vi "myRIO_BRig_RT_v0,41.vi"() -> ()   [LabVIEW 2014]
uses:
  myRIO_BRig_RT__Case_Exp_stateList.ctl
  myRIO_BRig_RT__Case_NonExp_stateList.ctl
  <vilib>/Platform/TimedLoop/XDataNode/timing_clust.ctl
  <vilib>/Platform/TimedLoop/XDataNode/nitl_modes.ctl
  <vilib>/Platform/TimedLoop/XDataNode/wakeup.ctl
  <vilib>/WebDAVClient/Advanced/SessionHandle.ctl
  <vilib>/myRIO/Common/Instrument Driver Framework/myRIO v1.0/UART/vis/myRIO v1.0 Close UART.vi
  <vilib>/FPGAPlugInAG/myRIO-1900/niLvFpga_Open_myRIO-1900.vi
  <vilib>/rvi/interface/common/dynamic/niFpgaDynamicAddResources.vi
  <vilib>/Utility/error.llb/Error Cluster From Error Code.vi
  <vilib>/rvi/errors/niLvFpgaAdjustHostInterfaceError.vi
  <vilib>/FPGAPlugInAG/Dynamic/niLvFpga_Close_Dynamic.vi
  <vilib>/myRIO/Common/Instrument Driver Framework/Utilities/vis/FPGA Ref Manager.vi
  <vilib>/myRIO/Common/Instrument Driver Framework/myRIO v1.0/myRIO v1.0 Reset FPGA.vi
  <vilib>/myRIO/Common/Instrument Driver Framework/myRIO v1.0/IRQ/vis/myRIO v1.0 IRQ Info FGV.vi
  <vilib>/myRIO/Common/Instrument Driver Framework/myRIO v1.0/IRQ/vis/myRIO v1.0 Timer IRQ Info FGV.vi
  <vilib>/myRIO/Common/Instrument Driver Framework/myRIO v1.0/IRQ/vis/myRIO v1.0 ISR Agent.vi
  <vilib>/rvi/interface/nirviOpenFPGA/nirviOpenFPGA.xnode
  myRIO_BRig_FPGA_v3,2__PortC__build.lvbitx
  myRIO_BRig_FPGA_v3,2__PortC.vi
  <vilib>/rvi/interface/nirviReadWriteControl/nirviReadWriteControl.xnode
  <vilib>/Platform/TimedLoop/XDataNode/XDataNode.xnode
  <vilib>/rvi/interface/nirviCloseFPGA/nirviCloseFPGA.xnode
  <vilib>/Platform/TimedLoop/XDataNode/XDNodeRunTimeDep.lvlib
  <vilib>/rvi/interface/Simulation/niFpgaSimulationCallBeginRW.vi
  <vilib>/myRIO/Instrument Drivers/Utilities/Utilities.lvlib
  <vilib>/WebDAVClient/NI_WebDAV.lvlib
  NiFpgaLv.dll
panel:
  in  "AO0":i16 min=-2047 max=2047 step=1
  in  "laser_Nvalley":u32
  in  "laser_Npeak":u32
  in  "LC_Cue1_All_Count":u16
  in  "LC_Cue1_First_Count":u16
  in  "LC_Cue1_All_delayOpt":bool
  in  "LC_ENL1_All_delayOpt":bool
  in  "LC_ENL1_All_Count":u16
  in  "LC_ENL1_First_Count":u16
  in  "LC_Cue1_First_delayOpt":bool
  in  "LC_ENL1_First_delayOpt":bool
  in  "Tcycle_Cue_max":u16=1000 caption="Max [ms]" min=5 max=5000 step=5
  in  "Tcycle_Cue_min":u16=1000 caption="Min [ms]" min=5 max=5000 step=5
  in  "SendData":bool
  out "cSpout":enum16{"Left", "Right"}(ring) caption="Left or Right Spout"
  out "A4":u32 caption="LickCounter_Right"
  out "A2":u32 caption="LickCounter_Left"
  in  "tDelay_laser_wro":u32
  in  "tCycle_laser_wro":u32=1000
  in  "tDelay_laser_rew":u32
  in  "laserResponse_wrong_LED":bool
  out "error_initTrial":errorcluster
  out "error_Selection_pre":errorcluster
  out "error_Selection":errorcluster
  in  "tCycle_laser_rew":u32=1000
  out "SelectWrong":bool
  out "SelectReward":bool
  in  "Left(F)_or_Right(T)":bool
  in  "ignoreWrong":bool
  in  "SelectionState":bool
  in  "laserResponse_wrong":bool
  in  "laserResponse_reward":bool
  in  "laserResponse_reward_LED":bool
  out "nRewards_Right":u16 caption="# Rewards Total (Right)"
  out "nRewards_Left":u16 caption="# Rewards Total (Left)"
  out "nRewards_cur":u16 caption="# Rewards in Current Block"
  out "TpB_target":u16 caption="Target Trials Per Block"
  out "cState_NonExp":T1 caption="NonExperimental State"
  out "iBlock":u16 caption="Current Block"
  out "cState":T2 caption="Experimental State"
  out "iTrial":u16 caption="Current Trial"
  in  "warmupType":bool
  in  "TestConnection":bool
  in  "warmup":bool caption="WarmUp"
  in  "Host Filename Prefix":string="Exp1_TM2"
  out "Connected To Host?":bool
  in  "Host Password":string="sabalab"
  in  "Host UserName":string="Test2"
  in  "sp_RightSpout":u16(slide)=2 max=2 step=1 scale=0.0..2.0
  in  "sp_LeftSpout":u16(slide)=2 max=2 step=1 scale=0.0..2.0
  in  "BUR_max":u16 caption="Count Reward Structure  (0 = off)"
  in  "LC_Wrong_Probability":u16
  in  "LC_Wrong_Trial":u16(slide) max=2 step=1 scale=0.0..2.0
  in  "LC_Wrong_Block":u16(slide) max=2 step=1 scale=0.0..2.0
  in  "LC_Wrong_OnOff":bool
  in  "LC_Reward_Probability":u16
  in  "LC_Reward_Trial":u16(slide) max=2 step=1 scale=0.0..2.0
  in  "LC_Reward_Block":u16(slide) max=2 step=1 scale=0.0..2.0
  in  "LC_Reward_OnOff":bool
  in  "LC_Cue1_All_Probability":u16
  in  "LC_Cue1_All_Block":u16(slide) max=2 step=1 scale=0.0..2.0
  in  "LC_Cue1_All_OnOff":bool
  in  "LC_Cue1_First_Probability":u16
  in  "LC_Cue1_First_Block":u16(slide) max=2 step=1 scale=0.0..2.0
  in  "LC_Cue1_First_OnOff":bool
  in  "LC_ENL1_All_Probability":u16 max=100 step=1
  in  "LC_ENL1_All_Block":u16(slide) max=2 step=1 scale=0.0..2.0
  in  "LC_ENL1_All_OnOff":bool
  in  "LC_ENL1_First_Probability":u16 max=100 step=1
  in  "LC_ENL1_First_Block":u16(slide) max=2 step=1 scale=0.0..2.0
  in  "A6":bool caption="Activate Recording?\n(Select Prior to\nStarting Experiment)"
  in  "Tcycle_Timeout":u16=1000 caption="Timeout Time [ms]" min=10 max=10000 step=1
  in  "Tcycle_Wrong":u16=1000 caption="Wrong Time [ms]" min=10 max=10000 step=1
  in  "Tcycle_Selection":u16=1000 caption="Answer Time [ms]" min=1 max=10000 step=1
  in  "Tcycle_RewardPost":u16=1000 caption="Consumption Time [ms]" min=250 max=10000 step=250
  in  "Tcycle_Reward_L":u16=500 caption="Reward Time [ms]" min=1 max=1000 step=1
  in  "Tcycle_Reward_R":u16=500 caption="Reward Time [ms]" min=1 max=1000 step=1
  in  "TpB_Max_R":u16=4 caption="Max TrialsPerBlock" min=1 max=12 step=1
  in  "TpB_Min_R":u16=4 caption="Min TrialsPerBlock" min=1 max=12 step=1
  in  "TpB_Max_L":u16=4 caption="Max TrialsPerBlock" min=1 max=12 step=1
  in  "TpB_Min_L":u16=4 caption="Min TrialsPerBlock" min=1 max=12 step=1
  in  "BUR_min":u16 caption="Count Reward Structure  (0 = off)"
  in  "TrialUntilReward":bool caption="Ignore Wrong \nSelection"
  in  "CueCycles":u16=1 caption="Cue Structure" min=1 max=1 step=1
  in  "MTrig_Laser_Tcycle":u16=10 caption="Time [ms]"
  in  "MTrig_Laser_trig":bool
  in  "MTrig_Audio_trig__R":bool caption="Trigger Audio"
  in  "MTrig_Audio_trig__L":bool caption="Trigger Audio"
  in  "RewCalib_Trig_R":bool caption="Calibrate_R"
  in  "RewCalib_Trig_L":bool caption="Calibrate_L"
  in  "MTrig_Solenoid_Tcycle__R":u16=300 caption="Time [ms]"
  in  "MTrig_Solenoid_Tcycle__L":u16=300 caption="Time [ms]"
  in  "MTrig_Solenoid_trig__R":bool caption="Solenoid"
  in  "MTrig_Solenoid_trig__L":bool caption="Solenoid"
  in  "STOP_abort":bool caption="Stop LabView\n(Stops myRio and FPGA)"
  in  "STOP_endBlock":bool caption="Stop Experiment\n@ End of Block"
  in  "STOP_endTrial":bool caption="Stop Experiment\n@ End of Trial"
  in  "START":bool caption="Start Experiment"
  in  "Tcycle_CuePenalty":u16=1000 caption="Penalty [ms]" min=1 max=10000 step=1
  in  "Audio_Amp__R":u16=100 caption="Amp"
  in  "Audio_Freq__R":u16=5 caption="Freq [kHz]" max=14 step=1
  in  "Audio_Amp__L":u16=100 caption="Amp"
  in  "Audio_Freq__L":u16=5 caption="Freq [kHz]" max=14 step=1
  in  "LC_Wrong_Tdelay":u16
  in  "LC_Cue1_All_Tdelay":u16
  in  "LC_ENL1_All_Tdelay":u16
  in  "LC_Reward_Tdelay":u16
  in  "LC_Cue1_First_Tdelay":u16
  in  "LC_ENL1_First_Tdelay":u16
  in  "LC_ENL1_First_OnOff":bool
  in  "Tcycle_ENLPenalty":u16=100 caption="Penalty [ms]" min=10 max=100 step=10
  in  "Tcycle_ENL_max":u16=1000 caption="Max [ms]" min=250 max=10000 step=250
  in  "Tcycle_ENL_min":u16=1000 caption="Min [ms]" min=250 max=10000 step=250
  # "Manual Control"
  # "Task Structure"
  # "Task Timing"
  # "Laser Control    [10ms pulse]\n\n                                                    On/Off      Block        Probability [%]   Delay [ms]                              Count"
  # "Manual Solenoid Trigger\nLeft              Right"
  # "Master Structure"
  # "Enforced NonLick"
  # "Enforced NonLick 1"
  # "from end"
  # "Time = Cue Min"
  # "Min\n \n  \nMax"
  # "First Trial"
  # "from start"
  # "(1) = Switching\n(2) = Two Choice"
  # "from end"
  # "All Trials"
  # "Cue"
  # "from start"
  # "Cue 1"
  # "from end"
  # "from start"
  # "Cue then reward"
  # "Min"
  # "Max"
  # "from end"
  # "Cue with reward"
  # "Trial Per Block Structure\n       Left                    Right"
  # "from start"
  # "Spout Selection Control"
  # "Manual Speaker Trigger\nLeft              Right"
  # "Selection Reward"
  # "Answer Time\n         [ms]\n\n  \nWrong Choice Penalty\n         [ms]\n \n \nChoice Timeout Penalty\n         [ms]"
  # "Selection Wrong"
  # "Cue Control"
  # "Left              Right"
  # "State"
  # "Manual Laser Trigger"
  # "Freq [kHz]\n \n \nAmp\n \n\n \n\nSpeaker\nSetting"
  # "Reward Control\n                 Left              Right"
  # "Min = 1\nMax = 32k"
  # "Reward Time\n         [ms]"
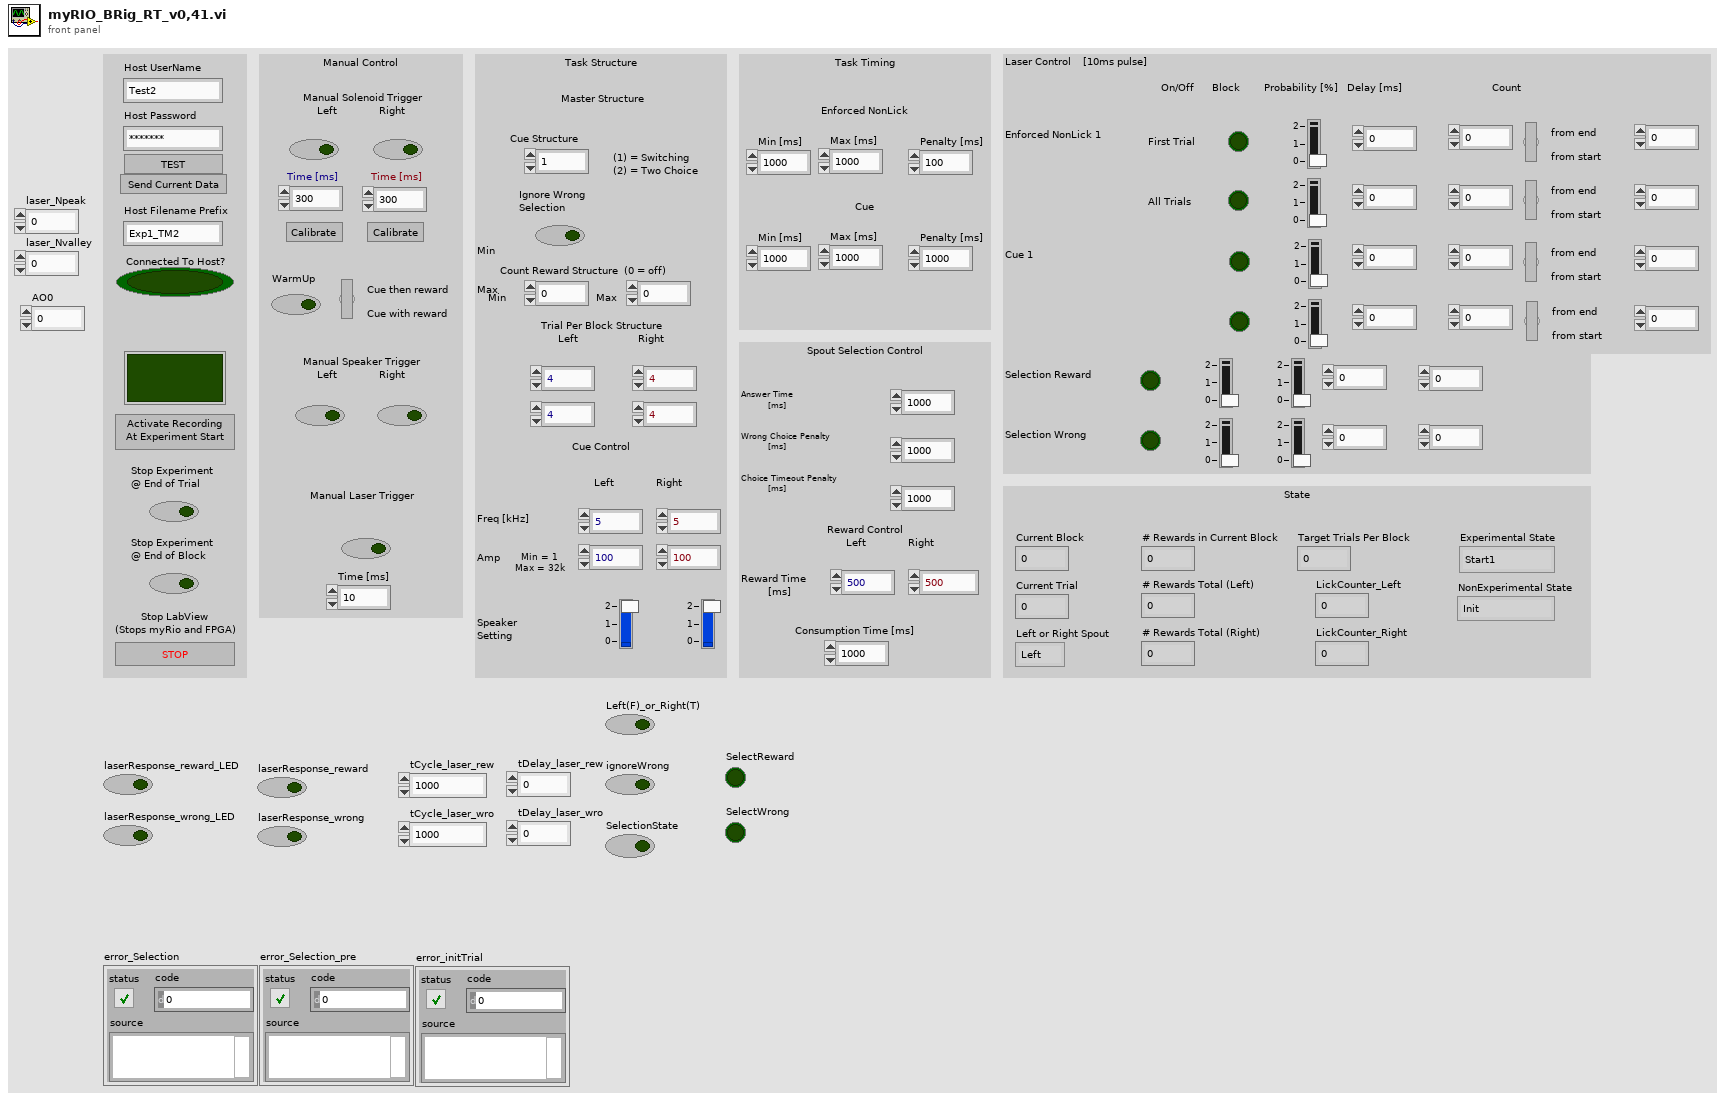
[diagram p1: front panel]
types:
  T1 = typedef "myRIO_BRig_RT__Case_NonExp_stateList.ctl" = enum16{"Init", "UploadSettings_pre", "UploadSettings_Read_dataExp", "UploadSettings_dataExp_1", "UploadSettings_Read_dataLC", "UploadSettings_dataLC_1", "UploadSettings_dataLC_2", "UploadSettings_Read_dataMTrig", "UploadSettings_dataMTrig_1", "UploadSettings_post", "Idle_pre", "IdleEmpty", "IdleEmpty2", "IdleEmpty3", "IdleEmpty4", "Idle", "Idle_2", "Idle_3", "Idle_4", "Idle_post", "Cue_pre__pre", "Cue_pre", "Cue", "Cue_post", "RewardCalibration_pre", "DispenseWater_pre__pre", "DispenseWater_pre", "DispenseWater", "DispenseWater_post", "TestConnection", "SendData", "End"}
  T2 = typedef "myRIO_BRig_RT__Case_Exp_stateList.ctl" = enum16{"Start1", "Start2", "Start3", "saveSettings1", "saveSettings2", "saveSettings3", "saveSettings4_LC_ENL", "saveSettings5_LC_Cue", "saveSettings6_LC_Other", "setSettings_Audio", "setSettings_Laser", "initBlock_pre", "initBlock", "initBlock2", "initBlock_post", "initTrial_pre", "initTrial", "initTrial2", "initTrial3", "initTrial4", "initTrial_LC_ENL1", "initTrial_LC_Cue1", "initTrial_post", "ENL1_pre", "ENL1", "ENL1_post", "ENL1Penalty_pre", "ENL1Penalty", "ENL2_pre", "ENL2", "ENL2Penalty_pre", "ENL2Penalty", "Cue1_pre", "Cue1", "Cue1_post", "Cue1Penalty_pre", "Cue1Penalty", "Cue2_pre", "Cue2", "Cue2Penalty_pre", "Cue2Penalty", "Selection_pre", "Selection", "Select_post", "SelectReward_pre", "SelectReward", "SelectRewardPost_pre", "SelectRewardPost", "SelectWrong_pre", "SelectWrong", "SelectWrong_post", "SelectTimeout_pre", "SelectTimeout", "SelectTimeout_post", "endTrial_pre", "endTrial1", "endTrial2", "endTrial3", "endTrial_post", "endBlock_pre", "endBlock", "endBlock_post", "endExp", "commConnect", "commUpload_pre", "commUpload_dataBlock", "commUpload_dataCurrent", "commUpload_dataExp", "commUpload_dataLC", "commUpload_dataTrial", "commUpload_post", "saveData_pre", "saveData_dataBlock", "saveData_dataCurrent", "saveData_dataExp", "saveData_dataLC", "saveData_dataTrial", "saveData_post"}
  T3 = typedef "XDNodeRunTimeDep.lvlib/timing_clust.ctl" = cluster{"Expected End [f-1]":u64, "Actual End [f-1]":u64, "Finished Late? [f-1]":bool, "Expected End [i-1]":u64, "Actual End [i-1]":u64, "Finished Late? [i-1]":bool, "Expected Start [i]":u64, "Actual Start [i]":u64, "Expected Start [f]":u64, "Actual Start [f]":u64, "Source Name":string, "Structure Name":string, "Period":i64, "Deadline":i64, "Offset":i64, "Start":i64, "Priority":i32, "Timeout":i32, "Mode":T4, "Wakeup Reason":T5, "Error":errorcluster, "Source Type":string, "Secondary Source Type":string, "Global End Time":u64, "Global Start Time":u64, "Frame Duration":u64, "Iteration Duration":u64, "Assigned CPU":i32, "I/O Scan Engine Mode":u32}
  T4 = typedef "XDNodeRunTimeDep.lvlib/nitl_modes.ctl" = enum32{"No Change", "Process missed periods, maintain original phase", "Discard missed periods, maintain original phase", "Process missed periods, ignore original phase", "Discard missed periods, ignore original phase"}
  T5 = typedef "XDNodeRunTimeDep.lvlib/wakeup.ctl" = enum32{"Normal", "Aborted", "Asynchronous wakeup", "Timing source error", "Timed loop error", "Timeout"}
  T6 = typedef "NI_WebDAV.lvlib/SessionHandle.ctl" = refnum<k1>
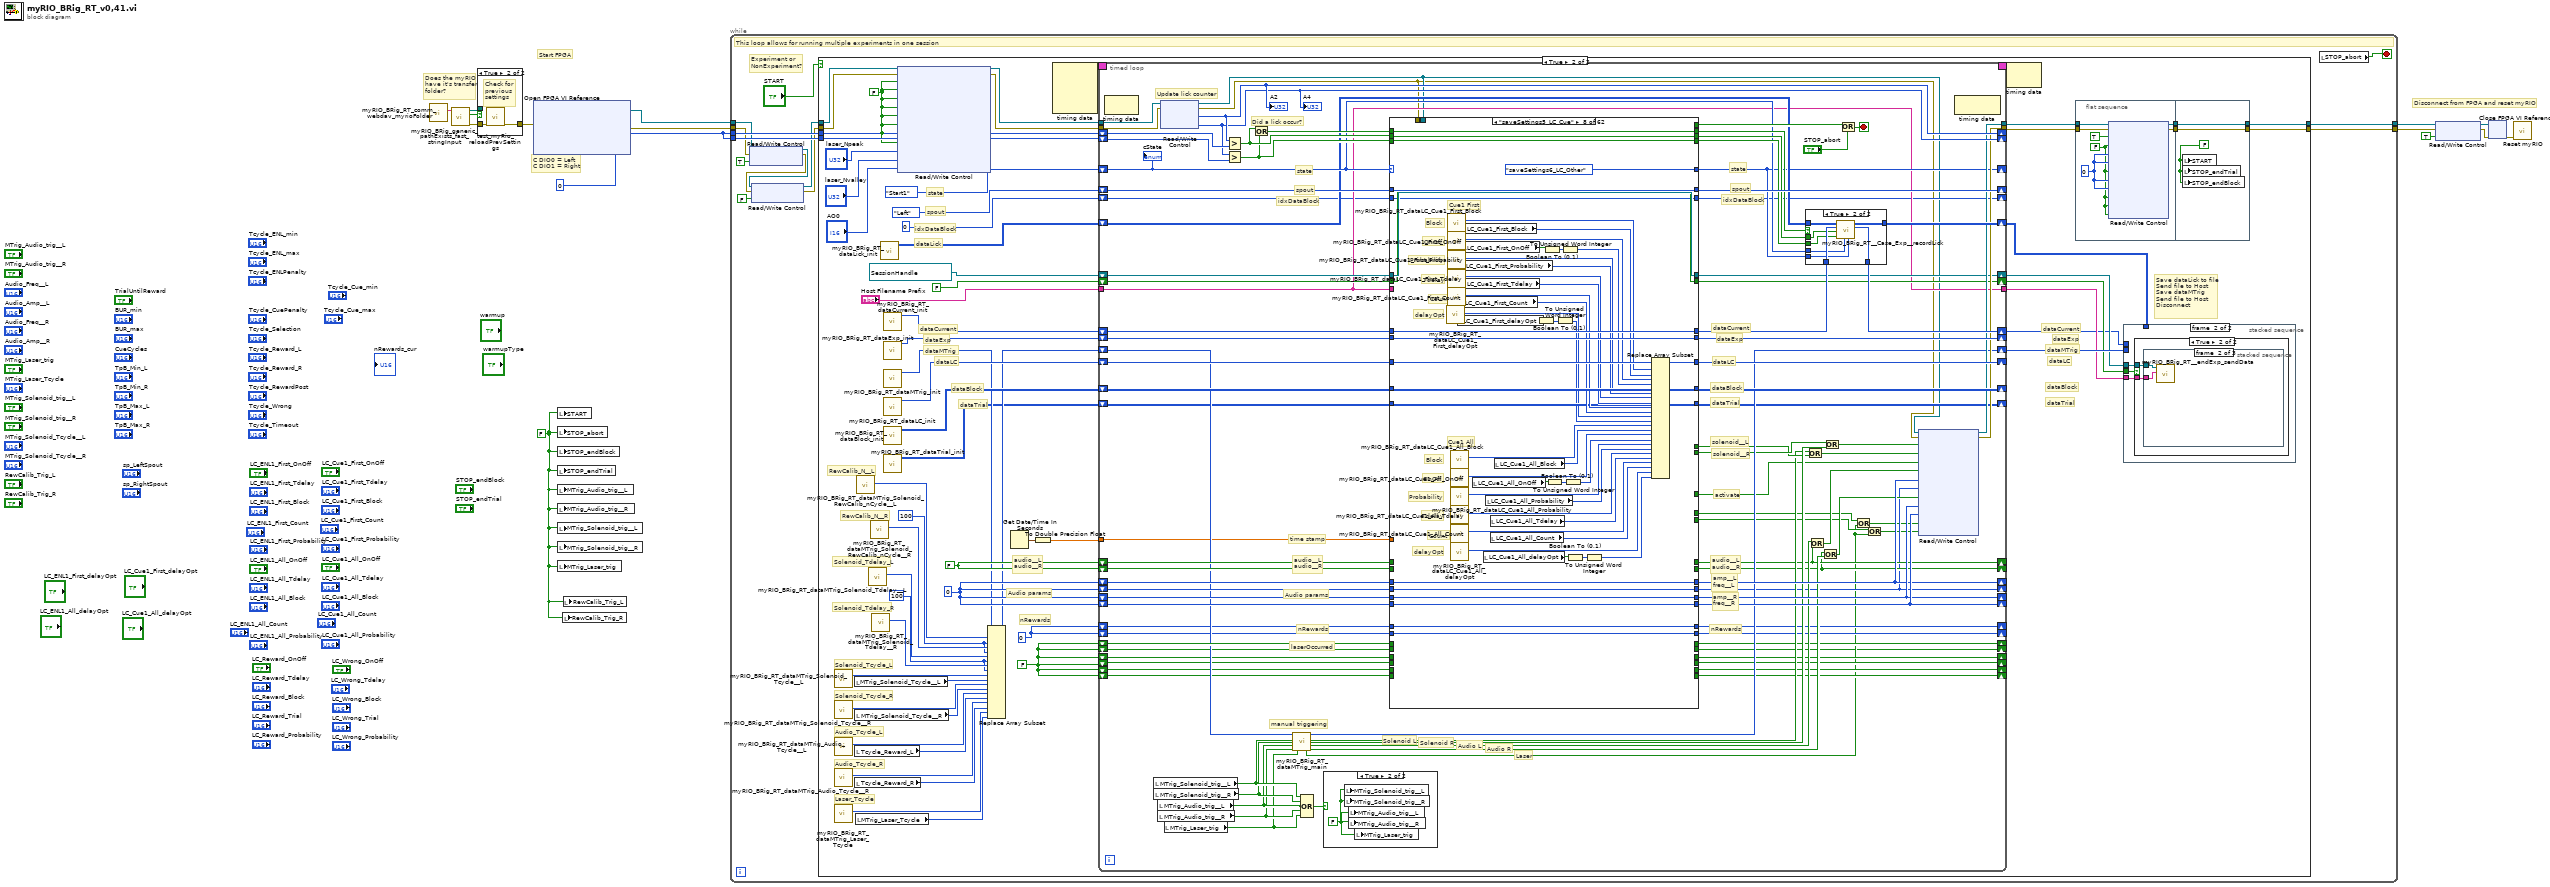
[diagram p0: block diagram]
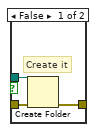
[diagram p2: hidden frame]
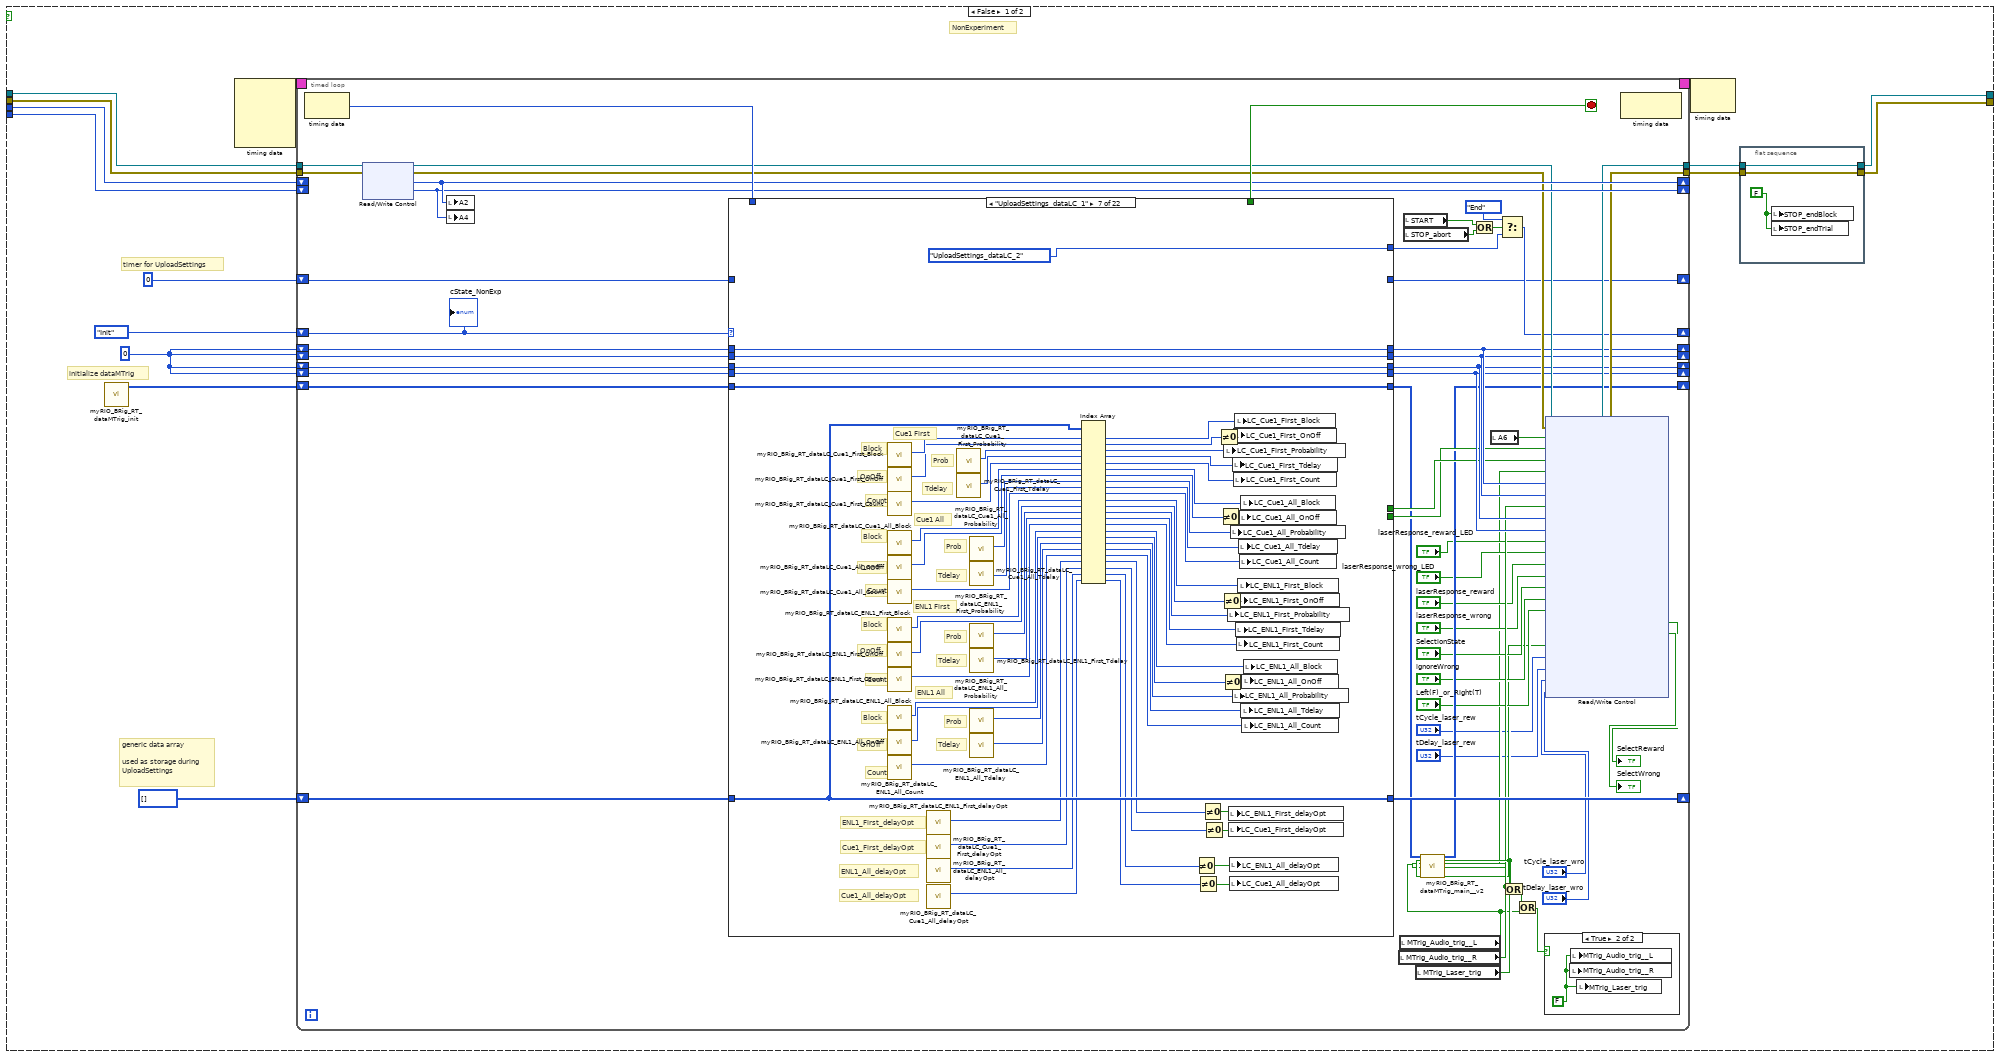
[diagram p3: hidden frame]
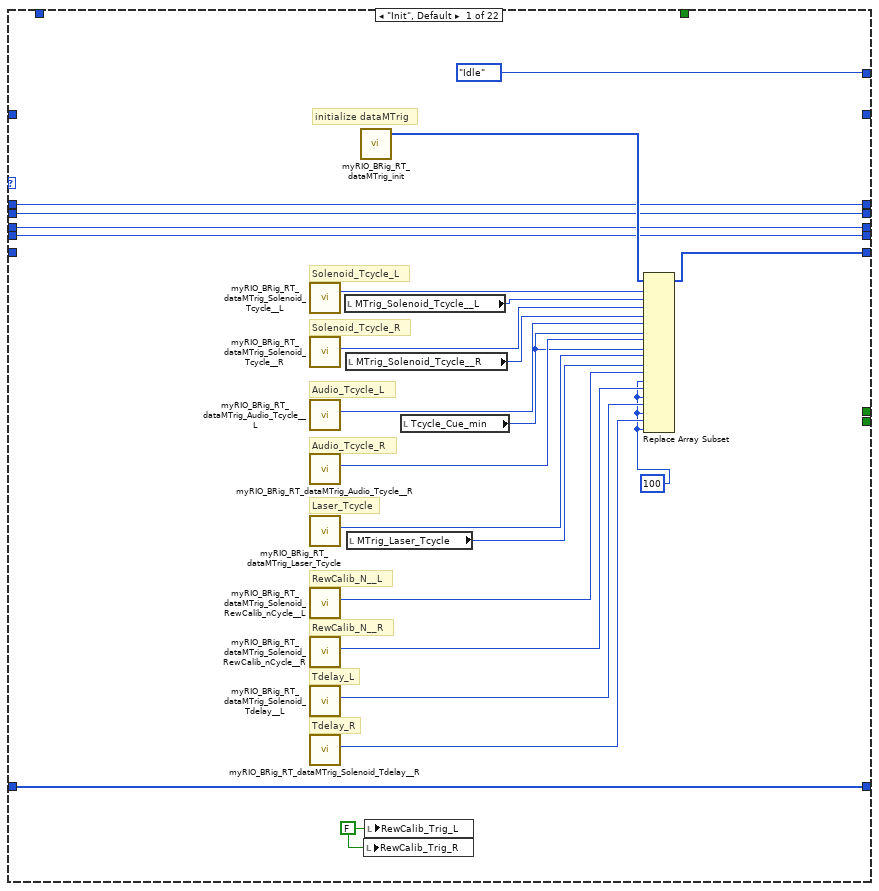
[diagram p5: hidden frame]
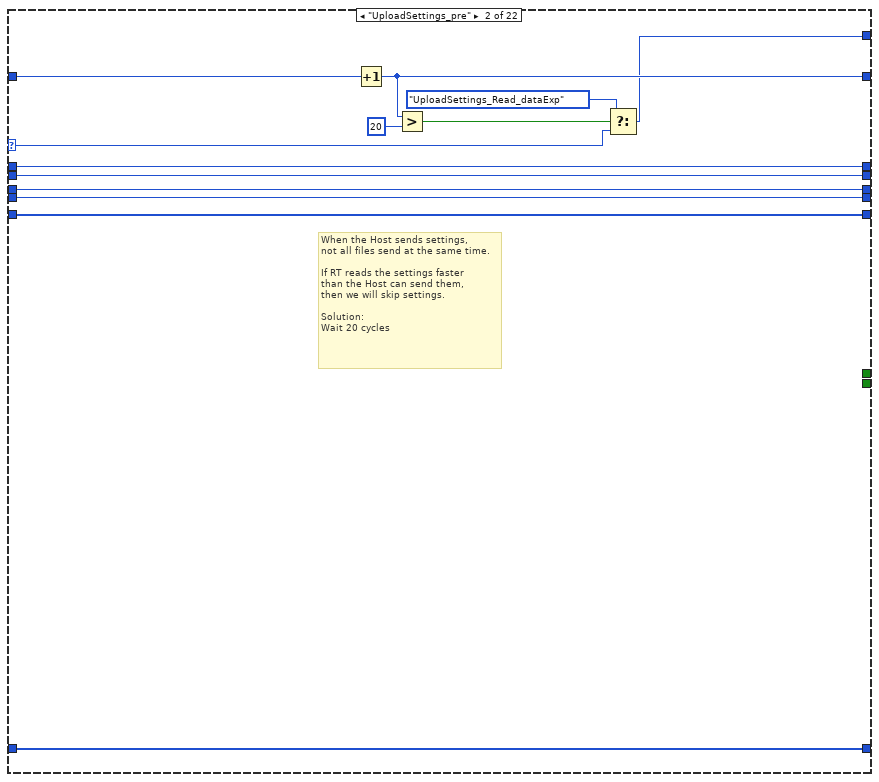
[diagram p6: hidden frame]
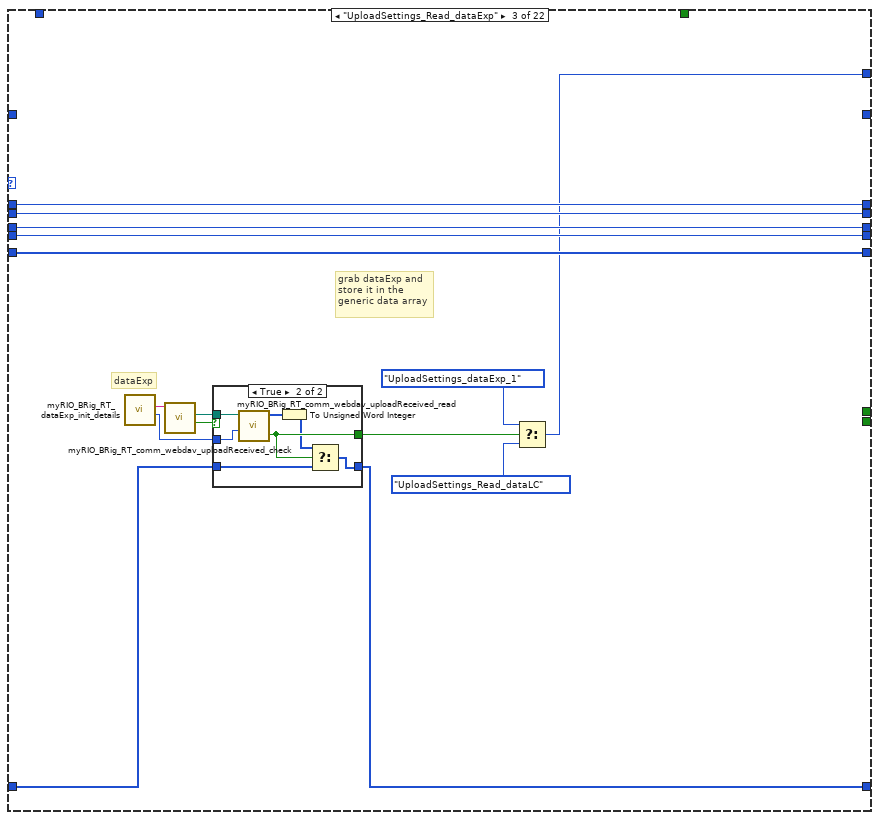
[diagram p7: hidden frame]
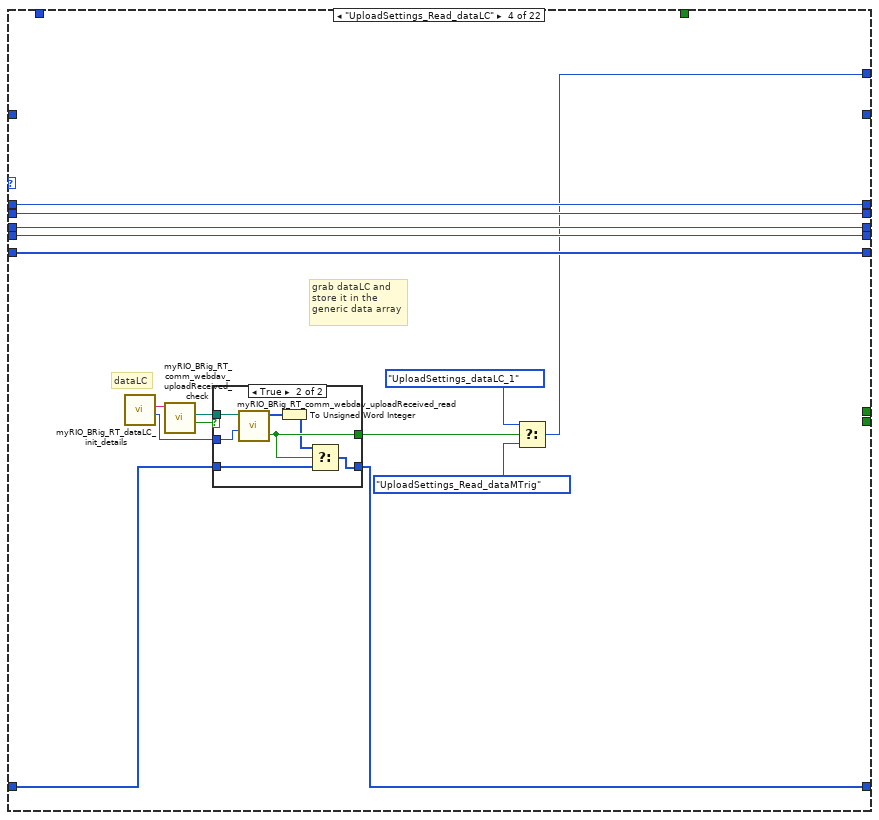
[diagram p9: hidden frame]
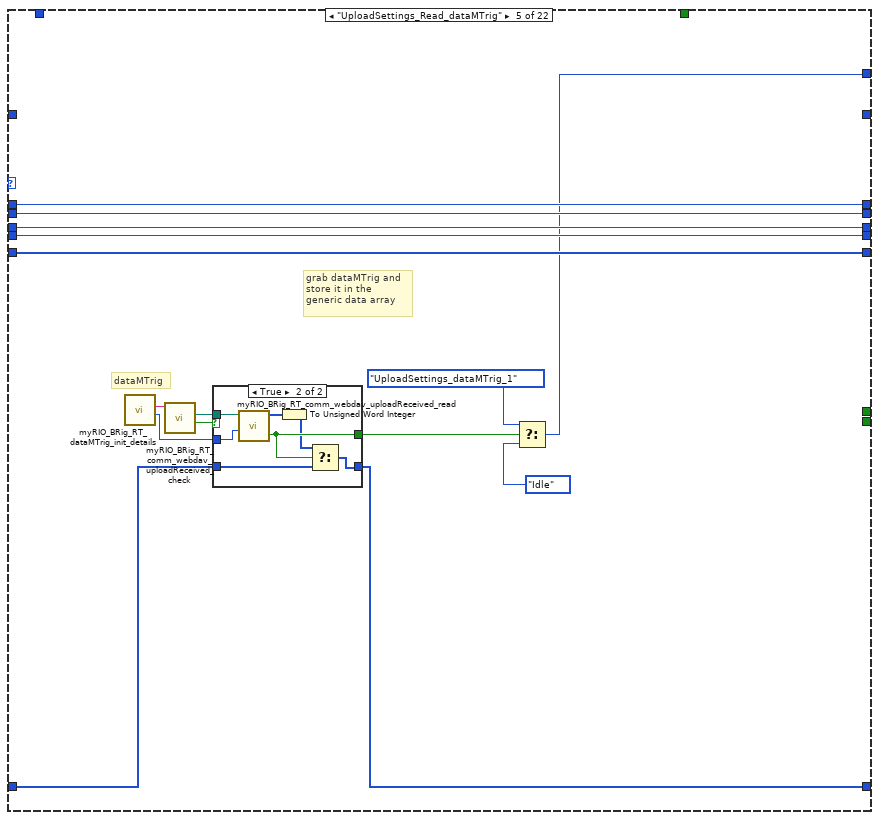
[diagram p11: hidden frame]
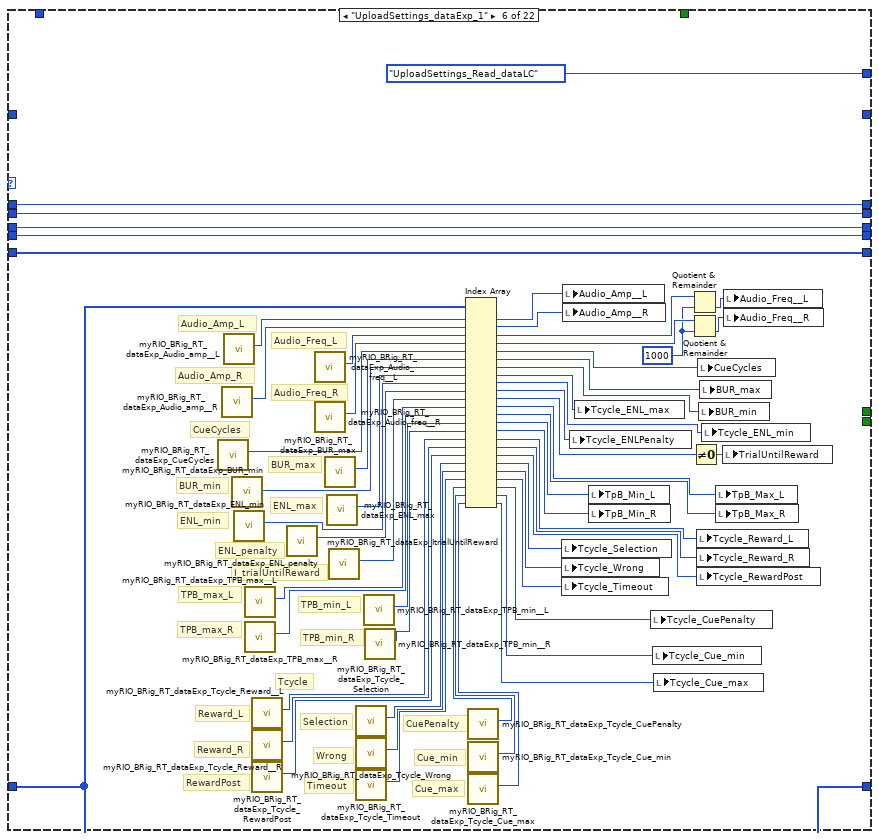
[diagram p13: hidden frame]
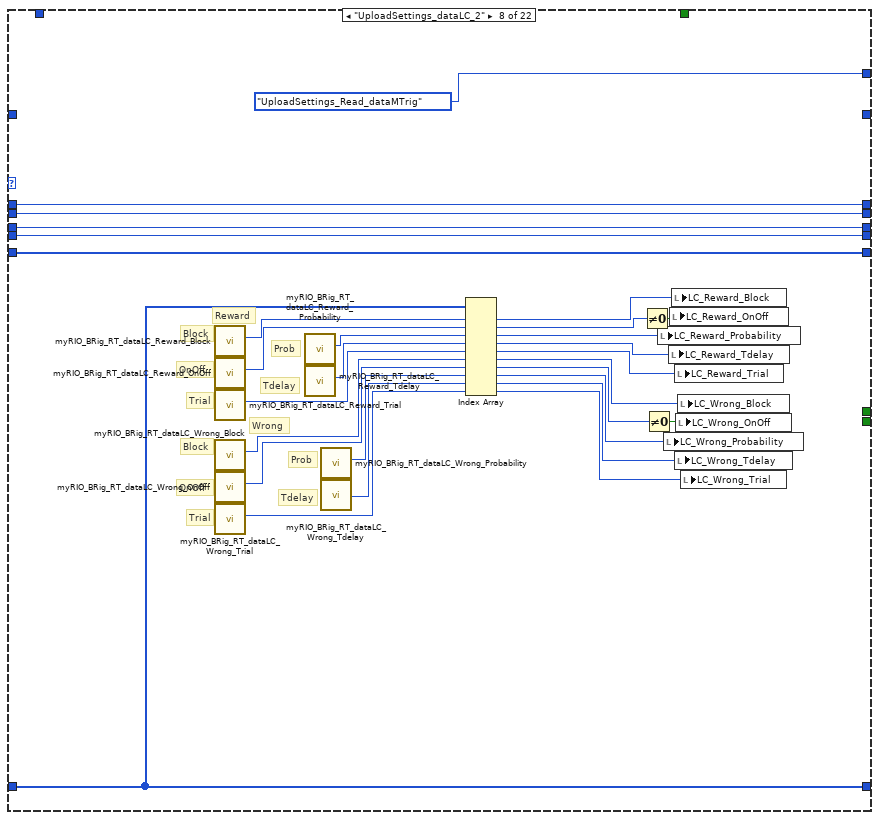
[diagram p14: hidden frame]
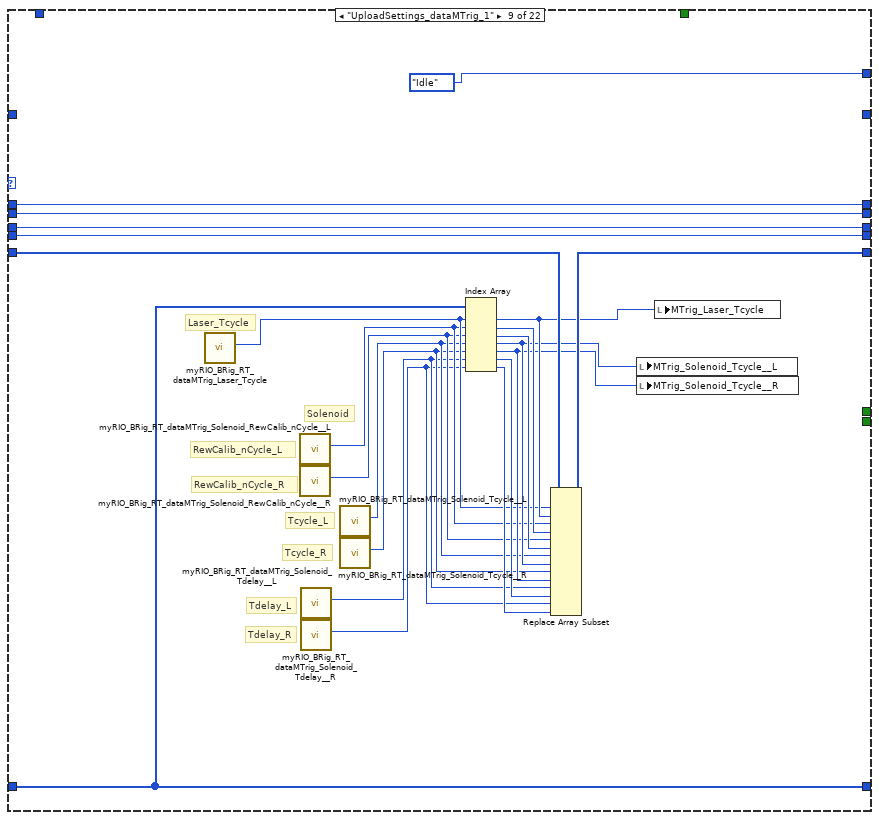
[diagram p15: hidden frame]
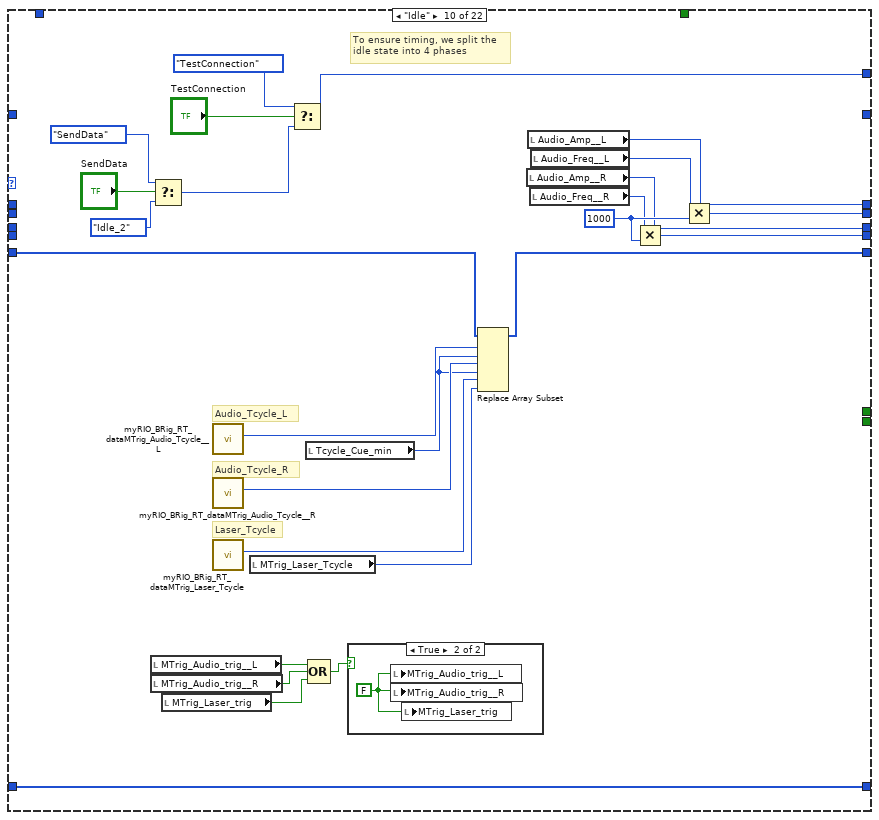
[diagram p16: hidden frame]
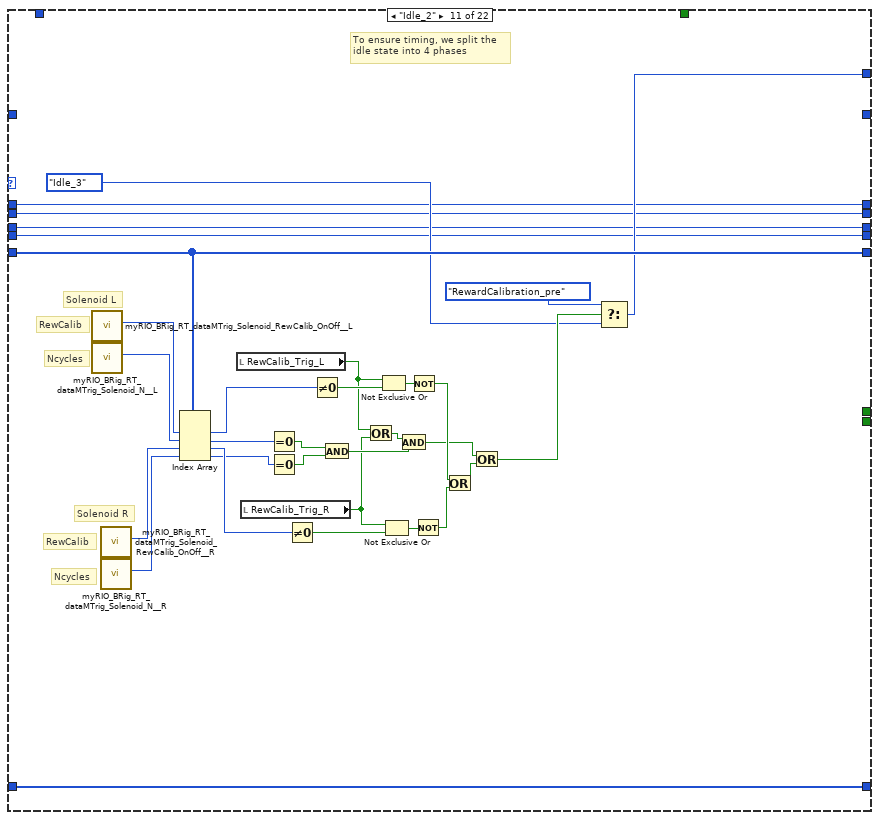
[diagram p18: hidden frame]
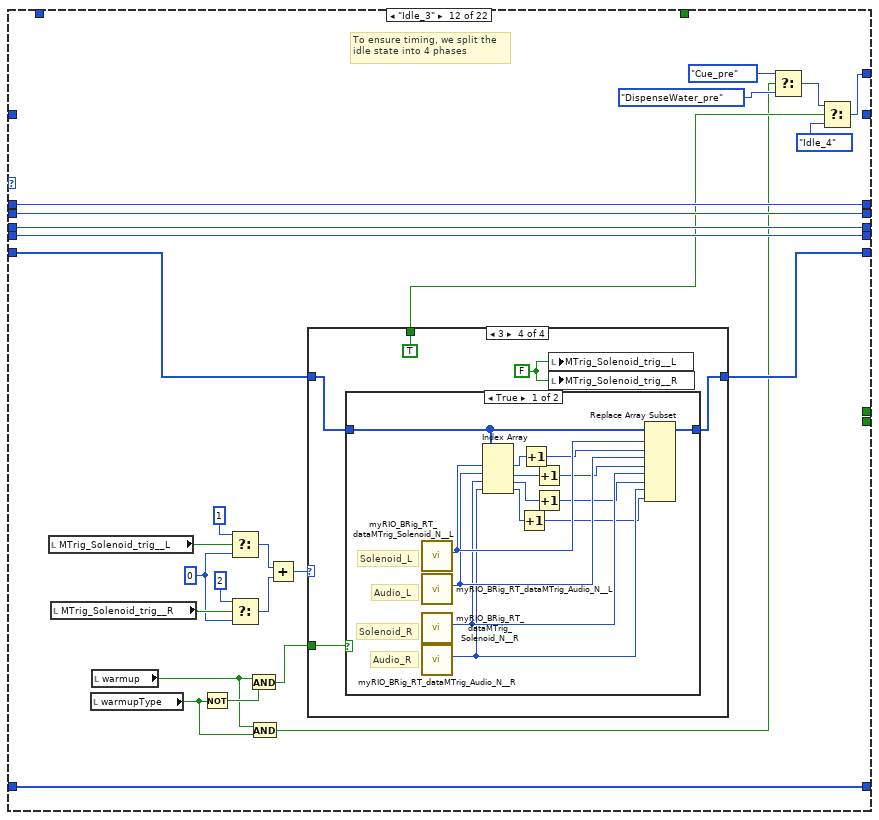
[diagram p19: hidden frame]
diagram:
  w9 = u32 0
  w6 = FALSE
  # "Does the myRIO\nhave it's transfer\nfolder?"
  # "C DIO0 = Left\nC DIO1 = Right"
  # "Start FPGA"
  # "Disconnect from FPGA and reset myRIO"
  n1 = call "myRIO_BRig_RT_comm_webdav_myrioFolder.vi"() -> ("output_myrioFolder"=w4:string)  [unwired: 11 in]
  n2 = call "myRIO_BRig_generic_pathExists_fast_stringInput.vi"("input_filePath"=w4) -> ("output_error"=w3:errorcluster, "output_Iexist"=w2:bool, "output_filePath"=w1:path)  [unwired: 8 in]
  n3 = case shown="True" w2 {
    tunnel: w1 -> [w18 _]
    tunnel: w3 -> [w17 w20]
    tunnel: [w16 w19] -> w5
    frame False {
      # "Create it"
      n4 = Create Folder(path (use dialog)=w18, error in=w17) -> (error out=w16:errorcluster)  [unwired: 1 in, 2 out]
    }
    frame True {
      # "Check for\nprevious\nsettings"
      n5 = call "test_myRio_reloadPrevSettings.vi"("input_error"=w20) -> ("output_error"=w19:errorcluster)  [unwired: 10 in]
    }
  }
  n6 = xnode "Open FPGA VI Reference"("error in"=w5) -> ("FPGA VI Reference Out"=w11:refnum<k20>, "error out"=w10:errorcluster)  [unwired: 1 in]
  n7 = local write "START"(w6) -> ()
  n8 = local write "STOP_abort"(w6) -> ()
  n9 = local write "STOP_endBlock"(w6) -> ()
  n10 = local write "STOP_endTrial"(w6) -> ()
  n11 = local write "MTrig_Audio_trig__L"(w6) -> ()
  n12 = local write "MTrig_Audio_trig__R"(w6) -> ()
  n13 = local write "MTrig_Solenoid_trig__L"(w6) -> ()
  n14 = local write "MTrig_Solenoid_trig__R"(w6) -> ()
  n15 = local write "MTrig_Laser_trig"(w6) -> ()
  n16 = local write "RewCalib_Trig_R"(w6) -> ()
  n17 = local write "RewCalib_Trig_L"(w6) -> ()
  n18 = while {
    tunnel: w11 -> [w24]
    tunnel: w10 -> [w29]
    tunnel: w9 -> [w32]
    tunnel: w9 -> [w31]
    tunnel: [w22] -> w8
    tunnel: [w21] -> w7
    stop <- w30 stop-if-true
    # "Experiment or\nNonExperiment?"
    # "This loop allows for running multiple experiments in one session"
    n19 = xnode "Read/Write Control"("FPGA VI Reference In"=w24, "error in"=w29, "Counts_Reset"=TRUE) -> ("FPGA VI Reference Out"=w26:refnum<k20>, "error out"=w27:errorcluster)
    n20 = xnode "Read/Write Control"("FPGA VI Reference In"=w26, "error in"=w27, "Counts_Reset"=FALSE) -> ("FPGA VI Reference Out"=w23:refnum<k20>, "error out"=w25:errorcluster)
    n21 = case shown="True" "START" {
      tunnel: w32 -> [w45 w917]
      tunnel: w31 -> [w44 w916]
      tunnel: w25 -> [w42 w867]
      tunnel: w23 -> [w43 w866]
      tunnel: [w40 w913] -> w22
      tunnel: [w38 w908] -> w21
      frame False {
        w37 = u16 0 ("Audio_Amp__L")
        # "generic data array\n\nused as storage during\nUploadSettings"
        # "timer for UploadSettings"
        # "initialize dataMTrig"
        # "NonExperiment"
        n22 = call "myRIO_BRig_RT_dataMTrig_init.vi"() -> ("output_dataMTrig"=w46:u16[])  [unwired: 5 in]
        n23 = node-c288() -> (w49:T3)  [unwired: 4 in]
        n24 = timed-loop {
          timing: w49 -> [_]
          timing-out: [_] -> w48
          shift-right: [w83] -> _
          shift-left: w46 -> [w107]
          shift-right: [w72] -> _
          shift-left: myRIO_BRig_RT__Case_NonExp_stateList."Init" ("Enum") -> [w97]
          shift-right: [w105] -> _
          shift-left: w45 -> [_]
          shift-right: [w104] -> _
          shift-left: w44 -> [_]
          tunnel: [w100] -> w41
          tunnel: [w98] -> w39
          tunnel: w42 -> [w103]
          tunnel: w43 -> [w102]
          shift-right: [w96] -> _
          shift-left: u16[] [] ("output_data") -> [w95]
          shift-right: [w90] -> _
          shift-left: w37 -> [w94]
          shift-right: [w89] -> _
          shift-left: w37 -> [w93]
          shift-right: [w88] -> _
          shift-left: w37 -> [w92]
          shift-right: [w87] -> _
          shift-left: w37 -> [w91]
          shift-right: [w54] -> _
          shift-left: u16 0 ("Audio_Amp__L") -> [w55]
          stop <- w108 stop-if-true
          n25 = node-c288() -> (w106:i64)  [unwired: 1 in]
          n26 = xnode "Read/Write Control"("FPGA VI Reference In"=w102, "error in"=w103) -> ("FPGA VI Reference Out"=w101:refnum<k20>, "error out"=w99:errorcluster, "A2_LickL"=w105:u32, "A4_LickR"=w104:u32)
          n27 = local write "A2"(w105) -> ()
          n28 = local write "A4"(w104) -> ()
          n29 = case shown="\"UploadSettings_dataLC_1\"" w97 {
            selector: w97 -> [_ w141 _ _ _ _ _ _ _ _ _ _ _ _ w573 _ _ w758 _ _ _ w855]
            tunnel: [myRIO_BRig_RT__Case_NonExp_stateList."Idle" ("Enum") w139 w146 w169 w192 myRIO_BRig_RT__Case_NonExp_stateList."UploadSettings_Read_dataLC" ("Enum") myRIO_BRig_RT__Case_NonExp_stateList."UploadSettings_dataLC_2" ("Enum") myRIO_BRig_RT__Case_NonExp_stateList."UploadSettings_Read_dataMTrig" ("f") myRIO_BRig_RT__Case_NonExp_stateList."Idle" ("Enum") w399 w420 w453 w544 myRIO_BRig_RT__Case_NonExp_stateList."Cue" ("t") w572 myRIO_BRig_RT__Case_NonExp_stateList."DispenseWater_pre" ("Enum") w700 w756 w783 myRIO_BRig_RT__Case_NonExp_stateList."Idle" ("Enum") myRIO_BRig_RT__Case_NonExp_stateList."Idle" ("Enum") w855] -> w73
            tunnel: [w124 w134 w156 w179 w202 w273 w336 w365 w385 w410 w435 w464 w542 w560 w586 w610 w737 w763 w794 w837 w847 w853] -> w84
            tunnel: [_ _ _ _ _ _ _ _ _ _ _ _ _ _ _ _ _ _ _ _ _ TRUE] -> w108
            tunnel: w107 -> [_ w134 w156 w179 w202 w273 w336 w365 w386 w409 w435 w465 w542 w561 w586 w596 w733 w764 w795 w837 w847 w853]
            tunnel: w106 -> [_ _ _ _ _ _ _ _ _ _ _ _ _ _ _ _ _ w768 _ _ _ _]
            tunnel: [w113 w133 w147 w170 w193 w217 w288 w337 w366 w394 w415 w447 w537 w548 w571 w587 w685 w741 w776 w825 w841 w848] -> w96
            tunnel: w95 -> [w113 w133 w148 w171 w194 w217 w288 w337 w366 w394 w415 w447 w537 w548 w571 w587 w685 w741 w776 w825 w841 w848]
            tunnel: [w117 w137 w159 w182 w205 w270 w334 w340 w383 w405 w418 w457 w539 w568 w583 w590 w739 w774 w801 w828 w844 w851] -> w89
            tunnel: [w115 w135 w157 w180 w203 w268 w332 w338 w381 w404 w416 w459 w541 w566 w585 w588 w738 w772 w799 w826 w842 w849] -> w87
            tunnel: [w118 w138 w160 w183 w206 w271 w335 w341 w384 w403 w419 w456 w538 w570 w582 w591 w740 w775 w802 w829 w845 w852] -> w90
            tunnel: [w116 w136 w158 w181 w204 w269 w333 w339 w382 w402 w417 w458 w540 w567 w584 w589 w738 w773 w800 w827 w843 w850] -> w88
            tunnel: w94 -> [w118 w138 w160 w183 w206 w271 w335 w341 w384 _ w419 w456 w538 w570 w582 w591 w740 w775 w802 w829 w845 w852]
            tunnel: w93 -> [w117 w137 w159 w182 w205 w270 w334 w340 w383 _ w418 w457 w539 w568 w583 w590 w739 w774 w801 w828 w844 w851]
            tunnel: w92 -> [w116 w136 w158 w181 w204 w269 w333 w339 w382 _ w417 w458 w540 w567 w584 w589 w738 w773 w800 w827 w843 w850]
            tunnel: w91 -> [w115 w135 w157 w180 w203 w268 w332 w338 w381 _ w416 w459 w541 w566 w585 w588 _ w772 w799 w826 w842 w849]
            tunnel: [_ _ _ _ _ _ _ _ _ _ _ _ _ _ _ _ _ w765 _ _ _ _] -> w86
            tunnel: [_ _ _ _ _ _ _ _ _ _ _ _ _ _ _ _ _ w747 _ _ _ _] -> w85
            tunnel: w55 -> [_ w145 _ _ _ _ _ _ _ _ _ _ _ _ _ _ _ _ _ _ _ _]
            tunnel: [_ w144 _ _ _ _ _ _ _ _ _ _ _ _ _ _ _ _ _ _ _ _] -> w54
            frame "Init", Default {
              w114 = FALSE ("RewCalib_Trig_L")
              w110 = u16 100 ("new element/subarray")
              # "Tdelay_R"
              # "Tdelay_L"
              # "RewCalib_N__R"
              # "RewCalib_N__L"
              # "Solenoid_Tcycle_R"
              # "Solenoid_Tcycle_L"
              # "Laser_Tcycle"
              # "Audio_Tcycle_R"
              # "Audio_Tcycle_L"
              # "initialize dataMTrig"
              n30 = call "myRIO_BRig_RT_dataMTrig_Solenoid_Tcycle__L.vi"() -> ("output_Solenoid_Tcycle__L"=w126:i32)  [unwired: 11 in]
              n31 = call "myRIO_BRig_RT_dataMTrig_Solenoid_Tcycle__R.vi"() -> ("output_Solenoid_Tcycle__R"=w127:i32)  [unwired: 11 in]
              n32 = call "myRIO_BRig_RT_dataMTrig_Audio_Tcycle__L.vi"() -> ("output_Audio_Tcycle__L"=w128:i32)  [unwired: 11 in]
              n33 = call "myRIO_BRig_RT_dataMTrig_Audio_Tcycle__R.vi"() -> ("output_Audio_Tcycle__R"=w129:i32)  [unwired: 11 in]
              n34 = call "myRIO_BRig_RT_dataMTrig_Laser_Tcycle.vi"() -> ("output_Laser_Tcycle"=w130:i32)  [unwired: 11 in]
              n35 = call "myRIO_BRig_RT_dataMTrig_Solenoid_RewCalib_nCycle__L.vi"() -> ("output_Solenoid_RewCalib_nCycle__L"=w122:i32)  [unwired: 11 in]
              n36 = call "myRIO_BRig_RT_dataMTrig_Solenoid_RewCalib_nCycle__R.vi"() -> ("output_Solenoid_RewCalib_nCycle__R"=w121:i32)  [unwired: 11 in]
              n37 = call "myRIO_BRig_RT_dataMTrig_Solenoid_Tdelay__L.vi"() -> ("output_Solenoid_Tdelay__L"=w120:i32)  [unwired: 11 in]
              n38 = call "myRIO_BRig_RT_dataMTrig_Solenoid_Tdelay__R.vi"() -> ("output_Solenoid_Tdelay__R"=w119:i32)  [unwired: 11 in]
              n39 = local read "MTrig_Solenoid_Tcycle__L"() -> (w131:u16)
              n40 = local read "MTrig_Solenoid_Tcycle__R"() -> (w132:u16)
              n41 = local read "MTrig_Laser_Tcycle"() -> (w111:u16)
              n42 = call "myRIO_BRig_RT_dataMTrig_init.vi"() -> ("output_dataMTrig"=w125:u16[])  [unwired: 5 in]
              n43 = local write "RewCalib_Trig_R"(w114) -> ()
              n44 = local write "RewCalib_Trig_L"(w114) -> ()
              n45 = local read "Tcycle_Cue_min"() -> (w112:u16)
              n46 = Replace Array Subset(array=w125, new element #1=w131, index #1=w126, new element #2=w132, index #2=w127, new element #3=w112, index #3=w128, new element #4=w112, index #4=w129, new element #5=w111, index #5=w130, new element #6=w110, index #6=w122, new element #7=w110, index #7=w121, new element #8=w110, index #8=w120, new element #9=w110, index #9=w119) -> (w124:u16[])
            }
            frame "UploadSettings_pre" {
              # "When the Host sends settings,\nnot all files send at the same time.\n\nIf RT reads the settings faster\nthan the Host can send them,\nthen we will skip settings.\n\nSolution:\nWait 20 cycles"
              n47 = Increment(x=w145) -> (x+1=w144:u16)
              n48 = Greater?(x=w144, y=u16 20) -> (0:w142:bool)
              n49 = Select(t=myRIO_BRig_RT__Case_NonExp_stateList."UploadSettings_Read_dataExp", s=w142, f=w141) -> (s? t:f=w139:T1)
            }
            frame "UploadSettings_Read_dataExp" {
              # "grab dataExp and\nstore it in the\ngeneric data array"
              # "dataExp"
              n50 = call "myRIO_BRig_RT_dataExp_init_details.vi"() -> ("output_dataSize"=w152:i32, "output_dataName"=w155:string)  [unwired: 10 in]
              n51 = call "myRIO_BRig_RT_comm_webdav_uploadReceived_check.vi"("input_dataName"=w155) -> ("output_Iexist"=w154:bool, "output_dataPath"=w153:path)  [unwired: 9 in]
              n52 = case shown="True" w154 {
                tunnel: w153 -> [_ w168]
                tunnel: w152 -> [_ w167]
                tunnel: [_ w166] -> w151
                tunnel: w148 -> [w161 w165]
                tunnel: [w161 w162] -> w147
                frame False {
                }
                frame True {
                  n53 = call "myRIO_BRig_RT_comm_webdav_uploadReceived_read.vi"("input_dataSize"=w167, "input_filePath"=w168) -> ("output_Ivalid"=w166:bool, "output_data"=w164:i64[])  [unwired: 8 in]
                  n54 = To Unsigned Word Integer(number=w164) -> (unsigned 16bit integer=w163:u16[])
                  n55 = Select(t=w163, s=w166, f=w165) -> (s? t:f=w162:u16[])
                }
              }
              n56 = Select(t=myRIO_BRig_RT__Case_NonExp_stateList."UploadSettings_dataExp_1", s=w151, f=myRIO_BRig_RT__Case_NonExp_stateList."UploadSettings_Read_dataLC" ("t")) -> (s? t:f=w146:T1)
            }
            frame "UploadSettings_Read_dataLC" {
              # "grab dataLC and\nstore it in the\ngeneric data array"
              # "dataLC"
              n57 = call "myRIO_BRig_RT_dataLC_init_details.vi"() -> ("output_dataSize"=w175:i32, "output_dataName"=w178:string)  [unwired: 10 in]
              n58 = call "myRIO_BRig_RT_comm_webdav_uploadReceived_check.vi"("input_dataName"=w178) -> ("output_Iexist"=w177:bool, "output_dataPath"=w176:path)  [unwired: 9 in]
              n59 = case shown="True" w177 {
                tunnel: w176 -> [_ w191]
                tunnel: w175 -> [_ w190]
                tunnel: [_ w189] -> w174
                tunnel: w171 -> [w184 w188]
                tunnel: [w184 w185] -> w170
                frame False {
                }
                frame True {
                  n60 = call "myRIO_BRig_RT_comm_webdav_uploadReceived_read.vi"("input_dataSize"=w190, "input_filePath"=w191) -> ("output_Ivalid"=w189:bool, "output_data"=w187:i64[])  [unwired: 8 in]
                  n61 = To Unsigned Word Integer(number=w187) -> (unsigned 16bit integer=w186:u16[])
                  n62 = Select(t=w186, s=w189, f=w188) -> (s? t:f=w185:u16[])
                }
              }
              n63 = Select(t=myRIO_BRig_RT__Case_NonExp_stateList."UploadSettings_dataLC_1", s=w174, f=myRIO_BRig_RT__Case_NonExp_stateList."UploadSettings_Read_dataMTrig" ("t")) -> (s? t:f=w169:T1)
            }
            frame "UploadSettings_Read_dataMTrig" {
              # "grab dataMTrig and\nstore it in the\ngeneric data array"
              # "dataMTrig"
              n64 = call "myRIO_BRig_RT_dataMTrig_init_details.vi"() -> ("output_dataSize"=w198:i32, "output_dataName"=w201:string)  [unwired: 10 in]
              n65 = call "myRIO_BRig_RT_comm_webdav_uploadReceived_check.vi"("input_dataName"=w201) -> ("output_Iexist"=w200:bool, "output_dataPath"=w199:path)  [unwired: 9 in]
              n66 = case shown="True" w200 {
                tunnel: w199 -> [_ w214]
                tunnel: w198 -> [_ w213]
                tunnel: [_ w212] -> w197
                tunnel: w194 -> [w207 w211]
                tunnel: [w207 w208] -> w193
                frame False {
                }
                frame True {
                  n67 = call "myRIO_BRig_RT_comm_webdav_uploadReceived_read.vi"("input_dataSize"=w213, "input_filePath"=w214) -> ("output_Ivalid"=w212:bool, "output_data"=w210:i64[])  [unwired: 8 in]
                  n68 = To Unsigned Word Integer(number=w210) -> (unsigned 16bit integer=w209:u16[])
                  n69 = Select(t=w209, s=w212, f=w211) -> (s? t:f=w208:u16[])
                }
              }
              n70 = Select(t=myRIO_BRig_RT__Case_NonExp_stateList."UploadSettings_dataMTrig_1", s=w197, f=myRIO_BRig_RT__Case_NonExp_stateList."Idle" ("t")) -> (s? t:f=w192:T1)
            }
            frame "UploadSettings_dataExp_1" {
              w218 = u16 1000 ("y")
              # "Cue_max"
              # "Cue_min"
              # "CuePenalty"
              # "Timeout"
              # "Wrong"
              # "Selection"
              # "RewardPost"
              # "Reward_R"
              # "Reward_L"
              # "Tcycle"
              # "TPB_min_R"
              # "TPB_min_L"
              # "TPB_max_R"
              # "TPB_max_L"
              # "I_trialUntilReward"
              # "ENL_penalty"
              # "ENL_min"
              # "ENL_max"
              # "BUR_max"
              # "BUR_min"
              # "CueCycles"
              # "Audio_Freq_R"
              # "Audio_Freq_L"
              # "Audio_Amp_R"
              # "Audio_Amp_L"
              n71 = call "myRIO_BRig_RT_dataExp_CueCycles.vi"() -> ("output_CueCycles"=w261:i32)  [unwired: 11 in]
              n72 = call "myRIO_BRig_RT_dataExp_Audio_amp__R.vi"() -> ("output_Audio_amp__R"=w265:i32)  [unwired: 11 in]
              n73 = call "myRIO_BRig_RT_dataExp_Audio_amp__L.vi"() -> ("output_Audio_amp__L"=w267:i32)  [unwired: 11 in]
              n74 = call "myRIO_BRig_RT_dataExp_BUR_min.vi"() -> ("output_BUR_min"=w258:i32)  [unwired: 11 in]
              n75 = call "myRIO_BRig_RT_dataExp_ENL_min.vi"() -> ("output_ENL_min"=w254:i32)  [unwired: 11 in]
              n76 = call "myRIO_BRig_RT_dataExp_TPB_max__L.vi"() -> ("output_TPB_max__L"=w246:i32)  [unwired: 11 in]
              n77 = call "myRIO_BRig_RT_dataExp_TPB_max__R.vi"() -> ("output_TPB_max__R"=w245:i32)  [unwired: 11 in]
              n78 = call "myRIO_BRig_RT_dataExp_Tcycle_Reward__L.vi"() -> ("output_Tcycle_Reward__L"=w238:i32)  [unwired: 11 in]
              n79 = call "myRIO_BRig_RT_dataExp_Tcycle_Reward__R.vi"() -> ("output_Tcycle_Reward__R"=w237:i32)  [unwired: 11 in]
              n80 = call "myRIO_BRig_RT_dataExp_Tcycle_RewardPost.vi"() -> ("output_Tcycle_RewardPost"=w236:i32)  [unwired: 11 in]
              n81 = call "myRIO_BRig_RT_dataExp_ENL_penalty.vi"() -> ("output_ENL_penalty"=w253:i32)  [unwired: 11 in]
              n82 = call "myRIO_BRig_RT_dataExp_Audio_freq__L.vi"() -> ("output_Audio_freq__L"=w263:i32)  [unwired: 11 in]
              n83 = call "myRIO_BRig_RT_dataExp_Audio_freq__R.vi"() -> ("output_Audio_freq__R"=w262:i32)  [unwired: 11 in]
              n84 = call "myRIO_BRig_RT_dataExp_BUR_max.vi"() -> ("output_BUR_max"=w259:i32)  [unwired: 11 in]
              n85 = call "myRIO_BRig_RT_dataExp_ENL_max.vi"() -> ("output_ENL_max"=w255:i32)  [unwired: 11 in]
              n86 = call "myRIO_BRig_RT_dataExp_ItrialUntilReward.vi"() -> ("output_I_trialUntilReward"=w249:i32)  [unwired: 11 in]
              n87 = call "myRIO_BRig_RT_dataExp_Tcycle_Selection.vi"() -> ("output_Tcycle_Selection"=w235:i32)  [unwired: 11 in]
              n88 = call "myRIO_BRig_RT_dataExp_Tcycle_Wrong.vi"() -> ("output_Tcycle_Wrong"=w234:i32)  [unwired: 11 in]
              n89 = call "myRIO_BRig_RT_dataExp_Tcycle_Timeout.vi"() -> ("output_Tcycle_Timeout"=w233:i32)  [unwired: 11 in]
              n90 = call "myRIO_BRig_RT_dataExp_TPB_min__L.vi"() -> ("output_TPB_min__L"=w244:i32)  [unwired: 11 in]
              n91 = call "myRIO_BRig_RT_dataExp_TPB_min__R.vi"() -> ("output_TPB_min__R"=w243:i32)  [unwired: 11 in]
              n92 = call "myRIO_BRig_RT_dataExp_Tcycle_CuePenalty.vi"() -> ("output_Tcycle_CuePenalty"=w226:i32)  [unwired: 11 in]
              n93 = call "myRIO_BRig_RT_dataExp_Tcycle_Cue_min.vi"() -> ("output_Tcycle_Cue_min"=w225:i32)  [unwired: 11 in]
              n94 = call "myRIO_BRig_RT_dataExp_Tcycle_Cue_max.vi"() -> ("output_Tcycle_Cue_max"=w224:i32)  [unwired: 11 in]
              n95 = Index Array(array=w217, index #1=w267, index #2=w265, index #3=w263, index #4=w262, index #5=w261, index #6=w259, index #7=w258, index #8=w255, index #9=w254, index #10=w253, index #11=w249, index #12=w246, index #13=w245, index #14=w244, index #15=w243, index #16=w238, index #17=w237, index #18=w236, index #19=w235, index #20=w234, index #21=w233, index #22=w226, index #23=w225, index #24=w224) -> (element #1=w266:u16, element #2=w264:u16, element #3=w221:u16, element #4=w220:u16, element #5=w260:u16, element #6=w257:u16, element #7=w256:u16, element #8=w252:u16, element #9=w251:u16, element #10=w250:u16, element #11=w247:u16, element #12=w242:u16, element #13=w241:u16, element #14=w240:u16, element #15=w239:u16, element #16=w232:u16, element #17=w231:u16, element #18=w230:u16, element #19=w229:u16, element #20=w228:u16, element #21=w227:u16, element #22=w223:u16, element #23=w216:u16, element #24=w215:u16)
              n96 = local write "Tcycle_Selection"(w229) -> ()
              n97 = local write "Tcycle_Wrong"(w228) -> ()
              n98 = local write "Tcycle_Timeout"(w227) -> ()
              n99 = local write "Audio_Amp__L"(w266) -> ()
              n100 = local write "Audio_Amp__R"(w264) -> ()
              n101 = local write "Tcycle_ENLPenalty"(w250) -> ()
              n102 = local write "Tcycle_ENL_max"(w252) -> ()
              n103 = local write "TpB_Min_L"(w240) -> ()
              n104 = local write "TpB_Min_R"(w239) -> ()
              n105 = local write "Tcycle_CuePenalty"(w223) -> ()
              n106 = local write "Tcycle_Cue_min"(w216) -> ()
              n107 = local write "Tcycle_Cue_max"(w215) -> ()
              n108 = Quotient & Remainder(x=w221, y=w218) -> (floor(x/y)=w222:u16)  [unwired: 1 out]
              n109 = Quotient & Remainder(x=w220, y=w218) -> (floor(x/y)=w219:u16)  [unwired: 1 out]
              n110 = Not Equal To 0?(x=w247) -> (x != 0?=w248:bool)
              n111 = local write "Tcycle_Reward_L"(w232) -> ()
              n112 = local write "Tcycle_Reward_R"(w231) -> ()
              n113 = local write "Tcycle_RewardPost"(w230) -> ()
              n114 = local write "CueCycles"(w260) -> ()
              n115 = local write "BUR_min"(w256) -> ()
              n116 = local write "BUR_max"(w257) -> ()
              n117 = local write "Tcycle_ENL_min"(w251) -> ()
              n118 = local write "TpB_Max_L"(w242) -> ()
              n119 = local write "TpB_Max_R"(w241) -> ()
              n120 = local write "TrialUntilReward"(w248) -> ()
              n121 = local write "Audio_Freq__L"(w222) -> ()
              n122 = local write "Audio_Freq__R"(w219) -> ()
            }
            frame "UploadSettings_dataLC_1" {
              # "Cue1_All_delayOpt"
              # "ENL1_All_delayOpt"
              # "Cue1_First_delayOpt"
              # "ENL1_First_delayOpt"
              # "ENL1 First"
              # "Cue1 All"
              # "Cue1 First"
              # "Count"
              # "Tdelay"
              # "Prob"
              # "OnOff"
              # "Block"
              # "ENL1 All"
              # "Count"
              # "Tdelay"
              # "Prob"
              # "OnOff"
              # "Block"
              # "Count"
              # "Tdelay"
              # "Prob"
              # "Block"
              # "OnOff"
              # "Count"
              # "Tdelay"
              # "Prob"
              # "OnOff"
              # "Block"
              n123 = call "myRIO_BRig_RT_dataLC_Cue1_First_Block.vi"() -> ("output_Cue1_First_Block"=w330:i32)  [unwired: 11 in]
              n124 = call "myRIO_BRig_RT_dataLC_Cue1_First_OnOff.vi"() -> ("output_Cue1_First_OnOff"=w328:i32)  [unwired: 11 in]
              n125 = call "myRIO_BRig_RT_dataLC_Cue1_First_Count.vi"() -> ("output_Cue1_First_Count"=w325:i32)  [unwired: 11 in]
              n126 = call "myRIO_BRig_RT_dataLC_Cue1_All_Block.vi"() -> ("output_Cue1_All_Block"=w312:i32)  [unwired: 11 in]
              n127 = call "myRIO_BRig_RT_dataLC_Cue1_All_OnOff.vi"() -> ("output_Cue1_All_OnOff"=w311:i32)  [unwired: 11 in]
              n128 = call "myRIO_BRig_RT_dataLC_Cue1_All_Count.vi"() -> ("output_Cue1_All_Count"=w322:i32)  [unwired: 11 in]
              n129 = call "myRIO_BRig_RT_dataLC_ENL1_First_Block.vi"() -> ("output_ENL1_First_Block"=w310:i32)  [unwired: 11 in]
              n130 = call "myRIO_BRig_RT_dataLC_ENL1_First_OnOff.vi"() -> ("output_ENL1_First_OnOff"=w321:i32)  [unwired: 11 in]
              n131 = call "myRIO_BRig_RT_dataLC_ENL1_First_Count.vi"() -> ("output_ENL1_First_Count"=w318:i32)  [unwired: 11 in]
              n132 = call "myRIO_BRig_RT_dataLC_ENL1_All_Block.vi"() -> ("output_ENL1_All_Block"=w317:i32)  [unwired: 11 in]
              n133 = call "myRIO_BRig_RT_dataLC_ENL1_All_OnOff.vi"() -> ("output_ENL1_All_OnOff"=w316:i32)  [unwired: 11 in]
              n134 = call "myRIO_BRig_RT_dataLC_ENL1_All_Count.vi"() -> ("output_ENL1_All_Count"=w313:i32)  [unwired: 11 in]
              n135 = call "myRIO_BRig_RT_dataLC_ENL1_First_delayOpt.vi"() -> ("output_ENL1_First_delayOpt"=w287:i32)  [unwired: 11 in]
              n136 = call "myRIO_BRig_RT_dataLC_Cue1_First_delayOpt.vi"() -> ("output_Cue1_First_delayOpt"=w286:i32)  [unwired: 11 in]
              n137 = call "myRIO_BRig_RT_dataLC_ENL1_All_delayOpt.vi"() -> ("output_ENL1_All_delayOpt"=w279:i32)  [unwired: 11 in]
              n138 = call "myRIO_BRig_RT_dataLC_Cue1_All_delayOpt.vi"() -> ("output_Cue1_All_delayOpt"=w278:i32)  [unwired: 11 in]
              n139 = call "myRIO_BRig_RT_dataLC_Cue1_First_Probability.vi"() -> ("output_Cue1_First_Probability"=w327:i32)  [unwired: 11 in]
              n140 = call "myRIO_BRig_RT_dataLC_Cue1_First_Tdelay.vi"() -> ("output_Cue1_First_Tdelay"=w326:i32)  [unwired: 11 in]
              n141 = call "myRIO_BRig_RT_dataLC_Cue1_All_Probability.vi"() -> ("output_Cue1_All_Probability"=w324:i32)  [unwired: 11 in]
              n142 = call "myRIO_BRig_RT_dataLC_Cue1_All_Tdelay.vi"() -> ("output_Cue1_All_Tdelay"=w323:i32)  [unwired: 11 in]
              n143 = call "myRIO_BRig_RT_dataLC_ENL1_First_Probability.vi"() -> ("output_ENL1_First_Probability"=w320:i32)  [unwired: 11 in]
              n144 = call "myRIO_BRig_RT_dataLC_ENL1_First_Tdelay.vi"() -> ("output_ENL1_First_Tdelay"=w319:i32)  [unwired: 11 in]
              n145 = call "myRIO_BRig_RT_dataLC_ENL1_All_Probability.vi"() -> ("output_ENL1_All_Probability"=w315:i32)  [unwired: 11 in]
              n146 = call "myRIO_BRig_RT_dataLC_ENL1_All_Tdelay.vi"() -> ("output_ENL1_All_Tdelay"=w314:i32)  [unwired: 11 in]
              n147 = Index Array(array=w288, index #1=w330, index #2=w328, index #3=w327, index #4=w326, index #5=w325, index #6=w312, index #7=w311, index #8=w324, index #9=w323, index #10=w322, index #11=w310, index #12=w321, index #13=w320, index #14=w319, index #15=w318, index #16=w317, index #17=w316, index #18=w315, index #19=w314, index #20=w313, index #21=w287, index #22=w286, index #23=w279, index #24=w278) -> (element #1=w329:u16, element #2=w308:u16, element #3=w307:u16, element #4=w306:u16, element #5=w305:u16, element #6=w301:u16, element #7=w300:u16, element #8=w299:u16, element #9=w298:u16, element #10=w297:u16, element #11=w296:u16, element #12=w295:u16, element #13=w294:u16, element #14=w293:u16, element #15=w280:u16, element #16=w292:u16, element #17=w291:u16, element #18=w290:u16, element #19=w289:u16, element #20=w281:u16, element #21=w284:u16, element #22=w282:u16, element #23=w275:u16, element #24=w274:u16)
              n148 = Not Equal To 0?(x=w275) -> (x != 0?=w277:bool)
              n149 = Not Equal To 0?(x=w274) -> (x != 0?=w276:bool)
              n150 = Not Equal To 0?(x=w284) -> (x != 0?=w285:bool)
              n151 = Not Equal To 0?(x=w282) -> (x != 0?=w283:bool)
              n152 = Not Equal To 0?(x=w308) -> (x != 0?=w309:bool)
              n153 = Not Equal To 0?(x=w300) -> (x != 0?=w304:bool)
              n154 = Not Equal To 0?(x=w295) -> (x != 0?=w303:bool)
              n155 = Not Equal To 0?(x=w291) -> (x != 0?=w302:bool)
              n156 = local write "LC_Cue1_First_Probability"(w307) -> ()
              n157 = local write "LC_ENL1_First_Probability"(w294) -> ()
              n158 = local write "LC_ENL1_First_delayOpt"(w285) -> ()
              n159 = local write "LC_Cue1_First_delayOpt"(w283) -> ()
              n160 = local write "LC_ENL1_All_delayOpt"(w277) -> ()
              n161 = local write "LC_Cue1_All_delayOpt"(w276) -> ()
              n162 = local write "LC_Cue1_All_Probability"(w299) -> ()
              n163 = local write "LC_Cue1_First_Tdelay"(w306) -> ()
              n164 = local write "LC_ENL1_All_Probability"(w290) -> ()
              n165 = local write "LC_Cue1_First_OnOff"(w309) -> ()
              n166 = local write "LC_Cue1_First_Count"(w305) -> ()
              n167 = local write "LC_Cue1_First_Block"(w329) -> ()
              n168 = local write "LC_ENL1_First_Tdelay"(w293) -> ()
              n169 = local write "LC_ENL1_First_OnOff"(w303) -> ()
              n170 = local write "LC_ENL1_First_Count"(w280) -> ()
              n171 = local write "LC_ENL1_First_Block"(w296) -> ()
              n172 = local write "LC_Cue1_All_Tdelay"(w298) -> ()
              n173 = local write "LC_Cue1_All_OnOff"(w304) -> ()
              n174 = local write "LC_Cue1_All_Count"(w297) -> ()
              n175 = local write "LC_Cue1_All_Block"(w301) -> ()
              n176 = local write "LC_ENL1_All_Tdelay"(w289) -> ()
              n177 = local write "LC_ENL1_All_OnOff"(w302) -> ()
              n178 = local write "LC_ENL1_All_Count"(w281) -> ()
              n179 = local write "LC_ENL1_All_Block"(w292) -> ()
            }
            frame "UploadSettings_dataLC_2" {
              # "Wrong"
              # "Reward"
              # "Trial"
              # "Tdelay"
              # "Prob"
              # "Block"
              # "OnOff"
              # "Trial"
              # "Tdelay"
              # "Prob"
              # "OnOff"
              # "Block"
              n180 = call "myRIO_BRig_RT_dataLC_Reward_Block.vi"() -> ("output_Reward_Block"=w363:i32)  [unwired: 11 in]
              n181 = call "myRIO_BRig_RT_dataLC_Reward_OnOff.vi"() -> ("output_Reward_OnOff"=w361:i32)  [unwired: 11 in]
              n182 = call "myRIO_BRig_RT_dataLC_Reward_Trial.vi"() -> ("output_Reward_Trial"=w358:i32)  [unwired: 11 in]
              n183 = call "myRIO_BRig_RT_dataLC_Wrong_Block.vi"() -> ("output_Wrong_Block"=w354:i32)  [unwired: 11 in]
              n184 = call "myRIO_BRig_RT_dataLC_Wrong_OnOff.vi"() -> ("output_Wrong_OnOff"=w353:i32)  [unwired: 11 in]
              n185 = call "myRIO_BRig_RT_dataLC_Wrong_Trial.vi"() -> ("output_Wrong_Trial"=w355:i32)  [unwired: 11 in]
              n186 = call "myRIO_BRig_RT_dataLC_Reward_Probability.vi"() -> ("output_Reward_Probability"=w360:i32)  [unwired: 11 in]
              n187 = call "myRIO_BRig_RT_dataLC_Reward_Tdelay.vi"() -> ("output_Reward_Tdelay"=w359:i32)  [unwired: 11 in]
              n188 = call "myRIO_BRig_RT_dataLC_Wrong_Probability.vi"() -> ("output_Wrong_Probability"=w357:i32)  [unwired: 11 in]
              n189 = call "myRIO_BRig_RT_dataLC_Wrong_Tdelay.vi"() -> ("output_Wrong_Tdelay"=w356:i32)  [unwired: 11 in]
              n190 = Index Array(array=w337, index #1=w363, index #2=w361, index #3=w360, index #4=w359, index #5=w358, index #6=w354, index #7=w353, index #8=w357, index #9=w356, index #10=w355) -> (element #1=w362:u16, element #2=w351:u16, element #3=w350:u16, element #4=w349:u16, element #5=w348:u16, element #6=w346:u16, element #7=w345:u16, element #8=w344:u16, element #9=w343:u16, element #10=w342:u16)
              n191 = Not Equal To 0?(x=w351) -> (x != 0?=w352:bool)
              n192 = Not Equal To 0?(x=w345) -> (x != 0?=w347:bool)
              n193 = local write "LC_Reward_Probability"(w350) -> ()
              n194 = local write "LC_Wrong_Probability"(w344) -> ()
              n195 = local write "LC_Reward_Tdelay"(w349) -> ()
              n196 = local write "LC_Reward_OnOff"(w352) -> ()
              n197 = local write "LC_Reward_Block"(w362) -> ()
              n198 = local write "LC_Reward_Trial"(w348) -> ()
              n199 = local write "LC_Wrong_Tdelay"(w343) -> ()
              n200 = local write "LC_Wrong_OnOff"(w347) -> ()
              n201 = local write "LC_Wrong_Block"(w346) -> ()
              n202 = local write "LC_Wrong_Trial"(w342) -> ()
            }
            frame "UploadSettings_dataMTrig_1" {
              # "Tdelay_R"
              # "Tdelay_L"
              # "Tcycle_R"
              # "Tcycle_L"
              # "RewCalib_nCycle_R"
              # "RewCalib_nCycle_L"
              # "Solenoid"
              # "Laser_Tcycle"
              n203 = call "myRIO_BRig_RT_dataMTrig_Laser_Tcycle.vi"() -> ("output_Laser_Tcycle"=w373:i32)  [unwired: 11 in]
              n204 = call "myRIO_BRig_RT_dataMTrig_Solenoid_RewCalib_nCycle__L.vi"() -> ("output_Solenoid_RewCalib_nCycle__L"=w372:i32)  [unwired: 11 in]
              n205 = call "myRIO_BRig_RT_dataMTrig_Solenoid_RewCalib_nCycle__R.vi"() -> ("output_Solenoid_RewCalib_nCycle__R"=w371:i32)  [unwired: 11 in]
              n206 = call "myRIO_BRig_RT_dataMTrig_Solenoid_Tdelay__L.vi"() -> ("output_Solenoid_Tdelay__L"=w368:i32)  [unwired: 11 in]
              n207 = call "myRIO_BRig_RT_dataMTrig_Solenoid_Tdelay__R.vi"() -> ("output_Solenoid_Tdelay__R"=w367:i32)  [unwired: 11 in]
              n208 = call "myRIO_BRig_RT_dataMTrig_Solenoid_Tcycle__L.vi"() -> ("output_Solenoid_Tcycle__L"=w370:i32)  [unwired: 11 in]
              n209 = call "myRIO_BRig_RT_dataMTrig_Solenoid_Tcycle__R.vi"() -> ("output_Solenoid_Tcycle__R"=w369:i32)  [unwired: 11 in]
              n210 = Index Array(array=w366, index #1=w373, index #2=w372, index #3=w371, index #4=w370, index #5=w369, index #6=w368, index #7=w367) -> (element #1=w380:u16, element #2=w379:u16, element #3=w378:u16, element #4=w377:u16, element #5=w376:u16, element #6=w375:u16, element #7=w374:u16)
              n211 = Replace Array Subset(array=w386, new element #1=w380, index #1=w373, new element #2=w379, index #2=w372, new element #3=w378, index #3=w371, new element #4=w377, index #4=w370, new element #5=w376, index #5=w369, new element #6=w375, index #6=w368, new element #7=w374, index #7=w367) -> (w385:u16[])
              n212 = local write "MTrig_Solenoid_Tcycle__L"(w377) -> ()
              n213 = local write "MTrig_Solenoid_Tcycle__R"(w376) -> ()
              n214 = local write "MTrig_Laser_Tcycle"(w380) -> ()
            }
            frame "Idle" {
              w406 = u16 1000 ("y")
              # "To ensure timing, we split the\nidle state into 4 phases"
              # "Laser_Tcycle"
              # "Audio_Tcycle_R"
              # "Audio_Tcycle_L"
              n215 = local read "MTrig_Audio_trig__L"() -> (w395:bool)
              n216 = local read "MTrig_Audio_trig__R"() -> (w397:bool)
              n217 = Select(t=myRIO_BRig_RT__Case_NonExp_stateList."SendData" ("Enum"), s="SendData", f=myRIO_BRig_RT__Case_NonExp_stateList."Idle_2" ("Enum")) -> (s? t:f=w390:T1)
              n218 = local read "MTrig_Laser_trig"() -> (w396:bool)
              n219 = call "myRIO_BRig_RT_dataMTrig_Audio_Tcycle__L.vi"() -> ("output_Audio_Tcycle__L"=w413:i32)  [unwired: 11 in]
              n220 = call "myRIO_BRig_RT_dataMTrig_Audio_Tcycle__R.vi"() -> ("output_Audio_Tcycle__R"=w412:i32)  [unwired: 11 in]
              n221 = call "myRIO_BRig_RT_dataMTrig_Laser_Tcycle.vi"() -> ("output_Laser_Tcycle"=w411:i32)  [unwired: 11 in]
              n222 = local read "MTrig_Laser_Tcycle"() -> (w388:u16)
              n223 = Select(t=myRIO_BRig_RT__Case_NonExp_stateList."TestConnection" ("Enum"), s="TestConnection", f=w390) -> (s? t:f=w399:T1)
              n224 = local read "Tcycle_Cue_min"() -> (w389:u16)
              n225 = Compound Arithmetic op=OR(w395, w397, w396) -> (w398:bool)
              n226 = case shown="True" w398 {
                frame False {
                }
                frame True {
                  w414 = FALSE
                  n227 = local write "MTrig_Audio_trig__L"(w414) -> ()
                  n228 = local write "MTrig_Audio_trig__R"(w414) -> ()
                  n229 = local write "MTrig_Laser_trig"(w414) -> ()
                }
              }
              n230 = Replace Array Subset(array=w409, new element #1=w389, index #1=w413, new element #2=w389, index #2=w412, new element #3=w388, index #3=w411) -> (w410:u16[])
              n231 = local read "Audio_Amp__R"() -> (w402:u16)
              n232 = local read "Audio_Amp__L"() -> (w403:u16)
              n233 = local read "Audio_Freq__R"() -> (w400:u16)
              n234 = local read "Audio_Freq__L"() -> (w401:u16)
              n235 = Multiply(x=w400, y=w406) -> (x*y=w404:u16)
              n236 = Multiply(x=w401, y=w406) -> (x*y=w405:u16)
            }
            frame "Idle_2" {
              # "To ensure timing, we split the\nidle state into 4 phases"
              # "Ncycles"
              # "Ncycles"
              # "RewCalib"
              # "RewCalib"
              # "Solenoid R"
              # "Solenoid L"
              n237 = call "myRIO_BRig_RT_dataMTrig_Solenoid_RewCalib_OnOff__L.vi"() -> ("output_Solenoid_RewCalib_OnOff__L"=w444:i32)  [unwired: 11 in]
              n238 = call "myRIO_BRig_RT_dataMTrig_Solenoid_N__L.vi"() -> ("output_Solenoid_N__L"=w432:i32)  [unwired: 11 in]
              n239 = call "myRIO_BRig_RT_dataMTrig_Solenoid_RewCalib_OnOff__R.vi"() -> ("output_Solenoid_RewCalib_OnOff__R"=w429:i32)  [unwired: 11 in]
              n240 = call "myRIO_BRig_RT_dataMTrig_Solenoid_N__R.vi"() -> ("output_Solenoid_N__R"=w428:i32)  [unwired: 11 in]
              n241 = Index Array(array=w435, index #1=w444, index #2=w432, index #3=w429, index #4=w428) -> (element #1=w431:u16, element #2=w426:u16, element #3=w427:u16, element #4=w425:u16)
              n242 = local read "RewCalib_Trig_L"() -> (w424:bool)
              n243 = local read "RewCalib_Trig_R"() -> (w423:bool)
              n244 = Equal To 0?(x=w426) -> (x = 0?=w434:bool)
              n245 = Equal To 0?(x=w425) -> (x = 0?=w433:bool)
              n246 = Not Equal To 0?(x=w427) -> (x != 0?=w445:bool)
              n247 = Not Equal To 0?(x=w431) -> (x != 0?=w446:bool)
              n248 = And(x=w434, y=w433) -> (x .and. y?=w438:bool)
              n249 = Or(x=w424, y=w423) -> (x .or. y?=w439:bool)
              n250 = Not Exclusive Or(1:w446, 2:w424) -> (0:w441:bool)
              n251 = Not Exclusive Or(1:w445, 2:w423) -> (0:w443:bool)
              n252 = And(x=w439, y=w438) -> (x .and. y?=w421:bool)
              n253 = Not(x=w441) -> (.not. x?=w440:bool)
              n254 = Not(x=w443) -> (.not. x?=w442:bool)
              n255 = Or(x=w440, y=w442) -> (x .or. y?=w422:bool)
              n256 = Or(x=w421, y=w422) -> (x .or. y?=w437:bool)
              n257 = Select(t=myRIO_BRig_RT__Case_NonExp_stateList."RewardCalibration_pre" ("Enum"), s=w437, f=myRIO_BRig_RT__Case_NonExp_stateList."Idle_3" ("Enum")) -> (s? t:f=w420:T1)
            }
            frame "Idle_3" {
              w469 = u8 0 ("f")
              # "To ensure timing, we split the\nidle state into 4 phases"
              n258 = local read "MTrig_Solenoid_trig__L"() -> (w455:bool)
              n259 = local read "MTrig_Solenoid_trig__R"() -> (w470:bool)
              n260 = local read "warmupType"() -> (w461:bool)
              n261 = local read "warmup"() -> (w462:bool)
              n262 = Not(x=w461) -> (.not. x?=w463:bool)
              n263 = Select(t=u8 1, s=w455, f=w469) -> (s? t:f=w468:u8)
              n264 = Select(t=u8 2, s=w470, f=w469) -> (s? t:f=w467:u8)
              n265 = And(x=w462, y=w463) -> (x .and. y?=w460:bool)
              n266 = And(x=w462, y=w461) -> (x .and. y?=w450:bool)
              n267 = Add(x=w468, y=w467) -> (x+y=w466:u8)
              n268 = case shown="3" w466 {
                tunnel: w465 -> [w473 w477 w495 w513]
                tunnel: [w473 w476 w494 w512] -> w464
                tunnel: w460 -> [_ w475 w493 w511]
                tunnel: [_ TRUE TRUE TRUE] -> w452
                frame 0, Default {
                }
                frame 1 {
                  n269 = case shown="True" w475 {
                    tunnel: w477 -> [w486 w491]
                    tunnel: [w485 w490] -> w476
                    frame True {
                      # "Audio_L"
                      # "Solenoid_L"
                      n270 = call "myRIO_BRig_RT_dataMTrig_Solenoid_N__L.vi"() -> ("output_Solenoid_N__L"=w482:i32)  [unwired: 11 in]
                      n271 = call "myRIO_BRig_RT_dataMTrig_Audio_N__L.vi"() -> ("output_Audio_N__L"=w480:i32)  [unwired: 11 in]
                      n272 = Index Array(array=w486, index #1=w482, index #2=w480) -> (element #1=w484:u16, element #2=w483:u16)
                      n273 = Increment(x=w484) -> (x+1=w481:u16)
                      n274 = Increment(x=w483) -> (x+1=w479:u16)
                      n275 = Replace Array Subset(array=w486, new element #1=w481, index #1=w482, new element #2=w479, index #2=w480) -> (w485:u16[])
                    }
                    frame False {
                      # "Solenoid_L"
                      n276 = call "myRIO_BRig_RT_dataMTrig_Solenoid_N__L.vi"() -> ("output_Solenoid_N__L"=w488:i32)  [unwired: 11 in]
                      n277 = Index Array(array=w491, index=w488) -> (element=w489:u16)
                      n278 = Increment(x=w489) -> (x+1=w487:u16)
                      n279 = Replace Array Subset(array=w491, new element=w487, index=w488) -> (w490:u16[])
                    }
                  }
                  n280 = local write "MTrig_Solenoid_trig__L"(FALSE) -> ()
                }
                frame 2 {
                  n281 = case shown="True" w493 {
                    tunnel: w495 -> [w504 w509]
                    tunnel: [w503 w508] -> w494
                    frame True {
                      # "Audio_R"
                      # "Solenoid_R"
                      n282 = call "myRIO_BRig_RT_dataMTrig_Solenoid_N__R.vi"() -> ("output_Solenoid_N__R"=w500:i32)  [unwired: 11 in]
                      n283 = call "myRIO_BRig_RT_dataMTrig_Audio_N__R.vi"() -> ("output_Audio_N__R"=w499:i32)  [unwired: 11 in]
                      n284 = Index Array(array=w504, index #1=w500, index #2=w499) -> (element #1=w502:u16, element #2=w501:u16)
                      n285 = Increment(x=w501) -> (x+1=w497:u16)
                      n286 = Increment(x=w502) -> (x+1=w498:u16)
                      n287 = Replace Array Subset(array=w504, new element #1=w498, index #1=w500, new element #2=w497, index #2=w499) -> (w503:u16[])
                    }
                    frame False {
                      # "Solenoid_R"
                      n288 = call "myRIO_BRig_RT_dataMTrig_Solenoid_N__R.vi"() -> ("output_Solenoid_N__R"=w505:i32)  [unwired: 11 in]
                      n289 = Index Array(array=w509, index=w505) -> (element=w507:u16)
                      n290 = Increment(x=w507) -> (x+1=w506:u16)
                      n291 = Replace Array Subset(array=w509, new element=w506, index=w505) -> (w508:u16[])
                    }
                  }
                  n292 = local write "MTrig_Solenoid_trig__R"(FALSE) -> ()
                }
                frame 3 {
                  w514 = FALSE
                  n293 = case shown="True" w511 {
                    tunnel: w513 -> [w528 w536]
                    tunnel: [w527 w535] -> w512
                    frame True {
                      # "Audio_R"
                      # "Solenoid_R"
                      # "Audio_L"
                      # "Solenoid_L"
                      n294 = call "myRIO_BRig_RT_dataMTrig_Solenoid_N__L.vi"() -> ("output_Solenoid_N__L"=w522:i32)  [unwired: 11 in]
                      n295 = call "myRIO_BRig_RT_dataMTrig_Audio_N__L.vi"() -> ("output_Audio_N__L"=w520:i32)  [unwired: 11 in]
                      n296 = call "myRIO_BRig_RT_dataMTrig_Solenoid_N__R.vi"() -> ("output_Solenoid_N__R"=w518:i32)  [unwired: 11 in]
                      n297 = call "myRIO_BRig_RT_dataMTrig_Audio_N__R.vi"() -> ("output_Audio_N__R"=w517:i32)  [unwired: 11 in]
                      n298 = Index Array(array=w528, index #1=w522, index #2=w520, index #3=w518, index #4=w517) -> (element #1=w526:u16, element #2=w525:u16, element #3=w524:u16, element #4=w523:u16)
                      n299 = Increment(x=w523) -> (x+1=w515:u16)
                      n300 = Increment(x=w526) -> (x+1=w521:u16)
                      n301 = Increment(x=w525) -> (x+1=w519:u16)
                      n302 = Increment(x=w524) -> (x+1=w516:u16)
                      n303 = Replace Array Subset(array=w528, new element #1=w521, index #1=w522, new element #2=w519, index #2=w520, new element #3=w516, index #3=w518, new element #4=w515, index #4=w517) -> (w527:u16[])
                    }
                    frame False {
                      # "Solenoid_R"
                      # "Solenoid_L"
                      n304 = call "myRIO_BRig_RT_dataMTrig_Solenoid_N__L.vi"() -> ("output_Solenoid_N__L"=w532:i32)  [unwired: 11 in]
                      n305 = call "myRIO_BRig_RT_dataMTrig_Solenoid_N__R.vi"() -> ("output_Solenoid_N__R"=w529:i32)  [unwired: 11 in]
                      n306 = Index Array(array=w536, index #1=w532, index #2=w529) -> (element #1=w534:u16, element #2=w533:u16)
                      n307 = Increment(x=w534) -> (x+1=w531:u16)
                      n308 = Increment(x=w533) -> (x+1=w530:u16)
                      n309 = Replace Array Subset(array=w536, new element #1=w531, index #1=w532, new element #2=w530, index #2=w529) -> (w535:u16[])
                    }
                  }
                  n310 = local write "MTrig_Solenoid_trig__L"(w514) -> ()
                  n311 = local write "MTrig_Solenoid_trig__R"(w514) -> ()
                }
              }
              n312 = Select(t=myRIO_BRig_RT__Case_NonExp_stateList."Cue_pre", s=w450, f=myRIO_BRig_RT__Case_NonExp_stateList."DispenseWater_pre" ("Enum")) -> (s? t:f=w448:T1)
              n313 = Select(t=w448, s=w452, f=myRIO_BRig_RT__Case_NonExp_stateList."Idle_4" ("Enum")) -> (s? t:f=w453:T1)
            }
            frame "Idle_4" {
              # "use dataMTrig as it is one of the last to transfer"
              # "To ensure timing, we split the\nidle state into 4 phases"
              n314 = call "myRIO_BRig_RT_comm_webdav_uploadReceived_check_v2,0.vi"("input_dataName"="dataMTrig") -> ("output_Iexist"=w546:bool)  [unwired: 9 in, 1 out]
              n315 = Select(t=myRIO_BRig_RT__Case_NonExp_stateList."UploadSettings_pre" ("Enum"), s=w546, f=myRIO_BRig_RT__Case_NonExp_stateList."Idle") -> (s? t:f=w544:T1)
            }
            frame "Cue_pre" {
              w554 = u16 1 ("t")
              w553 = u16 0 ("new element/subarray")
              w550 = u16 0 ("new element/subarray")
              # "Ncycle"
              # "count"
              # "Audio_R"
              # "Solenoid_R"
              # "Solenoid_L"
              # "Ncycle"
              # "count"
              # "Audio_L"
              n316 = call "myRIO_BRig_RT_dataMTrig_Solenoid_N__L.vi"() -> ("output_Solenoid_N__L"=w565:i32)  [unwired: 11 in]
              n317 = call "myRIO_BRig_RT_dataMTrig_Solenoid_N__R.vi"() -> ("output_Solenoid_N__R"=w564:i32)  [unwired: 11 in]
              n318 = Index Array(array=w561, index #1=w565, index #2=w564) -> (element #1=w563:u16, element #2=w562:u16)
              n319 = Not Equal To 0?(x=w562) -> (x != 0?=w555:bool)
              n320 = Not Equal To 0?(x=w563) -> (x != 0?=w557:bool)
              n321 = Select(t=w554, s=w557, f=w553) -> (s? t:f=w556:u16)
              n322 = Select(t=w554, s=w555, f=w553) -> (s? t:f=w549:u16)
              n323 = call "myRIO_BRig_RT_dataMTrig_Audio_c__L.vi"() -> ("output_Audio_c__L"=w559:i32)  [unwired: 11 in]
              n324 = call "myRIO_BRig_RT_dataMTrig_Audio_N__L.vi"() -> ("output_Audio_N__L"=w558:i32)  [unwired: 11 in]
              n325 = call "myRIO_BRig_RT_dataMTrig_Audio_c__R.vi"() -> ("output_Audio_c__R"=w552:i32)  [unwired: 11 in]
              n326 = call "myRIO_BRig_RT_dataMTrig_Audio_N__R.vi"() -> ("output_Audio_N__R"=w551:i32)  [unwired: 11 in]
              n327 = Replace Array Subset(array=w561, new element #1=w550, index #1=w559, new element #2=w556, index #2=w558, new element #3=w550, index #3=w552, new element #4=w549, index #4=w551) -> (w560:u16[])
            }
            frame "Cue" {
              # "Ncycle"
              # "Audio_R"
              # "Ncycle"
              # "Audio_L"
              n328 = call "myRIO_BRig_RT_dataMTrig_Audio_N__L.vi"() -> ("output_Audio_N__L"=w581:i32)  [unwired: 11 in]
              n329 = call "myRIO_BRig_RT_dataMTrig_Audio_N__R.vi"() -> ("output_Audio_N__R"=w580:i32)  [unwired: 11 in]
              n330 = Index Array(array=w586, index #1=w581, index #2=w580) -> (element #1=w579:u16, element #2=w578:u16)
              n331 = Equal To 0?(x=w579) -> (x = 0?=w577:bool)
              n332 = Equal To 0?(x=w578) -> (x = 0?=w576:bool)
              n333 = And(x=w577, y=w576) -> (x .and. y?=w575:bool)
              n334 = Select(t=myRIO_BRig_RT__Case_NonExp_stateList."DispenseWater_pre", s=w575, f=w573) -> (s? t:f=w572:T1)
            }
            frame "RewardCalibration_pre" {
              (unwired) FALSE
              w592 = FALSE
              w603 = u8 0
              w619 = u8 0
              # "Are we starting a RewardCalibration?\nOr are we stopping a RewardCalibration?\nOr is a RewardCalibration over?"
              # "RewCalib\nOnOff"
              # "N"
              # "Solenoid R"
              # "RewCalib\nOnOff"
              # "N"
              # "Solenoid L"
              n335 = local read "RewCalib_Trig_L"() -> (w626:bool)
              n336 = local read "RewCalib_Trig_R"() -> (w595:bool)
              n337 = call "myRIO_BRig_RT_dataMTrig_Solenoid_N__R.vi"() -> ("output_Solenoid_N__R"=w597:i32)  [unwired: 11 in]
              n338 = call "myRIO_BRig_RT_dataMTrig_Solenoid_RewCalib_OnOff__R.vi"() -> ("output_Solenoid_RewCalib_OnOff__R"=w594:i32)  [unwired: 11 in]
              n339 = call "myRIO_BRig_RT_dataMTrig_Solenoid_N__L.vi"() -> ("output_Solenoid_N__L"=w612:i32)  [unwired: 11 in]
              n340 = call "myRIO_BRig_RT_dataMTrig_Solenoid_RewCalib_OnOff__L.vi"() -> ("output_Solenoid_RewCalib_OnOff__L"=w613:i32)  [unwired: 11 in]
              n341 = Index Array(array=w596, index #1=w597, index #2=w594) -> (element #1=w607:u16, element #2=w602:u16)
              n342 = Index Array(array=w596, index #1=w612, index #2=w613) -> (element #1=w623:u16, element #2=w618:u16)
              n343 = Equal To 0?(x=w607) -> (x = 0?=w608:bool)
              n344 = Not Equal To 0?(x=w602) -> (x != 0?=w605:bool)
              n345 = Equal To 0?(x=w623) -> (x = 0?=w624:bool)
              n346 = Not Equal To 0?(x=w618) -> (x != 0?=w621:bool)
              n347 = local write "MTrig_Solenoid_trig__L"(w592) -> ()
              n348 = local write "MTrig_Solenoid_trig__R"(w592) -> ()
              n349 = Select(t=u8 1, s=w595, f=w603) -> (s? t:f=w599:u8)
              n350 = Select(t=u8 1, s=w626, f=w619) -> (s? t:f=w615:u8)
              n351 = Select(t=u8 2, s=w608, f=w603) -> (s? t:f=w600:u8)
              n352 = Select(t=u8 4, s=w605, f=w603) -> (s? t:f=w601:u8)
              n353 = Select(t=u8 2, s=w624, f=w619) -> (s? t:f=w616:u8)
              n354 = Select(t=u8 4, s=w621, f=w619) -> (s? t:f=w617:u8)
              n355 = Compound Arithmetic op=ADD(w599, w600, w601) -> (w598:u8)
              n356 = Compound Arithmetic op=ADD(w615, w616, w617) -> (w614:u8)
              n357 = case shown="7" w614 {
                tunnel: w596 -> [w656 w661 w663 w668 w673 w675 w678 w683]
                tunnel: [w656 w662 w663 w669 w674 w675 w679 w684] -> w611
                tunnel: w613 -> [_ w659 _ w666 w671 _ w677 w682]
                tunnel: w612 -> [_ w660 _ w667 w672 _ _ _]
                frame 0, Default {
                }
                frame 1 {
                  n358 = Replace Array Subset(array=w661, new element #1=u16 100 ("new element/subarray"), index #1=w660, new element #2=u16 1 ("new element/subarray"), index #2=w659) -> (w662:u16[])
                }
                frame 2 {
                }
                frame 3 {
                  n359 = Replace Array Subset(array=w668, new element #1=u16 100 ("new element/subarray"), index #1=w667, new element #2=u16 1 ("new element/subarray"), index #2=w666) -> (w669:u16[])
                }
                frame 4 {
                  w670 = u16 0 ("new element/subarray")
                  n360 = Replace Array Subset(array=w673, new element #1=w670, index #1=w672, new element #2=w670, index #2=w671) -> (w674:u16[])
                }
                frame 5 {
                }
                frame 6 {
                  n361 = Replace Array Subset(array=w678, new element=u16 0 ("new element/subarray"), index=w677) -> (w679:u16[])
                }
                frame 7 {
                  n362 = local write "RewCalib_Trig_L"(FALSE ("RewCalib_Trig_L")) -> ()
                  n363 = Replace Array Subset(array=w683, new element=u16 0 ("new element/subarray"), index=w682) -> (w684:u16[])
                }
              }
              n364 = case shown="7" w598 {
                tunnel: w611 -> [w627 w632 w634 w639 w644 w646 w649 w654]
                tunnel: [w627 w633 w634 w640 w645 w646 w650 w655] -> w610
                tunnel: w594 -> [_ w630 _ w637 w642 _ w648 w653]
                tunnel: w597 -> [_ w631 _ w638 w643 _ _ _]
                frame 0, Default {
                }
                frame 1 {
                  n365 = Replace Array Subset(array=w632, new element #1=u16 100 ("new element/subarray"), index #1=w631, new element #2=u16 1 ("new element/subarray"), index #2=w630) -> (w633:u16[])
                }
                frame 2 {
                }
                frame 3 {
                  n366 = Replace Array Subset(array=w639, new element #1=u16 100 ("new element/subarray"), index #1=w638, new element #2=u16 1 ("new element/subarray"), index #2=w637) -> (w640:u16[])
                }
                frame 4 {
                  w641 = u16 0 ("new element/subarray")
                  n367 = Replace Array Subset(array=w644, new element #1=w641, index #1=w643, new element #2=w641, index #2=w642) -> (w645:u16[])
                }
                frame 5 {
                }
                frame 6 {
                  n368 = Replace Array Subset(array=w649, new element=u16 0 ("new element/subarray"), index=w648) -> (w650:u16[])
                }
                frame 7 {
                  n369 = local write "RewCalib_Trig_R"(FALSE ("RewCalib_Trig_L")) -> ()
                  n370 = Replace Array Subset(array=w654, new element=u16 0 ("new element/subarray"), index=w653) -> (w655:u16[])
                }
              }
            }
            frame "DispenseWater_pre" {
              w691 = u16 0 ("t")
              w734 = u16 0 ("new element/subarray")
              # "just trust me on this one"
              # "RewCalib\nOnOff"
              # "RewCalib\nOnOff"
              # "nCycle"
              # "Solenoid__R"
              # "Tdelay"
              # "delay"
              # "nCycle"
              # "Solenoid__L"
              # "Tdelay"
              # "delay"
              # "Solenoid__R"
              # "count"
              # "Solenoid_Tcycle_R"
              # "Solenoid_Tcycle_L"
              # "Solenoid__L"
              # "count"
              n371 = call "myRIO_BRig_RT_dataMTrig_Solenoid_RewCalib_OnOff__L.vi"() -> ("output_Solenoid_RewCalib_OnOff__L"=w698:i32)  [unwired: 11 in]
              n372 = call "myRIO_BRig_RT_dataMTrig_Solenoid_N__L.vi"() -> ("output_Solenoid_N__L"=w689:i32)  [unwired: 11 in]
              n373 = call "myRIO_BRig_RT_dataMTrig_Solenoid_delay__L.vi"() -> ("output_Solenoid_delay__L"=w732:i32)  [unwired: 11 in]
              n374 = call "myRIO_BRig_RT_dataMTrig_Solenoid_Tdelay__L.vi"() -> ("output_Solenoid_Tdelay__L"=w731:i32)  [unwired: 11 in]
              n375 = call "myRIO_BRig_RT_dataMTrig_Solenoid_N__R.vi"() -> ("output_Solenoid_N__R"=w687:i32)  [unwired: 11 in]
              n376 = call "myRIO_BRig_RT_dataMTrig_Solenoid_delay__R.vi"() -> ("output_Solenoid_delay__R"=w721:i32)  [unwired: 11 in]
              n377 = call "myRIO_BRig_RT_dataMTrig_Solenoid_Tdelay__R.vi"() -> ("output_Solenoid_Tdelay__R"=w720:i32)  [unwired: 11 in]
              n378 = call "myRIO_BRig_RT_dataMTrig_Solenoid_RewCalib_OnOff__R.vi"() -> ("output_Solenoid_RewCalib_OnOff__R"=w694:i32)  [unwired: 11 in]
              n379 = Index Array(array=w733, index #1=w689, index #2=w732, index #3=w731, index #4=w687, index #5=w721, index #6=w720, index #7=w698, index #8=w694) -> (element #1=w690:u16, element #2=w730:u16, element #3=w725:u16, element #4=w693:u16, element #5=w715:u16, element #6=w714:u16, element #7=w699:u16, element #8=w696:u16)
              n380 = Equal To 0?(x=w730) -> (x = 0?=w729:bool)
              n381 = Equal To 0?(x=w715) -> (x = 0?=w719:bool)
              n382 = local read "RewCalib_Trig_L"() -> (w710:bool)
              n383 = local read "RewCalib_Trig_R"() -> (w705:bool)
              n384 = Not Equal To 0?(x=w690) -> (x != 0?=w728:bool)
              n385 = Not Equal To 0?(x=w693) -> (x != 0?=w718:bool)
              n386 = local read "MTrig_Solenoid_Tcycle__L"() -> (w727:u16)
              n387 = local read "MTrig_Solenoid_Tcycle__R"() -> (w713:u16)
              n388 = Not Equal To 0?(x=w699) -> (x != 0?=w709:bool)
              n389 = Not Equal To 0?(x=w696) -> (x != 0?=w707:bool)
              n390 = Not(x=w710) -> (.not. x?=w708:bool)
              n391 = Not(x=w705) -> (.not. x?=w706:bool)
              n392 = And(x=w709, y=w708) -> (x .and. y?=w704:bool)
              n393 = And(x=w707, y=w706) -> (x .and. y?=w703:bool)
              n394 = call "myRIO_BRig_RT_dataMTrig_Solenoid_c__L.vi"() -> ("output_Solenoid_c__L"=w736:i32)  [unwired: 11 in]
              n395 = call "myRIO_BRig_RT_dataMTrig_Solenoid_c__R.vi"() -> ("output_Solenoid_c__R"=w735:i32)  [unwired: 11 in]
              n396 = Select(t=w727, s=w728, f=u16 0) -> (s? t:f=w724:u16)
              n397 = Or(x=w704, y=w703) -> (x .or. y?=w692:bool)
              n398 = Select(t=w713, s=w718, f=u16 0) -> (s? t:f=w716:u16)
              n399 = Select(t=w724, s=w729, f=w725) -> (s? t:f=w722:u16)
              n400 = Select(t=w716, s=w719, f=w714) -> (s? t:f=w711:u16)
              n401 = call "myRIO_BRig_RT_dataMTrig_Solenoid_Tcycle__L.vi"() -> ("output_Solenoid_Tcycle__L"=w723:i32)  [unwired: 11 in]
              n402 = call "myRIO_BRig_RT_dataMTrig_Solenoid_Tcycle__R.vi"() -> ("output_Solenoid_Tcycle__R"=w712:i32)  [unwired: 11 in]
              n403 = Select(t=w691, s=w692, f=w690) -> (s? t:f=w688:u16)
              n404 = Select(t=w691, s=w692, f=w693) -> (s? t:f=w686:u16)
              n405 = Select(t=myRIO_BRig_RT__Case_NonExp_stateList."Idle" ("Enum"), s=w692, f=myRIO_BRig_RT__Case_NonExp_stateList."DispenseWater" ("Enum")) -> (s? t:f=w700:T1)
              n406 = Select(t=w691, s=w692, f=w699) -> (s? t:f=w697:u16)
              n407 = Select(t=w691, s=w692, f=w696) -> (s? t:f=w695:u16)
              n408 = Replace Array Subset(array=w733, new element #1=w734, index #1=w736, new element #2=w734, index #2=w735, new element #3=w722, index #3=w723, new element #4=w711, index #4=w712, new element #5=w697, index #5=w698, new element #6=w695, index #6=w694, new element #7=w688, index #7=w689, new element #8=w686, index #8=w687) -> (w737:u16[])
            }
            frame "DispenseWater" {
              # "D"
              # "C"
              # "B"
              # "A"
              # "(A) Add COUNT and INCREMENT\n(B) Is (A) smaller than Tcycle?\n(C) Are we dispensing water or in the delay phase?\n(D) If (A) is smaller than Tcycle   AND   if we are dispensing water\n      then send TRUE to solenoid"
              # "delay"
              # "Tcycle"
              # "Solenoid__R"
              # "count"
              # "delay"
              # "Tcycle"
              # "Solenoid__L"
              # "count"
              n409 = To Unsigned Word Integer(number=w768) -> (unsigned 16bit integer=w750:u16)
              n410 = call "myRIO_BRig_RT_dataMTrig_Solenoid_delay__R.vi"() -> ("output_Solenoid_delay__R"=w754:i32)  [unwired: 11 in]
              n411 = call "myRIO_BRig_RT_dataMTrig_Solenoid_c__R.vi"() -> ("output_Solenoid_c__R"=w753:i32)  [unwired: 11 in]
              n412 = call "myRIO_BRig_RT_dataMTrig_Solenoid_Tcycle__R.vi"() -> ("output_Solenoid_Tcycle__R"=w755:i32)  [unwired: 11 in]
              n413 = call "myRIO_BRig_RT_dataMTrig_Solenoid_delay__L.vi"() -> ("output_Solenoid_delay__L"=w770:i32)  [unwired: 11 in]
              n414 = call "myRIO_BRig_RT_dataMTrig_Solenoid_c__L.vi"() -> ("output_Solenoid_c__L"=w762:i32)  [unwired: 11 in]
              n415 = call "myRIO_BRig_RT_dataMTrig_Solenoid_Tcycle__L.vi"() -> ("output_Solenoid_Tcycle__L"=w771:i32)  [unwired: 11 in]
              n416 = Index Array(array=w764, index #1=w762, index #2=w771, index #3=w770, index #4=w753, index #5=w755, index #6=w754) -> (element #1=w769:u16, element #2=w759:u16, element #3=w767:u16, element #4=w749:u16, element #5=w746:u16, element #6=w745:u16)
              n417 = Add(x=w769, y=w750) -> (x+y=w760:u16)
              n418 = Add(x=w749, y=w750) -> (x+y=w751:u16)
              n419 = Less?(x=w760, y=w759) -> (x < y?=w743:bool)
              n420 = Equal To 0?(x=w767) -> (x = 0?=w766:bool)
              n421 = Less?(x=w751, y=w746) -> (x < y?=w744:bool)
              n422 = Equal To 0?(x=w745) -> (x = 0?=w752:bool)
              n423 = And(x=w743, y=w766) -> (x .and. y?=w765:bool)
              n424 = Or(x=w743, y=w744) -> (x .or. y?=w742:bool)
              n425 = And(x=w744, y=w752) -> (x .and. y?=w747:bool)
              n426 = Select(t=w760, s=w743, f=w759) -> (s? t:f=w761:u16)
              n427 = Select(t=w751, s=w744, f=w746) -> (s? t:f=w748:u16)
              n428 = Replace Array Subset(array=w764, new element #1=w761, index #1=w762, new element #2=w748, index #2=w753) -> (w763:u16[])
              n429 = Select(t=w758, s=w742, f=myRIO_BRig_RT__Case_NonExp_stateList."DispenseWater_post" ("Enum")) -> (s? t:f=w756:T1)
            }
            frame "DispenseWater_post" {
              # "nCycle"
              # "delay"
              # "Solenoid__R"
              # "nCycle"
              # "delay"
              # "Solenoid__L"
              n430 = call "myRIO_BRig_RT_dataMTrig_Solenoid_N__L.vi"() -> ("output_Solenoid_N__L"=w793:i32)  [unwired: 11 in]
              n431 = call "myRIO_BRig_RT_dataMTrig_Solenoid_delay__L.vi"() -> ("output_Solenoid_delay__L"=w792:i32)  [unwired: 11 in]
              n432 = call "myRIO_BRig_RT_dataMTrig_Solenoid_N__R.vi"() -> ("output_Solenoid_N__R"=w789:i32)  [unwired: 11 in]
              n433 = call "myRIO_BRig_RT_dataMTrig_Solenoid_delay__R.vi"() -> ("output_Solenoid_delay__R"=w788:i32)  [unwired: 11 in]
              n434 = Index Array(array=w795, index #1=w793, index #2=w792, index #3=w789, index #4=w788) -> (element #1=w797:u16, element #2=w796:u16, element #3=w780:u16, element #4=w782:u16)
              n435 = Not Equal To 0?(x=w797) -> (x != 0?=w798:bool)
              n436 = Not Equal To 0?(x=w780) -> (x != 0?=w781:bool)
              n437 = case shown="True" w781 {
                selector: w781 -> [_ w806]
                tunnel: w780 -> [w804 w812]
                tunnel: w782 -> [_ w813]
                tunnel: [w804 w810] -> w779
                tunnel: [u16 0 w809] -> w778
                tunnel: [_ w806] -> w777
                frame False {
                }
                frame True {
                  n438 = Equal To 0?(x=w813) -> (x = 0?=w805:bool)
                  n439 = Decrement(x=w812) -> (x-1=w811:u16)
                  n440 = Select(t=w811, s=w805, f=w812) -> (s? t:f=w810:u16)
                  n441 = Select(t=u16 1, s=w805, f=u16 0) -> (s? t:f=w809:u16)
                }
              }
              n442 = case shown="True" w798 {
                selector: w798 -> [_ w817]
                tunnel: w797 -> [w815 w823]
                tunnel: w796 -> [_ w824]
                tunnel: [w815 w821] -> w791
                tunnel: [u16 0 w820] -> w790
                tunnel: [_ w817] -> w787
                frame False {
                }
                frame True {
                  n443 = Equal To 0?(x=w824) -> (x = 0?=w816:bool)
                  n444 = Decrement(x=w823) -> (x-1=w822:u16)
                  n445 = Select(t=w822, s=w816, f=w823) -> (s? t:f=w821:u16)
                  n446 = Select(t=u16 1, s=w816, f=u16 0) -> (s? t:f=w820:u16)
                }
              }
              n447 = Or(x=w787, y=w777) -> (x .or. y?=w786:bool)
              n448 = Replace Array Subset(array=w795, new element #1=w791, index #1=w793, new element #2=w790, index #2=w792, new element #3=w779, index #3=w789, new element #4=w778, index #4=w788) -> (w794:u16[])
              n449 = Select(t=myRIO_BRig_RT__Case_NonExp_stateList."DispenseWater_pre" ("Enum"), s=w786, f=myRIO_BRig_RT__Case_NonExp_stateList."Idle" ("Enum")) -> (s? t:f=w783:T1)
            }
            frame "TestConnection" {
              n450 = local read "Host Password"() -> (w835:string)
              n451 = local read "Host UserName"() -> (w836:string)
              n452 = call "myRIO_BRig_RT_comm_webdav_testConnect.vi"("input_password"=w835, "input_username"=w836) -> ("output_Iconnected"=w833:bool)  [unwired: 9 in]
              n453 = Select(t="Connection accepted!" ("message"), s=w833, f="Error!") -> (s? t:f=w831:string)
              n454 = One Button Dialog(message=w831) -> ()  [unwired: 1 in, 1 out]
            }
            frame "SendData" {
              n455 = local read "Host Filename Prefix"() -> (w838:string)
              n456 = local read "Host Password"() -> (w839:string)
              n457 = local read "Host UserName"() -> (w840:string)
              n458 = call "myRIO_BRig_RT_comm_webdav_sendData_all.vi"("Host Filename Prefix"=w838, "Host Password"=w839, "Host UserName"=w840) -> ()  [unwired: 9 in]
            }
            frame "End" {
            }
          }
          n459 = local read "MTrig_Audio_trig__R"() -> (w81:bool)
          n460 = local read "MTrig_Audio_trig__L"() -> (w80:bool)
          n461 = local read "START"() -> (w76:bool)
          n462 = local read "STOP_abort"() -> (w75:bool)
          n463 = local read "MTrig_Laser_trig"() -> (w82:bool)
          n464 = call "myRIO_BRig_RT_dataMTrig_main__v2.vi"("input_dataMTrig"=w84, "input_Audio_trig_L"=w80, "input_Audio_trig_R"=w81, "input_Laser_trig"=w82) -> ("output_dataMTrig"=w83:u16[], "output_Audio_L"=w60:bool, "output_Audio_R"=w71:bool, "output_Laser"=w63:bool)  [unwired: 12 in]
          n465 = Or(x=w76, y=w75) -> (x .or. y?=w74:bool)
          n466 = local read "A6"() -> (w53:bool)
          n467 = Select(t=myRIO_BRig_RT__Case_NonExp_stateList."End" ("Enum"), s=w74, f=w73) -> (s? t:f=w72:T1)
          n468 = Or(x=w81, y=w82) -> (x .or. y?=w79:bool)
          n469 = Or(x=w79, y=w80) -> (x .or. y?=w78:bool)
          n470 = case shown="True" w78 {
            frame False {
            }
            frame True {
              w109 = FALSE
              n471 = local write "MTrig_Audio_trig__R"(w109) -> ()
              n472 = local write "MTrig_Audio_trig__L"(w109) -> ()
              n473 = local write "MTrig_Laser_trig"(w109) -> ()
            }
          }
          n474 = xnode "Read/Write Control"("FPGA VI Reference In"=w101, "error in"=w99, "A6_Act"=w53, "A1_SR"=w85, "A3_SL"=w86, "audioTrigger_L"=w60, "audioAmp_L"=w90, "audioFreq_L_Hz"=w89, "audioTrigger_R"=w71, "audioAmp_R"=w88, "audioFreq_R_Hz"=w87, "laserResponse_reward_LED"="laserResponse_reward_LED", "laserResponse_wrong_LED"="laserResponse_wrong_LED", "laserResponse_reward"="laserResponse_reward", "laserResponse_wrong"="laserResponse_wrong", "SelectionState"="SelectionState", "ignoreWrong"="ignoreWrong", "Left(F)_or_Right(T)"="Left(F)_or_Right(T)", "laserMTrig"=w63, "tCycle_laser_rew"="tCycle_laser_rew", "tDelay_laser_rew"="tDelay_laser_rew", "tCycle_laser_wro"="tCycle_laser_wro", "tDelay_laser_wro"="tDelay_laser_wro") -> ("FPGA VI Reference Out"=w100:refnum<k20>, "error out"=w98:errorcluster, "SelectReward"=→"SelectReward":bool, "SelectWrong"=→"SelectWrong":bool)
          n475 = node-c288() -> ()  [unwired: 1 in, 1 out]
          "cState_NonExp" <- w97
        }
        n476 = node-c288(w48) -> ()  [unwired: 1 out]
        n477 = flat-sequence {
          tunnel: w41 -> [w52]
          tunnel: [w52] -> w40
          tunnel: w39 -> [w51]
          tunnel: [w51] -> w38
          frame #0 {
            w50 = FALSE
            n478 = local write "STOP_endBlock"(w50) -> ()
            n479 = local write "STOP_endTrial"(w50) -> ()
          }
        }
      }
      frame True {
        w865 = FALSE ("SelectionState")
        w870 = u16 0 ("idxDataBlock")
        w872 = u16 100 ("new element/subarray")
        w873 = u16 100 ("new element/subarray")
        w893 = T6 refnum items=["Session NI_WebDAV"] ("output_hSession")
        w902 = FALSE
        w903 = u16 0
        w864 = FALSE
        # "audio__L\naudio__R"
        # "Audio params"
        # "nRewards"
        # "idxDataBlock"
        # "Solenoid_Tdelay_R"
        # "Solenoid_Tdelay_L"
        # "RewCalib_N__R"
        # "RewCalib_N__L"
        # "Save dataLick to file\nSend file to Host\nSave dataMTrig\nSend file to Host\nDisconnect"
        # "dataTrial"
        # "dataTrial"
        # "Solenoid_Tcycle_R"
        # "Solenoid_Tcycle_L"
        # "Laser_Tcycle"
        # "Audio_Tcycle_R"
        # "Audio_Tcycle_L"
        # "dataLick"
        # "dataLC"
        # "dataLC"
        # "dataBlock"
        # "dataBlock"
        # "dataMTrig"
        # "dataMTrig"
        # "dataExp"
        # "dataCurrent"
        # "dataExp"
        # "dataCurrent"
        # "spout"
        # "state"
        n480 = call "myRIO_BRig_RT_dataMTrig_Solenoid_Tcycle__L.vi"() -> ("output_Solenoid_Tcycle__L"=w899:i32)  [unwired: 11 in]
        n481 = call "myRIO_BRig_RT_dataMTrig_Solenoid_Tcycle__R.vi"() -> ("output_Solenoid_Tcycle__R"=w898:i32)  [unwired: 11 in]
        n482 = call "myRIO_BRig_RT_dataMTrig_Audio_Tcycle__L.vi"() -> ("output_Audio_Tcycle__L"=w897:i32)  [unwired: 11 in]
        n483 = call "myRIO_BRig_RT_dataMTrig_Audio_Tcycle__R.vi"() -> ("output_Audio_Tcycle__R"=w896:i32)  [unwired: 11 in]
        n484 = call "myRIO_BRig_RT_dataMTrig_Laser_Tcycle.vi"() -> ("output_Laser_Tcycle"=w895:i32)  [unwired: 11 in]
        n485 = local read "MTrig_Solenoid_Tcycle__L"() -> (w878:u16)
        n486 = local read "MTrig_Solenoid_Tcycle__R"() -> (w877:u16)
        n487 = local read "Tcycle_Reward_L"() -> (w874:u16)
        n488 = local read "Tcycle_Reward_R"() -> (w875:u16)
        n489 = local read "MTrig_Laser_Tcycle"() -> (w876:u16)
        n490 = call "myRIO_BRig_RT_dataMTrig_Solenoid_RewCalib_nCycle__L.vi"() -> ("output_Solenoid_RewCalib_nCycle__L"=w881:i32)  [unwired: 11 in]
        n491 = call "myRIO_BRig_RT_dataMTrig_Solenoid_Tdelay__L.vi"() -> ("output_Solenoid_Tdelay__L"=w883:i32)  [unwired: 11 in]
        n492 = call "myRIO_BRig_RT_dataMTrig_Solenoid_RewCalib_nCycle__R.vi"() -> ("output_Solenoid_RewCalib_nCycle__R"=w882:i32)  [unwired: 11 in]
        n493 = call "myRIO_BRig_RT_dataMTrig_Solenoid_Tdelay__R.vi"() -> ("output_Solenoid_Tdelay__R"=w884:i32)  [unwired: 11 in]
        n494 = call "myRIO_BRig_RT_dataLick_init.vi"() -> ("output_dataLick"=w905:u16[][])  [unwired: 11 in]
        n495 = call "myRIO_BRig_RT_dataCurrent_init.vi"() -> ("output_dataCurrent"=w912:u16[])  [unwired: 11 in]
        n496 = call "myRIO_BRig_RT_dataExp_init.vi"() -> ("output_dataExp"=w911:u16[])  [unwired: 11 in]
        n497 = call "myRIO_BRig_RT_dataMTrig_init.vi"() -> ("output_dataMTrig"=w901:u16[])  [unwired: 5 in]
        n498 = call "myRIO_BRig_RT_dataLC_init.vi"() -> ("output_dataLC"=w909:u16[])  [unwired: 11 in]
        n499 = call "myRIO_BRig_RT_dataBlock_init.vi"() -> ("output_dataBlock"=w910:u16[][])  [unwired: 11 in]
        n500 = call "myRIO_BRig_RT_dataTrial_init.vi"() -> ("output_dataTrial"=w894:u16[][])  [unwired: 11 in]
        n501 = xnode "Read/Write Control"("FPGA VI Reference In"=w866, "error in"=w867, "SelectionState"=w865, "laserResponse_reward"=w865, "laserResponse_wrong"=w865, "laserResponse_reward_LED"=w865, "laserResponse_wrong_LED"=w865, "Left(F)_or_Right(T)"=w865, "ignoreWrong"=w865, "SelectionState"=w865, "laser_Npeak"="laser_Npeak", "laser_Nvalley"="laser_Nvalley", "AO0"="AO0") -> ("FPGA VI Reference Out"=w868:refnum<k20>, "error out"=w869:errorcluster)
        n502 = Replace Array Subset(array=w901, new element #1=w873, index #1=w881, new element #2=w873, index #2=w882, new element #3=w872, index #3=w883, new element #4=w872, index #4=w884, new element #5=w878, index #5=w899, new element #6=w877, index #6=w898, new element #7=w874, index #7=w897, new element #8=w875, index #8=w896, new element #9=w876, index #9=w895) -> (w900:u16[])
        n503 = Get Date/Time In Seconds() -> (seconds since 1Jan1904=w880:timestamp)
        n504 = To Double Precision Float(number=w880) -> (double precision float=w879:dbl)
        n505 = node-c288() -> (w920:T3)  [unwired: 4 in]
        n506 = timed-loop {
          timing: w920 -> [_]
          timing-out: [_] -> w919
          shift-right: [w998] -> _
          shift-left: myRIO_BRig_RT__Case_Exp_stateList."Start1" ("Enum") -> [w1029]
          shift-right: [w1050] -> _
          shift-left: enum16{"Left", "Right"}."Left" -> [w1052]
          tunnel: w868 -> [w1049]
          tunnel: w869 -> [w1048]
          shift-right: [w1043] -> _
          shift-left: w917 -> [w1047]
          shift-right: [w1042] -> _
          shift-left: w916 -> [w1046]
          tunnel: [w1023] -> w914
          tunnel: [w1024] -> w915
          shift-right: [w1025] -> w885
          shift-left: w912 -> [w990]
          shift-right: [w1041] -> _
          shift-left: w911 -> [w985]
          shift-right: [w1012] -> w889
          shift-left: w900 -> [w1013]
          shift-right: [w1039] -> _
          shift-left: w910 -> [w1040]
          shift-right: [w1037] -> _
          shift-left: w909 -> [w1038]
          shift-right: [w970] -> _
          shift-left: w864 -> [w1036]
          shift-right: [w1027] -> w891
          shift-left: w905 -> [w1028]
          shift-right: [w1014] -> _
          shift-left: w903 -> [w1022]
          shift-right: [w982] -> _
          shift-left: w903 -> [w1021]
          shift-right: [w1015] -> _
          shift-left: w903 -> [w1020]
          shift-right: [w1016] -> _
          shift-left: w903 -> [w1019]
          shift-right: [w983] -> _
          shift-left: w902 -> [w1017]
          shift-right: [w984] -> _
          shift-left: w902 -> [w1018]
          shift-right: [w996] -> _
          shift-left: w894 -> [w997]
          shift-right: [w995] -> w887
          shift-left: w893 -> [w993]
          shift-right: [w994] -> w888
          shift-left: FALSE ("output_Iconnected") -> [w992]
          tunnel: "Host Filename Prefix" -> [w991]
          tunnel: [w991] -> w886
          shift-right: [w965] -> _
          shift-left: w864 -> [w989]
          tunnel: w879 -> [w986]
          shift-right: [w980] -> _
          shift-left: 0 ("idxDataBlock") -> [w981]
          shift-right: [w977] -> _
          shift-left: w870 -> [w979]
          shift-right: [w976] -> _
          shift-left: w870 -> [w978]
          shift-right: [w964] -> _
          shift-left: w864 -> [w971]
          shift-right: [w967] -> _
          shift-left: w864 -> [w969]
          shift-right: [w966] -> _
          shift-left: w864 -> [w968]
          shift-right: [w957] -> _
          shift-left: w864 -> [w958]
          stop <- w1035 stop-if-true
          # "Laser"
          # "Audio R"
          # "Audio L"
          # "Solenoid R"
          # "Solenoid L"
          # "manual triggering"
          # "dataTrial"
          # "dataBlock"
          # "nRewards"
          # "laserOccurred"
          # "dataExp"
          # "dataCurrent"
          # "audio__L\naudio__R"
          # "time stamp"
          # "Audio params"
          # "nRewards"
          # "idxDataBlock"
          # "idxDataBlock"
          # "activate"
          # "audio__L\naudio__R"
          # "amp__R\nfreq__R"
          # "amp__L\nfreq__L"
          # "dataLC"
          # "solenoid__R"
          # "solenoid__L"
          # "Did a lick occur?"
          # "Update lick counter"
          # "spout"
          # "spout"
          # "state"
          # "state"
          n507 = node-c288() -> ()  [unwired: 1 in, 1 out]
          n508 = local read "MTrig_Solenoid_trig__L"() -> (w1010:bool)
          n509 = local read "MTrig_Solenoid_trig__R"() -> (w1009:bool)
          n510 = local read "MTrig_Audio_trig__L"() -> (w1008:bool)
          n511 = local read "MTrig_Audio_trig__R"() -> (w1007:bool)
          n512 = xnode "Read/Write Control"("FPGA VI Reference In"=w1049, "error in"=w1048) -> ("FPGA VI Reference Out"=w975:refnum<k20>, "error out"=w974:errorcluster, "A2_LickL"=w1043:u32, "A4_LickR"=w1042:u32)
          "A2" <- w1043
          "A4" <- w1042
          n513 = local read "MTrig_Laser_trig"() -> (w1006:bool)
          n514 = Greater?(x=w1043, y=w1047) -> (0:w1045:bool)
          n515 = Greater?(x=w1042, y=w1046) -> (0:w1044:bool)
          n516 = Or(x=w1045, y=w1044) -> (x .or. y?=w1051:bool)
          n517 = call "myRIO_BRig_RT_dataMTrig_main.vi"("input_dataMTrig"=w1013, "input_Solenoid_trig_L"=w1010, "input_Solenoid_trig_R"=w1009, "input_Audio_trig_L"=w1008, "input_Audio_trig_R"=w1007, "input_Laser_trig"=w1006) -> ("output_Laser"=w962:bool, "output_dataMTrig"=w1012:u16[], "output_Solenoid_L"=w1000:bool, "output_Solenoid_R"=w1002:bool, "output_Audio_L"=w1004:bool, "output_Audio_R"=w1005:bool)  [unwired: 8 in]
          n518 = Compound Arithmetic op=OR(w1010, w1009, w1008, w1007, w1006) -> (w1011:bool)
          n519 = case shown="True" w1011 {
            frame False {
            }
            frame True {
              w1053 = FALSE
              n520 = local write "MTrig_Solenoid_trig__L"(w1053) -> ()
              n521 = local write "MTrig_Solenoid_trig__R"(w1053) -> ()
              n522 = local write "MTrig_Audio_trig__L"(w1053) -> ()
              n523 = local write "MTrig_Audio_trig__R"(w1053) -> ()
              n524 = local write "MTrig_Laser_trig"(w1053) -> ()
            }
          }
          n525 = case shown="\"saveSettings5_LC_Cue\"" w1029 {
            selector: w1029 -> [_ _ _ _ _ _ _ _ _ _ _ _ _ _ _ _ _ _ w1652 _ w1720 _ _ _ _ _ w1858 _ w1934 _ _ _ _ _ w2066 _ w2143 _ w2207 _ w2251 _ _ w2318 _ _ _ _ _ w2486 _ _ _ _ _ _ _ _ _ _ _ _]
            tunnel: [myRIO_BRig_RT__Case_Exp_stateList."Start2" ("Enum") myRIO_BRig_RT__Case_Exp_stateList."Start3" ("Enum") myRIO_BRig_RT__Case_Exp_stateList."saveSettings1" ("Enum") myRIO_BRig_RT__Case_Exp_stateList."saveSettings2" ("Enum") myRIO_BRig_RT__Case_Exp_stateList."saveSettings3" ("Enum") myRIO_BRig_RT__Case_Exp_stateList."saveSettings4_LC_ENL" ("Enum") myRIO_BRig_RT__Case_Exp_stateList."saveSettings5_LC_Cue" ("Enum") myRIO_BRig_RT__Case_Exp_stateList."saveSettings6_LC_Other" ("Enum") myRIO_BRig_RT__Case_Exp_stateList."setSettings_Audio" ("Enum") myRIO_BRig_RT__Case_Exp_stateList."commConnect" ("Enum") w1449 myRIO_BRig_RT__Case_Exp_stateList."initTrial" ("Enum") w1489 myRIO_BRig_RT__Case_Exp_stateList."initTrial3" ("Enum") myRIO_BRig_RT__Case_Exp_stateList."initTrial_LC_ENL1" ("Enum") myRIO_BRig_RT__Case_Exp_stateList."initTrial_LC_Cue1" ("Enum") myRIO_BRig_RT__Case_Exp_stateList."ENL1_pre" ("Enum") w1611 w1649 myRIO_BRig_RT__Case_Exp_stateList."ENL1Penalty" ("Enum") w1721 myRIO_BRig_RT__Case_Exp_stateList."endExp" ("Enum") myRIO_BRig_RT__Case_Exp_stateList."endExp" ("Enum") myRIO_BRig_RT__Case_Exp_stateList."endExp" ("Enum") myRIO_BRig_RT__Case_Exp_stateList."endExp" ("Enum") w1814 w1857 myRIO_BRig_RT__Case_Exp_stateList."Cue1Penalty" ("Enum") w1932 myRIO_BRig_RT__Case_Exp_stateList."endExp" ("Enum") myRIO_BRig_RT__Case_Exp_stateList."endExp" ("Enum") myRIO_BRig_RT__Case_Exp_stateList."endExp" ("Enum") myRIO_BRig_RT__Case_Exp_stateList."endExp" ("Enum") w2020 w2074 myRIO_BRig_RT__Case_Exp_stateList."SelectReward" ("Enum") w2144 myRIO_BRig_RT__Case_Exp_stateList."SelectRewardPost" ("Enum") w2208 myRIO_BRig_RT__Case_Exp_stateList."SelectWrong" ("Enum") w2247 myRIO_BRig_RT__Case_Exp_stateList."endTrial1" ("Enum") myRIO_BRig_RT__Case_Exp_stateList."SelectTimeout" ("Enum") w2320 myRIO_BRig_RT__Case_Exp_stateList."endTrial1" ("Enum") myRIO_BRig_RT__Case_Exp_stateList."endTrial2" ("Enum") myRIO_BRig_RT__Case_Exp_stateList."saveData_dataBlock" ("Enum") w2399 w2469 w2486 myRIO_BRig_RT__Case_Exp_stateList."initBlock" ("Enum") w2513 myRIO_BRig_RT__Case_Exp_stateList."commUpload_dataCurrent" ("Enum") myRIO_BRig_RT__Case_Exp_stateList."commUpload_dataExp" ("Enum") myRIO_BRig_RT__Case_Exp_stateList."commUpload_dataLC" ("Enum") myRIO_BRig_RT__Case_Exp_stateList."commUpload_dataTrial" ("Enum") myRIO_BRig_RT__Case_Exp_stateList."endTrial3" ("Enum") myRIO_BRig_RT__Case_Exp_stateList."saveData_dataCurrent" ("Enum") myRIO_BRig_RT__Case_Exp_stateList."saveData_dataExp" ("Enum") myRIO_BRig_RT__Case_Exp_stateList."saveData_dataLC" ("Enum") myRIO_BRig_RT__Case_Exp_stateList."saveData_dataTrial" ("Enum") myRIO_BRig_RT__Case_Exp_stateList."commUpload_pre" ("Enum")] -> w998
            tunnel: [w1079 w1099 w1121 w1178 w1222 w1249 w1301 w1353 w1397 w1421 w1425 w1457 w1490 w1513 w1534 w1561 w1586 w1627 w1665 w1698 w1725 w1741 w1763 w1782 w1801 w1833 w1879 w1905 w1931 w1952 w1973 w1992 w2011 w2031 w2092 w2117 w2140 w2155 w2205 w2229 w2262 w2283 w2299 w2331 w2354 w2366 w2385 w2423 w2442 w2485 w2502 w2516 w2550 w2571 w2592 w2613 w2634 w2662 w2682 w2709 w2729 w2754] -> w1050
            tunnel: w1052 -> [w1079 w1099 w1121 w1178 w1222 w1249 w1301 w1353 w1397 w1421 w1448 w1457 w1490 w1513 w1534 w1561 w1586 w1627 w1665 w1698 w1725 w1741 w1763 w1782 w1801 w1833 w1879 w1905 w1931 w1952 w1973 w1992 w2011 w2031 w2092 w2117 w2140 w2155 w2205 w2229 w2262 w2283 w2299 w2331 w2354 w2366 w2385 w2423 w2442 w2485 w2502 w2516 w2550 w2571 w2592 w2613 w2634 w2662 w2682 w2709 w2729 w2754]
            tunnel: w1051 -> [w1082 w1102 w1118 w1181 w1225 w1252 w1304 w1356 w1400 w1424 w1442 w1468 w1491 w1531 w1551 w1574 w1599 w1614 w1646 w1701 w1728 w1747 w1766 w1785 w1804 w1813 w1856 w1913 w1938 w1957 w1976 w1995 w2014 w2029 w2090 w2127 w2151 w2186 w2213 w2240 w2265 w2282 w2311 w2336 w2351 w2374 w2384 w2434 w2468 w2489 w2499 w2525 w2553 w2574 w2595 w2616 w2637 w2665 w2685 w2712 w2732 w2757]
            tunnel: w1045 -> [w1081 w1101 w1119 w1180 w1224 w1251 w1303 w1355 w1399 w1423 w1441 w1467 w1492 w1530 w1552 w1575 w1600 w1637 w1667 w1700 w1727 w1746 w1765 w1784 w1803 w1847 w1880 w1912 w1937 w1956 w1975 w1994 w2013 w2030 w2089 w2126 w2150 w2185 w2212 w2239 w2264 w2281 w2310 w2335 w2352 w2375 w2383 w2433 w2467 w2488 w2500 w2526 w2552 w2573 w2594 w2615 w2636 w2664 w2684 w2711 w2731 w2756]
            tunnel: w1044 -> [w1080 w1100 w1120 w1179 w1223 w1250 w1302 w1354 w1398 w1422 w1440 w1466 w1493 w1529 w1553 w1576 w1601 w1636 w1666 w1699 w1726 w1745 w1764 w1783 w1802 w1846 w1881 w1911 w1936 w1955 w1974 w1993 w2012 w2049 w2093 w2125 w2149 w2184 w2211 w2238 w2263 w2280 w2309 w2334 w2353 w2376 w2382 w2432 w2466 w2487 w2501 w2527 w2551 w2572 w2593 w2614 w2635 w2663 w2683 w2710 w2730 w2755]
            tunnel: [w1082 w1102 w1118 w1181 w1225 w1252 w1304 w1356 w1400 w1424 w1442 w1468 w1491 w1531 w1551 w1574 w1599 w1614 w1646 w1701 w1728 w1747 w1766 w1785 w1804 w1813 w1856 w1913 w1938 w1957 w1976 w1995 w2014 w2029 w2090 w2127 w2151 w2186 w2213 w2240 w2265 w2282 w2311 w2336 w2351 w2374 w2384 w2434 w2468 w2489 w2499 w2525 w2553 w2574 w2595 w2616 w2637 w2665 w2685 w2712 w2732 w2757] -> w1032
            tunnel: [w1081 w1101 w1119 w1180 w1224 w1251 w1303 w1355 w1399 w1423 w1441 w1467 w1492 w1530 w1552 w1575 w1600 w1637 w1667 w1700 w1727 w1746 w1765 w1784 w1803 w1847 w1880 w1912 w1937 w1956 w1975 w1994 w2013 w2030 w2089 w2126 w2150 w2185 w2212 w2239 w2264 w2281 w2310 w2335 w2352 w2375 w2383 w2433 w2467 w2488 w2500 w2526 w2552 w2573 w2594 w2615 w2636 w2664 w2684 w2711 w2731 w2756] -> w1031
            tunnel: [w1080 w1100 w1120 w1179 w1223 w1250 w1302 w1354 w1398 w1422 w1440 w1466 w1493 w1529 w1553 w1576 w1601 w1636 w1666 w1699 w1726 w1745 w1764 w1783 w1802 w1846 w1881 w1911 w1936 w1955 w1974 w1993 w2012 w2049 w2093 w2125 w2149 w2184 w2211 w2238 w2263 w2280 w2309 w2334 w2353 w2376 w2382 w2432 w2466 w2487 w2501 w2527 w2551 w2572 w2593 w2614 w2635 w2663 w2683 w2710 w2730 w2755] -> w1030
            tunnel: w990 -> [w1078 w1098 w1117 w1139 w1198 w1248 w1300 w1352 w1396 w1419 w1447 w1456 w1488 w1502 w1535 w1558 w1585 w1626 w1651 w1692 w1724 w1742 w1762 w1781 w1800 w1817 w1876 w1904 w1935 w1953 w1972 w1991 w2010 w2040 w2070 w2109 w2146 w2157 w2210 w2230 w2261 w2279 w2300 w2333 w2350 w2363 w2387 w2403 w2440 w2484 w2503 w2528 w2547 w2568 w2589 w2610 w2621 w2651 w2670 w2694 w2726 w2743]
            tunnel: w985 -> [w1077 w1097 w1116 w1176 w1220 w1245 w1298 w1350 w1394 w1412 w1446 w1465 w1487 w1510 w1539 w1564 w1589 w1629 w1664 w1691 w1722 w1744 w1761 w1780 w1799 w1835 w1878 w1902 w1930 w1954 w1971 w1990 w2009 w2042 w2091 w2123 w2148 w2178 w2206 w2231 w2259 w2278 w2302 w2330 w2349 w2373 w2390 w2402 w2459 w2483 w2504 w2529 w2546 w2567 w2588 w2609 w2622 w2659 w2679 w2690 w2725 w2751]
            tunnel: [w1078 w1098 w1117 w1139 w1198 w1248 w1300 w1352 w1396 w1419 w1431 w1456 w1476 w1502 w1535 w1557 w1584 w1630 w1650 w1693 w1723 w1742 w1762 w1781 w1800 w1842 w1875 w1903 w1933 w1953 w1972 w1991 w2010 w2043 w2065 w2124 w2145 w2179 w2209 w2232 w2260 w2279 w2303 w2332 w2350 w2362 w2386 w2403 w2438 w2484 w2503 w2528 w2547 w2568 w2589 w2610 w2621 w2651 w2670 w2694 w2726 w2743] -> w1026
            tunnel: [w1077 w1097 w1116 w1175 w1219 w1240 w1298 w1350 w1394 w1412 w1445 w1465 w1486 w1510 w1539 w1564 w1589 w1629 w1664 w1691 w1722 w1744 w1761 w1780 w1799 w1835 w1878 w1902 w1930 w1954 w1971 w1990 w2009 w2042 w2091 w2123 w2148 w2178 w2206 w2231 w2259 w2278 w2302 w2330 w2349 w2373 w2390 w2402 w2459 w2483 w2504 w2529 w2546 w2567 w2588 w2609 w2622 w2659 w2679 w2693 w2725 w2751] -> w1041
            tunnel: [_ _ _ _ _ _ _ _ _ _ _ _ _ _ _ _ _ _ _ _ _ _ _ _ _ _ _ _ _ _ _ _ _ _ _ _ w2138 _ _ _ _ _ _ _ _ _ _ _ _ _ _ _ _ _ _ _ _ _ _ _ _ _] -> w1001
            tunnel: [_ _ _ _ _ _ _ _ _ _ _ _ _ _ _ _ _ _ _ _ _ _ _ _ _ _ _ _ _ _ _ _ _ _ _ _ w2139 _ _ _ _ _ _ _ _ _ _ _ _ _ _ _ _ _ _ _ _ _ _ _ _ _] -> w1003
            tunnel: w1040 -> [w1075 w1095 w1114 w1141 w1200 w1246 w1299 w1351 w1395 w1417 w1443 w1458 w1484 w1522 w1549 w1554 w1581 w1628 w1663 w1688 w1718 w1743 w1759 w1778 w1797 w1841 w1877 w1901 w1928 w1950 w1969 w1988 w2007 w2041 w2087 w2115 w2147 w2159 w2203 w2228 w2256 w2276 w2301 w2329 w2347 w2365 w2392 w2430 w2451 w2481 w2506 w2531 w2544 w2565 w2586 w2607 w2631 w2645 w2672 w2700 w2719 w2745]
            tunnel: [w1075 w1095 w1114 w1141 w1200 w1246 w1299 w1351 w1395 w1417 w1443 w1455 w1484 w1522 w1549 w1554 w1581 w1628 w1663 w1688 w1718 w1743 w1759 w1778 w1797 w1841 w1877 w1901 w1928 w1950 w1969 w1988 w2007 w2041 w2087 w2115 w2147 w2158 w2203 w2228 w2256 w2276 w2301 w2329 w2347 w2364 w2392 w2430 w2451 w2481 w2506 w2531 w2544 w2565 w2586 w2607 w2631 w2645 w2672 w2700 w2719 w2745] -> w1039
            tunnel: w1038 -> [w1076 w1096 w1115 w1140 w1199 w1247 w1296 w1348 w1392 w1418 w1444 w1464 w1485 w1499 w1550 w1562 w1587 w1625 w1645 w1689 w1719 w1740 w1760 w1779 w1798 w1840 w1855 w1900 w1929 w1951 w1970 w1989 w2008 w2039 w2088 w2116 w2142 w2176 w2204 w2227 w2258 w2277 w2298 w2327 w2348 w2372 w2391 w2431 w2458 w2482 w2505 w2530 w2545 w2566 w2587 w2608 w2632 w2658 w2678 w2706 w2717 w2750]
            tunnel: [w1076 w1096 w1115 w1140 w1199 w1247 w1297 w1349 w1393 w1418 w1444 w1464 w1485 w1499 w1550 w1562 w1587 w1625 w1645 w1689 w1719 w1740 w1760 w1779 w1798 w1840 w1855 w1900 w1929 w1951 w1970 w1989 w2008 w2039 w2088 w2116 w2142 w2176 w2204 w2227 w2258 w2277 w2298 w2327 w2348 w2372 w2391 w2431 w2458 w2482 w2505 w2530 w2545 w2566 w2587 w2608 w2632 w2658 w2678 w2706 w2717 w2750] -> w1037
            tunnel: w1036 -> [_ _ _ _ _ _ _ _ _ _ _ _ _ _ _ _ _ w1610 w1644 w1673 w1707 _ _ _ _ _ w1848 w1882 w1916 _ _ _ _ _ _ _ w2141 _ _ _ w2257 _ _ w2328 _ _ _ _ _ _ _ _ _ _ _ _ _ _ _ _ _ _]
            tunnel: [_ _ _ _ _ _ _ _ _ _ _ _ _ _ _ _ _ _ _ _ _ _ _ _ _ _ _ _ _ _ _ _ _ _ _ _ _ _ _ _ _ _ _ _ _ _ _ _ _ TRUE _ _ _ _ _ _ _ _ _ _ _ _] -> w1033
            tunnel: w1022 -> [w1073 w1093 w1112 w1131 w1193 w1235 w1283 w1335 w1364 _ w1439 w1463 w1483 w1521 w1548 w1573 w1598 w1624 w1662 w1686 w1717 w1738 w1757 w1776 w1795 w1839 w1872 w1898 w1927 w1948 w1967 w1986 w2005 w2038 w2086 w2105 w2137 w2174 w2202 w2225 w2255 w2275 w2296 w2326 w2346 w2370 w2396 w2429 w2455 w2479 w2497 w2524 w2542 w2563 w2584 w2605 w2629 w2656 w2676 w2704 w2723 w2749]
            tunnel: w1021 -> [w1072 w1092 w1111 w1130 w1192 w1234 w1282 w1334 w1365 _ w1438 w1462 w1482 w1520 w1547 w1572 w1597 w1623 w1661 w1685 w1716 w1737 w1756 w1775 w1794 w1838 w1871 w1897 w1926 w1947 w1966 w1985 w2004 w2037 w2085 w2104 w2136 w2173 w2201 w2224 w2254 w2274 w2295 w2325 w2345 w2369 w2395 w2428 w2454 w2478 w2496 w2523 w2541 w2562 w2583 w2604 w2628 w2655 w2675 w2703 w2722 w2748]
            tunnel: w1020 -> [w1071 w1091 w1110 w1129 w1191 w1233 w1281 w1333 w1366 _ w1437 w1461 w1481 w1519 w1546 w1571 w1596 w1622 w1660 w1684 w1715 w1736 w1755 w1774 w1793 w1837 w1870 w1896 w1925 w1946 w1965 w1984 w2003 w2036 w2084 w2103 w2135 w2172 w2200 w2223 w2253 w2273 w2294 w2324 w2344 w2368 w2394 w2427 w2453 w2477 w2495 w2522 w2540 w2561 w2582 w2603 w2627 w2654 w2674 w2702 w2721 w2747]
            tunnel: w1019 -> [w1070 w1090 w1109 w1128 w1190 w1232 w1280 w1332 w1367 _ w1436 w1460 w1480 w1518 w1545 w1570 w1595 w1621 w1659 w1683 w1714 w1735 w1754 w1773 w1792 w1836 w1869 w1895 w1924 w1945 w1964 w1983 w2002 w2035 w2083 w2102 w2134 w2171 w2199 w2222 w2252 w2272 w2293 w2323 w2343 w2367 w2393 w2426 w2452 w2476 w2494 w2521 w2539 w2560 w2581 w2602 w2626 w2653 w2673 w2701 w2720 w2746]
            tunnel: w1018 -> [_ _ _ _ _ _ _ _ _ _ _ _ _ _ _ _ _ _ _ _ _ _ _ _ _ _ w1874 _ _ _ _ _ _ _ _ _ _ _ _ _ _ _ _ _ _ _ _ _ _ _ _ _ _ _ _ _ _ _ _ _ _ _]
            tunnel: w1017 -> [_ _ _ _ _ _ _ _ _ _ _ _ _ _ _ _ _ _ _ _ _ _ _ _ _ _ w1873 _ _ _ _ _ _ _ _ _ _ _ _ _ _ _ _ _ _ _ _ _ _ _ _ _ _ _ _ _ _ _ _ _ _ _]
            tunnel: [w1073 w1093 w1112 w1131 w1193 w1235 w1283 w1335 w1364 w1411 w1439 w1463 w1483 w1521 w1548 w1573 w1598 w1624 w1662 w1686 w1717 w1738 w1757 w1776 w1795 w1839 w1872 w1898 w1927 w1948 w1967 w1986 w2005 w2038 w2086 w2105 w2137 w2174 w2202 w2225 w2255 w2275 w2296 w2326 w2346 w2370 w2396 w2429 w2455 w2479 w2497 w2524 w2542 w2563 w2584 w2605 w2629 w2656 w2676 w2704 w2723 w2749] -> w1014
            tunnel: [w1072 w1092 w1111 w1130 w1192 w1234 w1282 w1334 w1365 w1410 w1438 w1462 w1482 w1520 w1547 w1572 w1597 w1623 w1661 w1685 w1716 w1737 w1756 w1775 w1794 w1838 w1871 w1897 w1926 w1947 w1966 w1985 w2004 w2037 w2085 w2104 w2136 w2173 w2201 w2224 w2254 w2274 w2295 w2325 w2345 w2369 w2395 w2428 w2454 w2478 w2496 w2523 w2541 w2562 w2583 w2604 w2628 w2655 w2675 w2703 w2722 w2748] -> w982
            tunnel: [w1071 w1091 w1110 w1129 w1191 w1233 w1281 w1333 w1366 w1409 w1437 w1461 w1481 w1519 w1546 w1571 w1596 w1622 w1660 w1684 w1715 w1736 w1755 w1774 w1793 w1837 w1870 w1896 w1925 w1946 w1965 w1984 w2003 w2036 w2084 w2103 w2135 w2172 w2200 w2223 w2253 w2273 w2294 w2324 w2344 w2368 w2394 w2427 w2453 w2477 w2495 w2522 w2540 w2561 w2582 w2603 w2627 w2654 w2674 w2702 w2721 w2747] -> w1015
            tunnel: [w1070 w1090 w1109 w1128 w1190 w1232 w1280 w1332 w1367 w1408 w1436 w1460 w1480 w1518 w1545 w1570 w1595 w1621 w1659 w1683 w1714 w1735 w1754 w1773 w1792 w1836 w1869 w1895 w1924 w1945 w1964 w1983 w2002 w2035 w2083 w2102 w2134 w2171 w2199 w2222 w2252 w2272 w2293 w2323 w2343 w2367 w2393 w2426 w2452 w2476 w2494 w2521 w2539 w2560 w2581 w2602 w2626 w2653 w2673 w2701 w2720 w2746] -> w1016
            tunnel: [_ _ _ _ _ _ _ _ _ _ _ _ _ _ _ _ _ _ _ _ _ _ _ _ _ w1826 w1874 _ _ _ _ _ _ _ _ _ _ _ _ _ _ _ _ _ _ _ _ _ _ _ _ _ _ _ _ _ _ _ _ _ _ _] -> w984
            tunnel: [_ _ _ _ _ _ _ _ _ _ _ _ _ _ _ _ _ _ _ _ _ _ _ _ _ w1825 w1873 _ _ _ _ _ _ _ _ _ _ _ _ _ _ _ _ _ _ _ _ _ _ _ _ _ _ _ _ _ _ _ _ _ _ _] -> w983
            tunnel: w997 -> [w1069 w1089 w1108 w1127 w1189 w1231 w1279 w1331 w1363 w1407 w1435 w1459 w1479 w1504 w1537 w1556 w1583 w1620 w1658 w1682 w1713 w1734 w1753 w1772 w1791 w1824 w1868 w1894 w1923 w1944 w1963 w1982 w2001 w2034 w2082 w2099 w2133 w2170 w2198 w2219 w2246 w2271 w2290 w2317 w2342 w2361 w2389 w2419 w2450 w2475 w2507 w2532 w2543 w2564 w2585 w2606 w2630 w2657 w2677 w2705 w2724 w2740]
            tunnel: [w1069 w1089 w1108 w1127 w1189 w1231 w1279 w1331 w1363 w1407 w1435 w1459 w1479 w1503 w1536 w1555 w1582 w1620 w1658 w1682 w1713 w1734 w1753 w1772 w1791 w1824 w1868 w1894 w1923 w1944 w1963 w1982 w2001 w2034 w2082 w2099 w2133 w2170 w2198 w2219 w2246 w2271 w2290 w2317 w2342 w2361 w2388 w2419 w2450 w2475 w2507 w2532 w2543 w2564 w2585 w2606 w2630 w2657 w2677 w2705 w2724 w2740] -> w996
            tunnel: [w1068 w1088 w1107 w1126 w1188 w1230 w1278 w1330 w1362 w1406 w1434 w1470 w1478 w1524 w1544 w1569 w1594 w1619 w1657 w1681 w1712 w1733 w1752 w1771 w1790 w1823 w1867 w1893 w1922 w1943 w1962 w1981 w2000 w2033 w2081 w2098 w2132 w2169 w2197 w2218 w2245 w2270 w2289 w2316 w2341 w2360 w2381 w2425 w2449 w2473 w2508 w2518 w2538 w2559 w2580 w2601 w2625 w2661 w2681 w2708 w2728 w2753] -> w995
            tunnel: [w1067 w1087 w1106 w1125 w1187 w1229 w1277 w1329 w1361 w1405 w1433 w1469 w1477 w1523 w1543 w1568 w1593 w1618 w1656 w1680 w1711 w1732 w1751 w1770 w1789 w1822 w1866 w1892 w1921 w1942 w1961 w1980 w1999 w2032 w2080 w2097 w2131 w2168 w2196 w2217 w2244 w2269 w2288 w2315 w2340 w2359 w2380 w2424 w2448 w2474 w2490 w2515 w2548 w2569 w2590 w2611 w2633 w2660 w2680 w2707 w2727 w2752] -> w994
            tunnel: w993 -> [w1068 w1088 w1107 w1126 w1188 w1230 w1278 w1330 w1362 w1406 w1434 w1470 w1478 w1524 w1544 w1569 w1594 w1619 w1657 w1681 w1712 w1733 w1752 w1771 w1790 w1823 w1867 w1893 w1922 w1943 w1962 w1981 w2000 w2033 w2081 w2098 w2132 w2169 w2197 w2218 w2245 w2270 w2289 w2316 w2341 w2360 w2381 w2425 w2449 w2473 _ w2518 w2538 w2559 w2580 w2601 w2625 w2661 w2681 w2708 w2728 w2753]
            tunnel: w992 -> [w1067 w1087 w1106 w1125 w1187 w1229 w1277 w1329 w1361 w1405 w1433 w1469 w1477 w1523 w1543 w1568 w1593 w1618 w1656 w1680 w1711 w1732 w1751 w1770 w1789 w1822 w1866 w1892 w1921 w1942 w1961 w1980 w1999 w2032 w2080 w2097 w2131 w2168 w2196 w2217 w2244 w2269 w2288 w2315 w2340 w2359 w2380 w2424 w2448 w2474 _ w2515 w2548 w2569 w2590 w2611 w2633 w2660 w2680 w2707 w2727 w2752]
            tunnel: w991 -> [_ _ _ _ _ _ _ _ _ _ _ _ _ _ _ _ _ _ _ _ _ _ _ _ _ _ _ _ _ _ _ _ _ _ _ _ _ _ _ _ _ _ _ _ _ _ _ _ _ _ _ _ w2536 w2557 w2578 w2599 w2623 _ _ _ _ _]
            tunnel: w989 -> [_ _ _ _ _ _ _ _ _ _ _ _ _ _ _ _ w1578 w1607 w1642 w1674 w1703 _ _ _ _ _ _ _ _ _ _ _ _ _ _ _ _ _ _ _ _ _ _ _ _ _ _ _ _ _ _ _ _ _ _ _ _ _ _ _ _ _]
            tunnel: [_ "A6" _ _ _ _ _ _ _ _ _ _ _ _ _ _ _ _ _ _ _ _ _ _ _ _ _ _ _ _ _ _ _ _ _ _ _ _ _ _ _ _ _ _ _ _ _ _ _ _ _ _ _ _ _ _ _ _ _ _ _ _] -> w972
            tunnel: w986 -> [_ _ _ _ _ _ _ _ _ _ _ _ _ _ _ _ _ _ _ _ _ _ _ _ _ _ _ _ _ _ _ _ _ _ _ _ _ _ _ _ _ _ _ _ _ _ _ _ _ _ _ _ _ _ _ _ _ _ _ w2695 _ _]
            tunnel: [w1066 w1085 w1105 w1124 w1186 w1228 w1276 w1328 w1360 w1404 w1428 w1453 w1473 w1525 w1542 w1567 w1592 w1617 w1655 w1679 w1710 w1731 w1750 w1769 w1788 w1821 w1865 w1891 w1920 w1941 w1960 w1979 w1998 w2028 w2079 w2096 w2130 w2153 w2195 w2216 w2243 w2268 w2287 w2314 w2339 w2358 w2379 w2422 w2435 w2472 w2493 w2517 w2535 w2556 w2577 w2598 w2620 w2640 w2669 w2689 w2716 w2736] -> w980
            tunnel: w981 -> [w1066 w1085 w1105 w1124 w1186 w1228 w1276 w1328 w1360 w1404 w1428 _ w1473 w1525 w1542 w1567 w1592 w1617 w1655 w1679 w1710 w1731 w1750 w1769 w1788 w1821 w1865 w1891 w1920 w1941 w1960 w1979 w1998 w2028 w2079 w2096 w2130 w2153 w2195 w2216 w2243 w2268 w2287 w2314 w2339 w2358 w2379 w2422 w2436 w2472 w2493 w2517 w2535 w2556 w2577 w2598 w2620 w2640 w2669 w2689 w2716 w2736]
            tunnel: w979 -> [w1065 w1084 w1104 w1123 w1185 w1227 w1275 w1327 w1359 w1403 w1427 w1452 w1472 w1517 w1541 w1566 w1591 w1616 w1654 w1678 w1709 w1730 w1749 w1768 w1787 w1820 w1864 w1890 w1919 w1940 w1959 w1978 w1997 w2027 w2078 w2095 w2129 w2167 w2194 w2215 w2242 w2267 w2286 w2313 w2338 w2357 w2378 w2421 w2447 w2471 w2492 w2520 w2534 w2555 w2576 w2597 w2619 w2639 w2668 w2688 w2715 w2735]
            tunnel: w978 -> [w1064 w1083 w1103 w1122 w1184 w1226 w1274 w1326 w1358 w1402 w1426 w1451 w1471 w1516 w1540 w1565 w1590 w1615 w1653 w1677 w1708 w1729 w1748 w1767 w1786 w1819 w1863 w1889 w1918 w1939 w1958 w1977 w1996 w2026 w2077 w2094 w2128 w2164 w2193 w2214 w2241 w2266 w2285 w2312 w2337 w2356 w2377 w2420 w2446 w2470 w2491 w2519 w2533 w2554 w2575 w2596 w2618 w2638 w2667 w2687 w2714 w2734]
            tunnel: [w1065 w1084 w1104 w1123 w1185 w1227 w1275 w1327 w1359 w1403 w1427 w1452 w1472 w1517 w1541 w1566 w1591 w1616 w1654 w1678 w1709 w1730 w1749 w1768 w1787 w1820 w1864 w1890 w1919 w1940 w1959 w1978 w1997 w2027 w2078 w2095 w2129 w2166 w2194 w2215 w2242 w2267 w2286 w2313 w2338 w2357 w2378 w2421 w2447 w2471 w2492 w2520 w2534 w2555 w2576 w2597 w2619 w2639 w2668 w2688 w2715 w2735] -> w977
            tunnel: [w1064 w1083 w1103 w1122 w1184 w1226 w1274 w1326 w1358 w1402 w1426 w1451 w1471 w1516 w1540 w1565 w1590 w1615 w1653 w1677 w1708 w1729 w1748 w1767 w1786 w1819 w1863 w1889 w1918 w1939 w1958 w1977 w1996 w2026 w2077 w2094 w2128 w2165 w2193 w2214 w2241 w2266 w2285 w2312 w2337 w2356 w2377 w2420 w2446 w2470 w2491 w2519 w2533 w2554 w2575 w2596 w2618 w2638 w2667 w2687 w2714 w2734] -> w976
            tunnel: w975 -> [_ _ _ _ _ _ _ _ _ _ _ _ _ w1528 _ _ _ _ _ _ _ _ _ _ _ _ w1860 _ _ _ _ _ _ w2024 w2076 _ _ _ _ _ _ _ _ _ _ _ _ _ _ _ _ _ _ _ _ _ _ _ _ _ _ _]
            tunnel: w974 -> [_ _ _ _ _ _ _ _ _ _ _ _ _ w1527 _ _ _ _ _ _ _ _ _ _ _ _ w1859 _ _ _ _ _ _ w2025 w2075 _ _ _ _ _ _ _ _ _ _ _ _ _ _ _ _ _ _ _ _ _ _ _ _ _ _ _]
            tunnel: w971 -> [_ _ _ _ _ _ _ _ _ _ _ _ _ _ _ _ w1577 w1606 w1641 w1672 w1704 _ _ _ _ _ _ _ _ _ _ _ _ _ _ _ _ _ _ _ _ _ _ _ _ _ _ _ _ _ _ _ _ _ _ _ _ _ _ _ _ _]
            tunnel: [_ _ _ _ _ _ _ _ _ _ _ _ _ _ _ _ _ w1610 w1643 w1673 w1707 _ _ _ _ TRUE w1848 w1882 w1916 _ _ _ _ _ _ _ _ _ _ _ _ _ _ _ _ _ _ _ _ _ _ _ _ _ _ _ _ _ _ _ _ _] -> w970
            tunnel: w969 -> [_ _ _ _ _ _ _ _ _ _ _ _ _ _ _ _ _ w1609 w1648 w1676 w1705 _ _ _ _ w1811 w1854 w1887 w1915 _ _ _ _ _ _ _ _ _ _ _ _ _ _ _ _ _ _ _ _ _ _ _ _ _ _ _ _ _ _ _ _ _]
            tunnel: w968 -> [_ _ _ _ _ _ _ _ _ _ _ _ _ _ _ _ _ w1608 w1647 w1675 w1706 _ _ _ _ w1810 w1853 w1886 w1914 _ _ _ _ _ _ _ _ _ _ _ _ _ _ _ _ _ _ _ _ _ _ _ _ _ _ _ _ _ _ _ _ _]
            tunnel: [_ _ _ _ _ _ _ _ _ _ _ _ _ _ _ _ w1580 w1609 w1648 w1676 w1705 _ _ _ _ w1811 w1854 w1884 w1915 _ _ _ _ _ _ _ _ _ _ _ _ _ _ _ _ _ _ _ _ _ _ _ _ _ _ _ _ _ _ _ _ _] -> w967
            tunnel: [_ _ _ _ _ _ _ _ _ _ _ _ _ _ _ _ w1579 w1608 w1647 w1675 w1706 _ _ _ _ w1810 w1853 w1885 w1914 _ _ _ _ _ _ _ _ _ _ _ _ _ _ _ _ _ _ _ _ _ _ _ _ _ _ _ _ _ _ _ _ _] -> w966
            tunnel: [_ _ _ _ _ _ _ _ _ _ _ _ _ _ _ w1559 w1578 w1607 w1642 w1669 w1703 _ _ _ _ _ _ _ _ _ _ _ _ _ _ _ _ _ _ _ _ _ _ _ _ _ _ _ _ _ _ _ _ _ _ _ _ _ _ _ _ _] -> w965
            tunnel: [_ _ _ _ _ _ _ _ _ _ _ _ _ _ _ w1560 w1577 w1606 w1641 w1670 w1704 _ _ _ _ _ _ _ _ _ _ _ _ _ _ _ _ _ _ _ _ _ _ _ _ _ _ _ _ _ _ _ _ _ _ _ _ _ _ _ _ _] -> w964
            tunnel: [_ _ _ _ _ _ _ _ _ _ _ _ _ _ _ _ _ _ w1640 _ _ _ _ _ _ _ w1851 _ _ _ _ _ _ _ _ _ _ _ _ _ _ _ _ _ _ _ _ _ _ _ _ _ _ _ _ _ _ _ _ _ _ _] -> w961
            tunnel: [_ _ _ _ _ _ _ _ _ _ _ _ _ _ _ _ _ _ w1639 _ _ _ _ _ _ _ w1852 _ _ _ _ _ _ _ _ _ _ _ _ _ _ _ _ _ _ _ _ _ _ _ _ _ _ _ _ _ _ _ _ _ _ _] -> w963
            tunnel: w958 -> [_ _ _ _ _ _ _ _ _ _ _ _ _ _ _ _ _ w1605 w1638 w1668 w1702 _ _ _ _ w1806 w1850 w1883 w1917 _ _ _ _ _ _ _ _ _ _ _ _ _ _ _ _ _ _ _ _ _ _ _ _ _ _ _ _ _ _ _ _ _]
            tunnel: [_ _ _ _ _ _ _ _ _ _ _ _ _ _ _ _ _ w1605 w1638 w1668 w1702 _ _ _ _ w1806 w1849 w1883 w1917 _ _ _ _ _ _ _ _ _ _ _ _ _ _ _ _ _ _ _ _ _ _ _ _ _ _ _ _ _ _ _ _ _] -> w957
            frame "Start1", Default {
            }
            frame "Start2" {
            }
            frame "Start3" {
            }
            frame "saveSettings1" {
              n526 = call "myRIO_BRig_RT_dataExp_Audio_freq__L.vi"() -> ("output_Audio_freq__L"=w1151:i32)  [unwired: 11 in]
              n527 = call "myRIO_BRig_RT_dataExp_Audio_freq__R.vi"() -> ("output_Audio_freq__R"=w1148:i32)  [unwired: 11 in]
              n528 = call "myRIO_BRig_RT_dataExp_Audio_amp__L.vi"() -> ("output_Audio_amp__L"=w1145:i32)  [unwired: 11 in]
              n529 = call "myRIO_BRig_RT_dataExp_Audio_amp__R.vi"() -> ("output_Audio_amp__R"=w1143:i32)  [unwired: 11 in]
              n530 = call "myRIO_BRig_RT_dataExp_TPB_min__L.vi"() -> ("output_TPB_min__L"=w1161:i32)  [unwired: 11 in]
              n531 = call "myRIO_BRig_RT_dataExp_TPB_min__R.vi"() -> ("output_TPB_min__R"=w1159:i32)  [unwired: 11 in]
              n532 = call "myRIO_BRig_RT_dataExp_TPB_max__L.vi"() -> ("output_TPB_max__L"=w1157:i32)  [unwired: 11 in]
              n533 = call "myRIO_BRig_RT_dataExp_TPB_max__R.vi"() -> ("output_TPB_max__R"=w1155:i32)  [unwired: 11 in]
              n534 = call "myRIO_BRig_RT_dataExp_ItrialUntilReward.vi"() -> ("output_I_trialUntilReward"=w1174:i32)  [unwired: 11 in]
              n535 = call "myRIO_BRig_RT_dataExp_IblockUntilReward.vi"() -> ("output_I_blockUntilReward"=w1170:i32)  [unwired: 11 in]
              n536 = call "myRIO_BRig_RT_dataExp_CueCycles.vi"() -> ("output_CueCycles"=w1169:i32)  [unwired: 11 in]
              n537 = call "myRIO_BRig_RT_dataExp_ENL_min.vi"() -> ("output_ENL_min"=w1167:i32)  [unwired: 11 in]
              n538 = call "myRIO_BRig_RT_dataExp_ENL_max.vi"() -> ("output_ENL_max"=w1165:i32)  [unwired: 11 in]
              n539 = call "myRIO_BRig_RT_dataExp_ENL_penalty.vi"() -> ("output_ENL_penalty"=w1163:i32)  [unwired: 11 in]
              n540 = local read "Audio_Freq__L"() -> (w1152:u16)
              n541 = local read "Audio_Freq__R"() -> (w1147:u16)
              n542 = local read "Audio_Amp__L"() -> (w1144:u16)
              n543 = local read "TpB_Min_L"() -> (w1160:u16)
              n544 = local read "TpB_Min_R"() -> (w1158:u16)
              n545 = local read "TpB_Max_L"() -> (w1156:u16)
              n546 = local read "TpB_Max_R"() -> (w1154:u16)
              n547 = local read "Audio_Amp__R"() -> (w1142:u16)
              n548 = local read "TrialUntilReward"() -> (w1173:bool)
              n549 = local read "CueCycles"() -> (w1168:u16)
              n550 = local read "Tcycle_ENL_min"() -> (w1166:u16)
              n551 = local read "Tcycle_ENL_max"() -> (w1164:u16)
              n552 = local read "Tcycle_ENLPenalty"() -> (w1162:u16)
              n553 = Multiply(x=w1152, y=u16 1000) -> (x*y=w1150:u16)
              n554 = Multiply(x=w1147, y=u16 1000) -> (x*y=w1146:u16)
              n555 = Boolean To (0,1)(Boolean=w1173) -> (0, 1=w1172:i16)
              n556 = To Unsigned Word Integer(number=w1172) -> (unsigned 16bit integer=w1171:u16)
              n557 = local read "BUR_min"() -> (w1136:u16)
              n558 = local read "BUR_max"() -> (w1137:u16)
              n559 = Not Equal To 0?(x=w1136) -> (x != 0?=w1135:bool)
              n560 = Not Equal To 0?(x=w1137) -> (x != 0?=w1134:bool)
              n561 = And(x=w1135, y=w1134) -> (x .and. y?=w1133:bool)
              n562 = Boolean To (0,1)(Boolean=w1133) -> (0, 1=w1138:i16)
              n563 = To Unsigned Word Integer(number=w1138) -> (unsigned 16bit integer=w1132:u16)
              n564 = Replace Array Subset(array=w1176, new element #1=w1171, index #1=w1174, new element #2=w1132, index #2=w1170, new element #3=w1168, index #3=w1169, new element #4=w1166, index #4=w1167, new element #5=w1164, index #5=w1165, new element #6=w1162, index #6=w1163, new element #7=w1160, index #7=w1161, new element #8=w1158, index #8=w1159, new element #9=w1156, index #9=w1157, new element #10=w1154, index #10=w1155, new element #11=w1150, index #11=w1151, new element #12=w1146, index #12=w1148, new element #13=w1144, index #13=w1145, new element #14=w1142, index #14=w1143) -> (w1175:u16[])
            }
            frame "saveSettings2" {
              n565 = call "myRIO_BRig_RT_dataExp_Tcycle_RewardPost.vi"() -> ("output_Tcycle_RewardPost"=w1209:i32)  [unwired: 11 in]
              n566 = call "myRIO_BRig_RT_dataExp_Tcycle_Wrong.vi"() -> ("output_Tcycle_Wrong"=w1207:i32)  [unwired: 11 in]
              n567 = call "myRIO_BRig_RT_dataExp_Tcycle_Timeout.vi"() -> ("output_Tcycle_Timeout"=w1205:i32)  [unwired: 11 in]
              n568 = call "myRIO_BRig_RT_dataExp_Tcycle_Cue_min.vi"() -> ("output_Tcycle_Cue_min"=w1203:i32)  [unwired: 11 in]
              n569 = call "myRIO_BRig_RT_dataExp_Tcycle_Cue_max.vi"() -> ("output_Tcycle_Cue_max"=w1202:i32)  [unwired: 11 in]
              n570 = call "myRIO_BRig_RT_dataExp_Tcycle_CuePenalty.vi"() -> ("output_Tcycle_CuePenalty"=w1201:i32)  [unwired: 11 in]
              n571 = call "myRIO_BRig_RT_dataExp_nBlock.vi"() -> ("output_nBlock"=w1218:i32)  [unwired: 11 in]
              n572 = call "myRIO_BRig_RT_dataExp_nTrial.vi"() -> ("output_nTrial"=w1217:i32)  [unwired: 11 in]
              n573 = call "myRIO_BRig_RT_dataExp_runTime_seconds.vi"() -> ("output_RunTime_minutes"=w1216:i32)  [unwired: 11 in]
              n574 = call "myRIO_BRig_RT_dataExp_Tcycle_Selection.vi"() -> ("output_Tcycle_Selection"=w1215:i32)  [unwired: 11 in]
              n575 = call "myRIO_BRig_RT_dataExp_Tcycle_Reward__L.vi"() -> ("output_Tcycle_Reward__L"=w1213:i32)  [unwired: 11 in]
              n576 = call "myRIO_BRig_RT_dataExp_Tcycle_Reward__R.vi"() -> ("output_Tcycle_Reward__R"=w1211:i32)  [unwired: 11 in]
              n577 = local read "Tcycle_RewardPost"() -> (w1208:u16)
              n578 = local read "Tcycle_Wrong"() -> (w1206:u16)
              n579 = local read "Tcycle_Timeout"() -> (w1204:u16)
              n580 = local read "Tcycle_CuePenalty"() -> (w1194:u16)
              n581 = local read "Tcycle_Cue_max"() -> (w1182:u16)
              n582 = local read "Tcycle_Cue_min"() -> (w1183:u16)
              n583 = local read "Tcycle_Selection"() -> (w1214:u16)
              n584 = local read "Tcycle_Reward_L"() -> (w1212:u16)
              n585 = local read "Tcycle_Reward_R"() -> (w1210:u16)
              n586 = Replace Array Subset(array=w1220, new element #1=u16 0, index #1=w1218, new element #2=u16 0, index #2=w1217, new element #3=u16 0, index #3=w1216, new element #4=w1214, index #4=w1215, new element #5=w1212, index #5=w1213, new element #6=w1210, index #6=w1211, new element #7=w1208, index #7=w1209, new element #8=w1206, index #8=w1207, new element #9=w1204, index #9=w1205, new element #10=w1183, index #10=w1203, new element #11=w1182, index #11=w1202, new element #12=w1194, index #12=w1201) -> (w1219:u16[])
            }
            frame "saveSettings3" {
              n587 = call "myRIO_BRig_RT_dataExp_BUR_min.vi"() -> ("output_BUR_min"=w1244:i32)  [unwired: 11 in]
              n588 = call "myRIO_BRig_RT_dataExp_BUR_max.vi"() -> ("output_BUR_max"=w1242:i32)  [unwired: 11 in]
              n589 = call "myRIO_BRig_RT_dataExp_Audio_sp__L.vi"() -> ("output_Audio_sp__L"=w1239:i32)  [unwired: 11 in]
              n590 = call "myRIO_BRig_RT_dataExp_Audio_sp__R.vi"() -> ("output_Audio_sp__R"=w1238:i32)  [unwired: 11 in]
              n591 = local read "sp_LeftSpout"() -> (w1237:u16)
              n592 = local read "BUR_max"() -> (w1241:u16)
              n593 = local read "sp_RightSpout"() -> (w1236:u16)
              n594 = local read "BUR_min"() -> (w1243:u16)
              n595 = Replace Array Subset(array=w1245, new element #1=w1243, index #1=w1244, new element #2=w1241, index #2=w1242, new element #3=w1237, index #3=w1239, new element #4=w1236, index #4=w1238) -> (w1240:u16[])
            }
            frame "saveSettings4_LC_ENL" {
              # "delayOpt"
              # "Count"
              # "Tdelay"
              # "Probability"
              # "OnOff"
              # "Block"
              # "ENL1 All"
              # "delayOpt"
              # "Count"
              # "Tdelay"
              # "Probability"
              # "OnOff"
              # "Block"
              # "ENL1 First"
              n596 = call "myRIO_BRig_RT_dataLC_ENL1_All_Block.vi"() -> ("output_ENL1_All_Block"=w1269:i32)  [unwired: 11 in]
              n597 = call "myRIO_BRig_RT_dataLC_ENL1_All_OnOff.vi"() -> ("output_ENL1_All_OnOff"=w1258:i32)  [unwired: 11 in]
              n598 = call "myRIO_BRig_RT_dataLC_ENL1_All_Probability.vi"() -> ("output_ENL1_All_Probability"=w1257:i32)  [unwired: 11 in]
              n599 = call "myRIO_BRig_RT_dataLC_ENL1_All_Tdelay.vi"() -> ("output_ENL1_All_Tdelay"=w1256:i32)  [unwired: 11 in]
              n600 = call "myRIO_BRig_RT_dataLC_ENL1_All_Count.vi"() -> ("output_ENL1_All_Count"=w1255:i32)  [unwired: 11 in]
              n601 = call "myRIO_BRig_RT_dataLC_ENL1_All_delayOpt.vi"() -> ("output_ENL1_All_delayOpt"=w1254:i32)  [unwired: 11 in]
              n602 = call "myRIO_BRig_RT_dataLC_ENL1_First_Block.vi"() -> ("output_ENL1_First_Block"=w1295:i32)  [unwired: 11 in]
              n603 = call "myRIO_BRig_RT_dataLC_ENL1_First_OnOff.vi"() -> ("output_ENL1_First_OnOff"=w1293:i32)  [unwired: 11 in]
              n604 = call "myRIO_BRig_RT_dataLC_ENL1_First_Probability.vi"() -> ("output_ENL1_First_Probability"=w1289:i32)  [unwired: 11 in]
              n605 = call "myRIO_BRig_RT_dataLC_ENL1_First_Tdelay.vi"() -> ("output_ENL1_First_Tdelay"=w1287:i32)  [unwired: 11 in]
              n606 = call "myRIO_BRig_RT_dataLC_ENL1_First_Count.vi"() -> ("output_ENL1_First_Count"=w1285:i32)  [unwired: 11 in]
              n607 = call "myRIO_BRig_RT_dataLC_ENL1_First_delayOpt.vi"() -> ("output_ENL1_First_delayOpt"=w1271:i32)  [unwired: 11 in]
              n608 = local read "LC_ENL1_First_delayOpt"() -> (w1272:bool)
              n609 = local read "LC_ENL1_First_Count"() -> (w1284:u16)
              n610 = local read "LC_ENL1_First_Probability"() -> (w1288:u16)
              n611 = local read "LC_ENL1_First_Block"() -> (w1294:u16)
              n612 = local read "LC_ENL1_First_Tdelay"() -> (w1286:u16)
              n613 = local read "LC_ENL1_First_OnOff"() -> (w1292:bool)
              n614 = local read "LC_ENL1_All_OnOff"() -> (w1265:bool)
              n615 = local read "LC_ENL1_All_Probability"() -> (w1263:u16)
              n616 = local read "LC_ENL1_All_delayOpt"() -> (w1260:bool)
              n617 = local read "LC_ENL1_All_Tdelay"() -> (w1262:u16)
              n618 = local read "LC_ENL1_All_Block"() -> (w1266:u16)
              n619 = local read "LC_ENL1_All_Count"() -> (w1261:u16)
              n620 = Boolean To (0,1)(Boolean=w1272) -> (0, 1=w1273:i16)
              n621 = Boolean To (0,1)(Boolean=w1292) -> (0, 1=w1291:i16)
              n622 = Boolean To (0,1)(Boolean=w1265) -> (0, 1=w1268:i16)
              n623 = To Unsigned Word Integer(number=w1273) -> (unsigned 16bit integer=w1270:u16)
              n624 = To Unsigned Word Integer(number=w1291) -> (unsigned 16bit integer=w1290:u16)
              n625 = Boolean To (0,1)(Boolean=w1260) -> (0, 1=w1267:i16)
              n626 = To Unsigned Word Integer(number=w1268) -> (unsigned 16bit integer=w1264:u16)
              n627 = To Unsigned Word Integer(number=w1267) -> (unsigned 16bit integer=w1259:u16)
              n628 = Replace Array Subset(array=w1296, new element #1=w1294, index #1=w1295, new element #2=w1290, index #2=w1293, new element #3=w1288, index #3=w1289, new element #4=w1286, index #4=w1287, new element #5=w1284, index #5=w1285, new element #6=w1270, index #6=w1271, new element #7=w1266, index #7=w1269, new element #8=w1264, index #8=w1258, new element #9=w1263, index #9=w1257, new element #10=w1262, index #10=w1256, new element #11=w1261, index #11=w1255, new element #12=w1259, index #12=w1254) -> (w1297:u16[])
            }
            frame "saveSettings5_LC_Cue" {
              # "delayOpt"
              # "Count"
              # "Tdelay"
              # "Probability"
              # "OnOff"
              # "Block"
              # "Cue1 All"
              # "delayOpt"
              # "Count"
              # "Tdelay"
              # "Probability"
              # "OnOff"
              # "Block"
              # "Cue1 First"
              n629 = call "myRIO_BRig_RT_dataLC_Cue1_First_delayOpt.vi"() -> ("output_Cue1_First_delayOpt"=w1324:i32)  [unwired: 11 in]
              n630 = call "myRIO_BRig_RT_dataLC_Cue1_First_Block.vi"() -> ("output_Cue1_First_Block"=w1347:i32)  [unwired: 11 in]
              n631 = call "myRIO_BRig_RT_dataLC_Cue1_First_OnOff.vi"() -> ("output_Cue1_First_OnOff"=w1345:i32)  [unwired: 11 in]
              n632 = call "myRIO_BRig_RT_dataLC_Cue1_First_Probability.vi"() -> ("output_Cue1_First_Probability"=w1341:i32)  [unwired: 11 in]
              n633 = call "myRIO_BRig_RT_dataLC_Cue1_First_Tdelay.vi"() -> ("output_Cue1_First_Tdelay"=w1339:i32)  [unwired: 11 in]
              n634 = call "myRIO_BRig_RT_dataLC_Cue1_First_Count.vi"() -> ("output_Cue1_First_Count"=w1337:i32)  [unwired: 11 in]
              n635 = call "myRIO_BRig_RT_dataLC_Cue1_All_Block.vi"() -> ("output_Cue1_All_Block"=w1321:i32)  [unwired: 11 in]
              n636 = call "myRIO_BRig_RT_dataLC_Cue1_All_OnOff.vi"() -> ("output_Cue1_All_OnOff"=w1320:i32)  [unwired: 11 in]
              n637 = call "myRIO_BRig_RT_dataLC_Cue1_All_Probability.vi"() -> ("output_Cue1_All_Probability"=w1319:i32)  [unwired: 11 in]
              n638 = call "myRIO_BRig_RT_dataLC_Cue1_All_Tdelay.vi"() -> ("output_Cue1_All_Tdelay"=w1318:i32)  [unwired: 11 in]
              n639 = call "myRIO_BRig_RT_dataLC_Cue1_All_Count.vi"() -> ("output_Cue1_All_Count"=w1317:i32)  [unwired: 11 in]
              n640 = call "myRIO_BRig_RT_dataLC_Cue1_All_delayOpt.vi"() -> ("output_Cue1_All_delayOpt"=w1316:i32)  [unwired: 11 in]
              n641 = local read "LC_Cue1_First_delayOpt"() -> (w1323:bool)
              n642 = local read "LC_Cue1_First_Count"() -> (w1336:u16)
              n643 = local read "LC_Cue1_First_Probability"() -> (w1340:u16)
              n644 = local read "LC_Cue1_First_Block"() -> (w1346:u16)
              n645 = local read "LC_Cue1_First_Tdelay"() -> (w1338:u16)
              n646 = local read "LC_Cue1_First_OnOff"() -> (w1344:bool)
              n647 = local read "LC_Cue1_All_OnOff"() -> (w1312:bool)
              n648 = local read "LC_Cue1_All_delayOpt"() -> (w1313:bool)
              n649 = local read "LC_Cue1_All_Probability"() -> (w1309:u16)
              n650 = local read "LC_Cue1_All_Tdelay"() -> (w1308:u16)
              n651 = local read "LC_Cue1_All_Count"() -> (w1307:u16)
              n652 = local read "LC_Cue1_All_Block"() -> (w1311:u16)
              n653 = Boolean To (0,1)(Boolean=w1323) -> (0, 1=w1325:i16)
              n654 = Boolean To (0,1)(Boolean=w1344) -> (0, 1=w1343:i16)
              n655 = Boolean To (0,1)(Boolean=w1312) -> (0, 1=w1315:i16)
              n656 = To Unsigned Word Integer(number=w1325) -> (unsigned 16bit integer=w1322:u16)
              n657 = To Unsigned Word Integer(number=w1343) -> (unsigned 16bit integer=w1342:u16)
              n658 = To Unsigned Word Integer(number=w1315) -> (unsigned 16bit integer=w1310:u16)
              n659 = Boolean To (0,1)(Boolean=w1313) -> (0, 1=w1314:i16)
              n660 = To Unsigned Word Integer(number=w1314) -> (unsigned 16bit integer=w1306:u16)
              n661 = Replace Array Subset(array=w1348, new element #1=w1346, index #1=w1347, new element #2=w1342, index #2=w1345, new element #3=w1340, index #3=w1341, new element #4=w1338, index #4=w1339, new element #5=w1336, index #5=w1337, new element #6=w1322, index #6=w1324, new element #7=w1311, index #7=w1321, new element #8=w1310, index #8=w1320, new element #9=w1309, index #9=w1319, new element #10=w1308, index #10=w1318, new element #11=w1307, index #11=w1317, new element #12=w1306, index #12=w1316) -> (w1349:u16[])
            }
            frame "saveSettings6_LC_Other" {
              # "Trial"
              # "Tdelay"
              # "Probability"
              # "OnOff"
              # "Block"
              # "Wrong"
              # "Trial"
              # "Tdelay"
              # "Probability"
              # "OnOff"
              # "Block"
              # "Reward"
              n662 = call "myRIO_BRig_RT_dataLC_Wrong_Block.vi"() -> ("output_Wrong_Block"=w1379:i32)  [unwired: 11 in]
              n663 = call "myRIO_BRig_RT_dataLC_Wrong_OnOff.vi"() -> ("output_Wrong_OnOff"=w1378:i32)  [unwired: 11 in]
              n664 = call "myRIO_BRig_RT_dataLC_Wrong_Probability.vi"() -> ("output_Wrong_Probability"=w1377:i32)  [unwired: 11 in]
              n665 = call "myRIO_BRig_RT_dataLC_Wrong_Tdelay.vi"() -> ("output_Wrong_Tdelay"=w1376:i32)  [unwired: 11 in]
              n666 = call "myRIO_BRig_RT_dataLC_Wrong_Trial.vi"() -> ("output_Wrong_Trial"=w1375:i32)  [unwired: 11 in]
              n667 = call "myRIO_BRig_RT_dataLC_Reward_Block.vi"() -> ("output_Reward_Block"=w1391:i32)  [unwired: 11 in]
              n668 = call "myRIO_BRig_RT_dataLC_Reward_OnOff.vi"() -> ("output_Reward_OnOff"=w1389:i32)  [unwired: 11 in]
              n669 = call "myRIO_BRig_RT_dataLC_Reward_Probability.vi"() -> ("output_Reward_Probability"=w1385:i32)  [unwired: 11 in]
              n670 = call "myRIO_BRig_RT_dataLC_Reward_Tdelay.vi"() -> ("output_Reward_Tdelay"=w1383:i32)  [unwired: 11 in]
              n671 = call "myRIO_BRig_RT_dataLC_Reward_Trial.vi"() -> ("output_Reward_Trial"=w1381:i32)  [unwired: 11 in]
              n672 = local read "LC_Wrong_OnOff"() -> (w1373:bool)
              n673 = local read "LC_Wrong_Probability"() -> (w1370:u16)
              n674 = local read "LC_Wrong_Block"() -> (w1372:u16)
              n675 = local read "LC_Wrong_Tdelay"() -> (w1369:u16)
              n676 = local read "LC_Wrong_Trial"() -> (w1368:u16)
              n677 = local read "LC_Reward_Probability"() -> (w1384:u16)
              n678 = local read "LC_Reward_Block"() -> (w1390:u16)
              n679 = local read "LC_Reward_Tdelay"() -> (w1382:u16)
              n680 = local read "LC_Reward_OnOff"() -> (w1388:bool)
              n681 = local read "LC_Reward_Trial"() -> (w1380:u16)
              n682 = Boolean To (0,1)(Boolean=w1373) -> (0, 1=w1374:i16)
              n683 = Boolean To (0,1)(Boolean=w1388) -> (0, 1=w1387:i16)
              n684 = To Unsigned Word Integer(number=w1374) -> (unsigned 16bit integer=w1371:u16)
              n685 = To Unsigned Word Integer(number=w1387) -> (unsigned 16bit integer=w1386:u16)
              n686 = Replace Array Subset(array=w1392, new element #1=w1390, index #1=w1391, new element #2=w1386, index #2=w1389, new element #3=w1384, index #3=w1385, new element #4=w1382, index #4=w1383, new element #5=w1380, index #5=w1381, new element #6=w1372, index #6=w1379, new element #7=w1371, index #7=w1378, new element #8=w1370, index #8=w1377, new element #9=w1369, index #9=w1376, new element #10=w1368, index #10=w1375) -> (w1393:u16[])
            }
            frame "setSettings_Audio" {
              # "amp_L"
              # "amp_R"
              # "freq_L"
              # "freq_R"
              n687 = call "myRIO_BRig_RT_dataExp_Audio_amp__L.vi"() -> ("output_Audio_amp__L"=w1416:i32)  [unwired: 11 in]
              n688 = call "myRIO_BRig_RT_dataExp_Audio_amp__R.vi"() -> ("output_Audio_amp__R"=w1415:i32)  [unwired: 11 in]
              n689 = call "myRIO_BRig_RT_dataExp_Audio_freq__L.vi"() -> ("output_Audio_freq__L"=w1414:i32)  [unwired: 11 in]
              n690 = call "myRIO_BRig_RT_dataExp_Audio_freq__R.vi"() -> ("output_Audio_freq__R"=w1413:i32)  [unwired: 11 in]
              n691 = Index Array(array=w1412, index #1=w1416, index #2=w1415, index #3=w1414, index #4=w1413) -> (element #1=w1411:u16, element #2=w1409:u16, element #3=w1410:u16, element #4=w1408:u16)
            }
            frame "initBlock" {
              n692 = call "myRIO_Brig_RT__Case_Exp_State_initBlock.vi"("input_spout"=w1448, "input_dataExp"=w1446, "input_dataCurrent"=w1447) -> ("output_spout"=w1425:enum16{"Left", "Right"}, "output_state"=w1449:T2, "output_dataExp"=w1445:u16[], "output_dataCurrent"=w1431:u16[], "output_TpB_target"=→"TpB_target":u16)  [unwired: 4 in]
              "cSpout" <- w1425
              n693 = call "myRIO_BRig_RT_dataCurrent_iBlock.vi"() -> ("output_iBlock"=w1430:i32)  [unwired: 11 in]
              n694 = Index Array(array=w1431, index=w1430) -> (element=→"iBlock":u16)
            }
            frame "initBlock2" {
              n695 = local write "nRewards_cur"(u16 0 ("nRewards_cur")) -> ()
              n696 = call "myRIO_BRig_RT__Case_Exp_State_initBlock2.vi"("input_spout"=w1457, "input_dataBlock"=w1458, "input_dataCurrent"=w1456) -> ("idxDataBlock"=w1453:i32, "output_dataBlock"=w1455:u16[][])  [unwired: 7 in]
            }
            frame "initTrial" {
              n697 = call "myRIO_Brig_RT__Case_Exp_State_initTrial.vi"("input_dataExp"=w1487, "input_dataCurrent"=w1488) -> ("output_state"=w1489:T2, "output_dataExp"=w1486:u16[], "output_dataCurrent"=w1476:u16[])  [unwired: 7 in]
              n698 = call "myRIO_BRig_RT_dataCurrent_iTrial.vi"() -> ("output_iTrial"=w1475:i32)  [unwired: 11 in]
              n699 = Index Array(array=w1476, index=w1475) -> (element=→"iTrial":u16)
            }
            frame "initTrial2" {
              w1494 = u32 10
              # "laser time"
              # "Wrong tDelay"
              # "Reward tDelay"
              # "trialUntilReward"
              n700 = call "myRIO_BRig_RT__Case_Exp_subState_LC__initTrial.vi"("input_dataTrial"=w1504, "input_spout"=w1513, "input_dataCurrent"=w1502, "input_dataLC"=w1499) -> ("output_LC_Wrong"=w1514:bool, "output_LC_led_Wrong"=w1506:bool, "output_LC_Reward"=w1515:bool, "output_LC_led_Reward"=w1505:bool, "output_dataTrial"=w1503:u16[][])  [unwired: 2 in]
              n701 = Equal?(x=w1513, y=enum16{"Left", "Right"}."Right") -> (x = y?=w1511:bool)
              n702 = call "myRIO_BRig_RT_dataExp_ItrialUntilReward.vi"() -> ("output_I_trialUntilReward"=w1509:i32)  [unwired: 11 in]
              n703 = Index Array(array=w1510, index=w1509) -> (element=w1508:u16)
              n704 = call "myRIO_BRig_RT_dataLC_Reward_Tdelay.vi"() -> ("output_Reward_Tdelay"=w1500:i32)  [unwired: 11 in]
              n705 = call "myRIO_BRig_RT_dataLC_Wrong_Tdelay.vi"() -> ("output_Wrong_Tdelay"=w1501:i32)  [unwired: 11 in]
              n706 = Not Equal To 0?(x=w1508) -> (x != 0?=w1507:bool)
              n707 = Index Array(array=w1499, index #1=w1500, index #2=w1501) -> (element #1=w1498:u16, element #2=w1497:u16)
              n708 = To Unsigned Long Integer(number=w1498) -> (unsigned 32bit integer=w1496:u32)
              n709 = To Unsigned Long Integer(number=w1497) -> (unsigned 32bit integer=w1495:u32)
              n710 = xnode "Read/Write Control"("FPGA VI Reference In"=w1528, "error in"=w1527, "SelectionState"=FALSE, "laserResponse_reward"=w1515, "laserResponse_wrong"=w1514, "laserResponse_reward_LED"=w1505, "laserResponse_wrong_LED"=w1506, "Left(F)_or_Right(T)"=w1511, "ignoreWrong"=w1507, "tCycle_laser_rew"=w1494, "tDelay_laser_rew"=w1496, "tCycle_laser_wro"=w1494, "tDelay_laser_wro"=w1495) -> ("error out"=→"error_initTrial":errorcluster)  [unwired: 1 out]
            }
            frame "initTrial3" {
              n711 = call "myRIO_BRig_RT__Case_Exp_State_initTrial_dataTrial.vi"("input_spout"=w1534, "input_dataCurrent"=w1535, "input_dataTrial"=w1537) -> ("output_dataTrial"=w1536:u16[][])  [unwired: 8 in]
            }
            frame "initTrial_LC_ENL1" {
              n712 = call "myRIO_BRig_RT__Case_Exp_State_initTrial_LC_ENL1.vi"("input_dataTrial"=w1556, "input_spout"=w1561, "input_dataBlock"=w1554, "input_dataLC"=w1562, "input_dataCurrent"=w1558) -> ("output_LC__ENL1"=w1560:bool, "output_LC_led__ENL1"=w1559:bool, "output_dataTrial"=w1555:u16[][], "output_dataCurrent"=w1557:u16[])  [unwired: 3 in]
            }
            frame "initTrial_LC_Cue1" {
              n713 = call "myRIO_BRig_RT__Case_Exp_State_initTrial_LC_Cue1.vi"("input_dataTrial"=w1583, "input_spout"=w1586, "input_dataBlock"=w1581, "input_dataLC"=w1587, "input_dataCurrent"=w1585) -> ("output_LC__Cue1"=w1579:bool, "output_LC_led__Cue1"=w1580:bool, "output_dataTrial"=w1582:u16[][], "output_dataCurrent"=w1584:u16[])  [unwired: 3 in]
            }
            frame "ENL1_pre" {
              # "ENL1_n"
              # "Tcycle"
              # "counter"
              n714 = call "myRIO_BRig_RT_dataCurrent_Tcycle_generic.vi"() -> ("output_Tcycle_generic"=w1633:i32)  [unwired: 11 in]
              n715 = call "myRIO_BRig_RT_dataCurrent_count_generic.vi"() -> ("output_count_generic"=w1635:i32)  [unwired: 11 in]
              n716 = call "myRIO_BRig_RT_dataCurrent_ENL.vi"() -> ("output_ENL"=w1632:i32)  [unwired: 11 in]
              n717 = call "myRIO_BRig_RT_dataCurrent_ENL1_n.vi"() -> ("output_ENL1_n"=w1604:i32)  [unwired: 11 in]
              n718 = Index Array(array=w1626, index #1=w1632, index #2=w1604) -> (element #1=w1631:u16, element #2=w1603:u16)
              n719 = Increment(x=w1603) -> (x+1=w1602:u16)
              n720 = Replace Array Subset(array=w1626, new element #1=u16 0 ("new element/subarray"), index #1=w1635, new element #2=w1631, index #2=w1633, new element #3=w1602, index #3=w1604) -> (w1630:u16[])
              n721 = Select(t=myRIO_BRig_RT__Case_Exp_stateList."ENL1Penalty_pre" ("Enum"), s=w1614, f=myRIO_BRig_RT__Case_Exp_stateList."ENL1" ("Enum")) -> (s? t:f=w1611:T2)
            }
            frame "ENL1" {
              n722 = call "myRIO_BRig_RT__Case_Exp_State_ENL1.vi"("input_LC"=w1641, "I_lick"=w1646, "input_LC_led"=w1642, "input_state"=w1652, "input_dataCurrent"=w1651) -> ("output_trigger_laser_led"=w1640:bool, "output_state"=w1649:T2, "output_dataCurrent"=w1650:u16[], "output_trigger_laser"=w1639:bool)  [unwired: 3 in]
              n723 = Or(x=w1640, y=w1644) -> (x .or. y?=w1643:bool)
            }
            frame "ENL1Penalty_pre" {
              w1671 = FALSE
              # "Tcycle"
              # "counter"
              n724 = call "myRIO_BRig_RT_dataCurrent_Tcycle_generic.vi"() -> ("output_Tcycle_generic"=w1695:i32)  [unwired: 11 in]
              n725 = call "myRIO_BRig_RT_dataCurrent_count_generic.vi"() -> ("output_count_generic"=w1697:i32)  [unwired: 11 in]
              n726 = Select(t=w1671, s=w1673, f=w1674) -> (s? t:f=w1669:bool)
              n727 = Select(t=w1671, s=w1673, f=w1672) -> (s? t:f=w1670:bool)
              n728 = call "myRIO_BRig_RT_dataExp_ENL_penalty.vi"() -> ("output_ENL_penalty"=w1690:i32)  [unwired: 11 in]
              n729 = Index Array(array=w1691, index=w1690) -> (element=w1694:u16)
              n730 = Replace Array Subset(array=w1692, new element #1=u16 0 ("new element/subarray"), index #1=w1697, new element #2=w1694, index #2=w1695) -> (w1693:u16[])
            }
            frame "ENL1Penalty" {
              n731 = call "myRIO_BRig_RT__Case_Exp_State_ENL1Penalty.vi"("input_state"=w1720, "input_dataCurrent"=w1724) -> ("output_state"=w1721:T2, "output_dataCurrent"=w1723:u16[])  [unwired: 8 in]
            }
            frame "ENL2_pre" {
            }
            frame "ENL2" {
            }
            frame "ENL2Penalty_pre" {
            }
            frame "ENL2Penalty" {
            }
            frame "Cue1_pre" {
              # "Cue1_n"
              # "Tcycle_Cue1"
              # "0 = L, 1 = R, 2 = both"
              # "sp_R"
              # "sp_L"
              # "Tcycle"
              # "counter"
              n732 = Equal?(x=w1833, y=enum16{"Left", "Right"}."Left") -> (x = y?=w1832:bool)
              n733 = call "myRIO_BRig_RT_dataExp_Audio_sp__L.vi"() -> ("output_Audio_sp__L"=w1831:i32)  [unwired: 11 in]
              n734 = call "myRIO_BRig_RT_dataExp_Audio_sp__R.vi"() -> ("output_Audio_sp__R"=w1830:i32)  [unwired: 11 in]
              n735 = call "myRIO_BRig_RT_dataCurrent_Tcycle_generic.vi"() -> ("output_Tcycle_generic"=w1843:i32)  [unwired: 11 in]
              n736 = call "myRIO_BRig_RT_dataCurrent_count_generic.vi"() -> ("output_count_generic"=w1845:i32)  [unwired: 11 in]
              n737 = Select(t=w1831, s=w1832, f=w1830) -> (s? t:f=w1829:i32)
              n738 = call "myRIO_BRig_RT_dataCurrent_Cue1_n.vi"() -> ("output_Cue1_n"=w1807:i32)  [unwired: 11 in]
              n739 = call "myRIO_BRig_RT_dataCurrent_Tcycle_cue.vi"() -> ("output_Tcycle_cue"=w1816:i32)  [unwired: 11 in]
              n740 = Index Array(array=w1835, index=w1829) -> (element=w1827:u16)
              n741 = Index Array(array=w1817, index #1=w1816, index #2=w1807) -> (element #1=w1818:u16, element #2=w1809:u16)
              n742 = Increment(x=w1809) -> (x+1=w1808:u16)
              n743 = Not Equal To 0?(x=w1827) -> (x != 0?=w1825:bool)
              n744 = Not Equal?(x=w1827, y=u16 1) -> (x != y?=w1826:bool)
              n745 = Replace Array Subset(array=w1817, new element #1=u16 0 ("new element/subarray"), index #1=w1845, new element #2=w1818, index #2=w1843, new element #3=w1808, index #3=w1807) -> (w1842:u16[])
              n746 = Select(t=myRIO_BRig_RT__Case_Exp_stateList."Cue1Penalty_pre" ("Enum"), s=w1813, f=myRIO_BRig_RT__Case_Exp_stateList."Cue1" ("Enum")) -> (s? t:f=w1814:T2)
            }
            frame "Cue1" {
              n747 = call "myRIO_BRig_RT__Case_Exp_State_Cue1.vi"("input_LC"=w1853, "I_lick"=w1856, "input_LC_led"=w1854, "input_state"=w1858, "input_dataCurrent"=w1876) -> ("output_trigger_laser_led"=w1851:bool, "output_state"=w1857:T2, "output_dataCurrent"=w1875:u16[], "output_trigger_laser"=w1852:bool)  [unwired: 3 in]
              n748 = Or(x=w1851, y=w1850) -> (x .or. y?=w1849:bool)
              n749 = Equal?(x=myRIO_BRig_RT__Case_Exp_stateList."Selection_pre", y=w1857) -> (x = y?=w1861:bool)
              n750 = xnode "Read/Write Control"("FPGA VI Reference In"=w1860, "error in"=w1859, "SelectionState"=w1861) -> ()  [unwired: 2 out]
            }
            frame "Cue1Penalty_pre" {
              w1888 = FALSE
              # "Tcycle"
              # "counter"
              n751 = call "myRIO_BRig_RT_dataCurrent_Tcycle_generic.vi"() -> ("output_Tcycle_generic"=w1908:i32)  [unwired: 11 in]
              n752 = call "myRIO_BRig_RT_dataCurrent_count_generic.vi"() -> ("output_count_generic"=w1910:i32)  [unwired: 11 in]
              n753 = call "myRIO_BRig_RT_dataExp_Tcycle_CuePenalty.vi"() -> ("output_Tcycle_CuePenalty"=w1907:i32)  [unwired: 11 in]
              n754 = Select(t=w1888, s=w1883, f=w1887) -> (s? t:f=w1884:bool)
              n755 = Select(t=w1888, s=w1883, f=w1886) -> (s? t:f=w1885:bool)
              n756 = Index Array(array=w1902, index=w1907) -> (element=w1906:u16)
              n757 = Replace Array Subset(array=w1904, new element #1=u16 0 ("new element/subarray"), index #1=w1910, new element #2=w1906, index #2=w1908) -> (w1903:u16[])
            }
            frame "Cue1Penalty" {
              n758 = call "myRIO_BRig_RT__Case_Exp_State_Cue1Penalty.vi"("input_state"=w1934, "input_dataCurrent"=w1935) -> ("output_state"=w1932:T2, "output_dataCurrent"=w1933:u16[])  [unwired: 8 in]
            }
            frame "Cue2_pre" {
              n759 = call "myRIO_BRig_RT__Case_Exp_subState_LC__Cue2.vi"("input_spout"=w1952, "input_dataCurrent"=w1953, "input_dataLC"=w1951) -> ()  [unwired: 6 in, 2 out]
            }
            frame "Cue2" {
            }
            frame "Cue2Penalty_pre" {
            }
            frame "Cue2Penalty" {
            }
            frame "Selection_pre" {
              # "Tcycle"
              # "counter"
              n760 = xnode "Read/Write Control"("FPGA VI Reference In"=w2024, "error in"=w2025) -> ("error out"=→"error_Selection_pre":errorcluster, "SelectReward"=w2017:bool, "SelectWrong"=w2019:bool)  [unwired: 1 out]
              n761 = call "myRIO_BRig_RT_dataCurrent_Tcycle_generic.vi"() -> ("output_Tcycle_generic"=w2046:i32)  [unwired: 11 in]
              n762 = call "myRIO_BRig_RT_dataCurrent_count_generic.vi"() -> ("output_count_generic"=w2048:i32)  [unwired: 11 in]
              n763 = call "myRIO_BRig_RT_dataExp_Tcycle_Selection.vi"() -> ("output_Tcycle_Selection"=w2045:i32)  [unwired: 11 in]
              n764 = Index Array(array=w2042, index=w2045) -> (element=w2044:u16)
              n765 = Replace Array Subset(array=w2040, new element #1=u16 0 ("new element/subarray"), index #1=w2048, new element #2=w2044, index #2=w2046) -> (w2043:u16[])
              n766 = Or(x=w2017, y=w2019) -> (x .or. y?=w2018:bool)
              n767 = Select(t=myRIO_BRig_RT__Case_Exp_stateList."SelectReward_pre" ("Enum"), s=w2017, f=myRIO_BRig_RT__Case_Exp_stateList."SelectWrong_pre" ("Enum")) -> (s? t:f=w2023:T2)
              n768 = Select(t=w2023, s=w2018, f=myRIO_BRig_RT__Case_Exp_stateList."Selection" ("Enum")) -> (s? t:f=w2020:T2)
            }
            frame "Selection" {
              # "counter\nSelection"
              # "increment"
              # "get Tcycle"
              # "get count"
              n769 = xnode "Read/Write Control"("FPGA VI Reference In"=w2076, "error in"=w2075) -> ("FPGA VI Reference Out"=w2051:refnum<k20>, "error out"=w2052:errorcluster, "SelectReward"=w2072:bool, "SelectWrong"=w2073:bool)
              n770 = call "myRIO_BRig_RT_dataCurrent_Tcycle_generic.vi"() -> ("output_Tcycle_generic"=w2069:i32)  [unwired: 11 in]
              n771 = call "myRIO_BRig_RT_dataCurrent_count_generic.vi"() -> ("output_count_generic"=w2061:i32)  [unwired: 11 in]
              n772 = Index Array(array=w2070, index #1=w2069, index #2=w2061) -> (element #1=w2060:u16, element #2=w2068:u16)
              n773 = call "myRIO_BRig_RT__increment_u16.vi"() -> ("output_increment__u16"=w2067:u16)  [unwired: 11 in]
              n774 = Add(x=w2068, y=w2067) -> (x+y=w2062:u16)
              n775 = Greater?(x=w2060, y=w2062) -> (0:w2063:bool)
              n776 = Select(t=w2066, s=w2063, f=myRIO_BRig_RT__Case_Exp_stateList."SelectTimeout_pre" ("Enum")) -> (s? t:f=w2055:T2)
              n777 = Select(t=w2062, s=w2063, f=w2060) -> (s? t:f=w2058:u16)
              n778 = call "myRIO_BRig_RT_dataCurrent_count_selection.vi"() -> ("output_count_generic"=w2059:i32)  [unwired: 11 in]
              n779 = Select(t=myRIO_BRig_RT__Case_Exp_stateList."SelectReward_pre" ("Enum"), s=w2072, f=myRIO_BRig_RT__Case_Exp_stateList."SelectWrong_pre" ("Enum")) -> (s? t:f=w2071:T2)
              n780 = Replace Array Subset(array=w2070, new element #1=w2058, index #1=w2061, new element #2=w2058, index #2=w2059) -> (w2065:u16[])
              n781 = Or(x=w2072, y=w2073) -> (x .or. y?=w2054:bool)
              n782 = Not(x=w2054) -> (.not. x?=w2053:bool)
              n783 = xnode "Read/Write Control"("FPGA VI Reference In"=w2051, "error in"=w2052, "SelectionState"=w2053) -> ("error out"=→"error_Selection":errorcluster)  [unwired: 1 out]
              n784 = Select(t=w2071, s=w2054, f=w2055) -> (s? t:f=w2074:T2)
            }
            frame "SelectReward_pre" {
              # "iState"
              # "Tcycle\nReward"
              # "nRewTrials"
              # "Tcycle\nGeneric"
              # "counter"
              n785 = call "myRIO_BRig_RT_dataCurrent_nRewTrials.vi"() -> ("output_nRewTrials"=w2108:i32)  [unwired: 11 in]
              n786 = Equal?(x=w2117, y=enum16{"Left", "Right"}."Left") -> (x = y?=w2118:bool)
              n787 = Index Array(array=w2109, index=w2108) -> (element=w2107:u16)
              n788 = call "myRIO_BRig_RT_dataExp_Tcycle_Reward__L.vi"() -> ("output_Tcycle_Reward__L"=w2121:i32)  [unwired: 11 in]
              n789 = call "myRIO_BRig_RT_dataExp_Tcycle_Reward__R.vi"() -> ("output_Tcycle_Reward__R"=w2122:i32)  [unwired: 11 in]
              n790 = Increment(x=w2107) -> (x+1=w2106:u16)
              n791 = Select(t=w2121, s=w2118, f=w2122) -> (s? t:f=w2120:i32)
              n792 = call "myRIO_BRig_RT__Case_Exp_subState_LC__Reward.vi"("input_spout"=w2117, "input_dataCurrent"=w2109, "input_dataLC"=w2116) -> ()  [unwired: 6 in, 2 out]
              n793 = call "myRIO_BRig_RT_dataCurrent_count_generic.vi"() -> ("output_count_generic"=w2111:i32)  [unwired: 11 in]
              n794 = call "myRIO_BRig_RT_dataCurrent_Tcycle_generic.vi"() -> ("output_Tcycle_generic"=w2112:i32)  [unwired: 11 in]
              n795 = Index Array(array=w2123, index=w2120) -> (element=w2113:u16)
              n796 = call "myRIO_BRig_RT_dataCurrent_iState.vi"() -> ("output_iState"=w2101:i32)  [unwired: 11 in]
              n797 = Replace Array Subset(array=w2109, new element #1=w2106, index #1=w2108, new element #2=u16 0 ("new element/subarray"), index #2=w2111, new element #3=w2113, index #3=w2112, new element #4=u16 1 ("new element/subarray"), index #4=w2101) -> (w2124:u16[])
            }
            frame "SelectReward" {
              n798 = call "myRIO_BRig_RT__Case_Exp_State_Reward.vi"("input_dataCurrent"=w2146, "input_state"=w2143, "input_spout"=w2140, "input_LC"=w2141, "input_dataLC"=w2142) -> ("output_dataCurrent"=w2145:u16[], "output_state"=w2144:T2, "output__L"=w2138:bool, "output__R"=w2139:bool)  [unwired: 6 in, 1 out]
            }
            frame "SelectRewardPost_pre" {
              # "nRewards"
              # "nRewTrials"
              # "Tcycle"
              # "counter"
              n799 = call "myRIO_BRig_RT_dataBlock_nRewards__L.vi"() -> ("output_nRewards__L"=w2162:i32)  [unwired: 11 in]
              n800 = call "myRIO_BRig_RT_dataBlock_nRewards__R.vi"() -> ("output_nRewards__R"=w2161:i32)  [unwired: 11 in]
              n801 = call "myRIO_BRig_RT_dataCurrent_Tcycle_generic.vi"() -> ("output_Tcycle_generic"=w2181:i32)  [unwired: 11 in]
              n802 = call "myRIO_BRig_RT_dataCurrent_count_generic.vi"() -> ("output_count_generic"=w2183:i32)  [unwired: 11 in]
              n803 = case shown="\"Left\", Default" w2155 {
                tunnel: w2167 -> [w2188 w2192]
                tunnel: [w2187 w2192] -> w2166
                tunnel: [w2189 w2190] -> w2165
                tunnel: w2164 -> [w2189 w2191]
                frame "Left", Default {
                  n804 = Increment(x=w2188) -> (x+1=w2187:u16)
                }
                frame "Right" {
                  n805 = Increment(x=w2191) -> (x+1=w2190:u16)
                }
              }
              "nRewards_Left" <- w2166
              "nRewards_Right" <- w2165
              n806 = Equal?(x=w2155, y=enum16{"Left", "Right"}."Left") -> (x = y?=w2154:bool)
              n807 = Select(t=w2162, s=w2154, f=w2161) -> (s? t:f=w2160:i32)
              n808 = call "myRIO_BRig_RT_dataExp_Tcycle_RewardPost.vi"() -> ("output_Tcycle_RewardPost"=w2177:i32)  [unwired: 11 in]
              n809 = call "myRIO_BRig_RT_dataCurrent_nRewTrials.vi"() -> ("output_nRewTrials"=w2163:i32)  [unwired: 11 in]
              n810 = Index Array(array=w2178, index=w2177) -> (element=w2180:u16)
              n811 = Index Array(array=w2157, index=w2163) -> (element=w2152:u16)
              n812 = Replace Array Subset(array=w2157, new element #1=u16 0 ("new element/subarray"), index #1=w2183, new element #2=w2180, index #2=w2181) -> (w2179:u16[])
              n813 = Replace Array Subset(array=w2159, new element=w2152, index (row)=w2153, index (col)=w2160) -> (w2158:u16[][])
              n814 = local write "nRewards_cur"(w2152) -> ()
            }
            frame "SelectRewardPost" {
              n815 = call "myRIO_BRig_RT__Case_Exp_State_RewardPost.vi"("input_state"=w2207, "input_dataCurrent"=w2210) -> ("output_state"=w2208:T2, "output_dataCurrent"=w2209:u16[])  [unwired: 8 in]
            }
            frame "SelectWrong_pre" {
              # "iState"
              # "Tcycle"
              # "counter"
              n816 = call "myRIO_BRig_RT_dataCurrent_Tcycle_generic.vi"() -> ("output_Tcycle_generic"=w2235:i32)  [unwired: 11 in]
              n817 = call "myRIO_BRig_RT_dataCurrent_count_generic.vi"() -> ("output_count_generic"=w2237:i32)  [unwired: 11 in]
              n818 = call "myRIO_BRig_RT_dataExp_Tcycle_Wrong.vi"() -> ("output_Tcycle_Wrong"=w2233:i32)  [unwired: 11 in]
              n819 = call "myRIO_BRig_RT__Case_Exp_subState_LC__Wrong.vi"("input_spout"=w2229, "input_dataCurrent"=w2230, "input_dataLC"=w2227) -> ()  [unwired: 6 in, 2 out]
              n820 = Index Array(array=w2231, index=w2233) -> (element=w2234:u16)
              n821 = call "myRIO_BRig_RT_dataCurrent_iState.vi"() -> ("output_iState"=w2221:i32)  [unwired: 11 in]
              n822 = Replace Array Subset(array=w2230, new element #1=u16 0 ("new element/subarray"), index #1=w2237, new element #2=w2234, index #2=w2235, new element #3=u16 2 ("new element/subarray"), index #3=w2221) -> (w2232:u16[])
            }
            frame "SelectWrong" {
              n823 = call "myRIO_BRig_RT__Case_Exp_State_Wrong.vi"("input_dataLC"=w2258, "input_LC"=w2257, "input_state"=w2251, "input_dataCurrent"=w2261) -> ("output_state"=w2248:T2, "output_dataCurrent"=w2260:u16[])  [unwired: 5 in, 1 out]
              n824 = Not Equal?(x=w2251, y=w2248) -> (x != y?=w2250:bool)
              n825 = Select(t=myRIO_BRig_RT__Case_Exp_stateList."SelectWrong_post" ("Enum"), s=w2250, f=w2248) -> (s? t:f=w2247:T2)
            }
            frame "SelectWrong_post" {
            }
            frame "SelectTimeout_pre" {
              # "iState"
              # "Tcycle"
              # "counter"
              n826 = call "myRIO_BRig_RT_dataCurrent_Tcycle_generic.vi"() -> ("output_Tcycle_generic"=w2306:i32)  [unwired: 11 in]
              n827 = call "myRIO_BRig_RT_dataCurrent_count_generic.vi"() -> ("output_count_generic"=w2304:i32)  [unwired: 11 in]
              n828 = call "myRIO_BRig_RT_dataExp_Tcycle_Timeout.vi"() -> ("output_Tcycle_Timeout"=w2308:i32)  [unwired: 11 in]
              n829 = call "myRIO_BRig_RT__Case_Exp_subState_LC__Timeout.vi"("input_spout"=w2299, "input_dataCurrent"=w2300, "input_dataLC"=w2298) -> ()  [unwired: 6 in, 2 out]
              n830 = Index Array(array=w2302, index=w2308) -> (element=w2307:u16)
              n831 = call "myRIO_BRig_RT_dataCurrent_iState.vi"() -> ("output_iState"=w2292:i32)  [unwired: 11 in]
              n832 = Replace Array Subset(array=w2300, new element #1=u16 0 ("new element/subarray"), index #1=w2304, new element #2=w2307, index #2=w2306, new element #3=u16 3 ("new element/subarray"), index #3=w2292) -> (w2303:u16[])
            }
            frame "SelectTimeout" {
              n833 = call "myRIO_BRig_RT__Case_Exp_State_Timeout.vi"("input_dataLC"=w2327, "input_LC"=w2328, "input_state"=w2318, "input_dataCurrent"=w2333) -> ("output_state"=w2319:T2, "output_dataCurrent"=w2332:u16[])  [unwired: 5 in, 1 out]
              n834 = Not Equal?(x=w2318, y=w2319) -> (x != y?=w2322:bool)
              n835 = Select(t=myRIO_BRig_RT__Case_Exp_stateList."SelectTimeout_post" ("Enum"), s=w2322, f=w2319) -> (s? t:f=w2320:T2)
            }
            frame "SelectTimeout_post" {
            }
            frame "endTrial1" {
              # "Update dataBlock"
              n836 = call "myRIO_BRig_RT__Case_Exp_State_endTrial1.vi"("input_spout"=w2366, "input_dataBlock"=w2365, "input_dataCurrent"=w2363) -> ("output_dataBlock"=w2364:u16[][], "output_dataCurrent"=w2362:u16[])  [unwired: 7 in]
            }
            frame "endTrial2" {
              # "update dataTrial"
              n837 = call "myRIO_BRig_RT__Case_Exp_State_endTrial2.vi"("input_spout"=w2385, "input_dataTrial"=w2389, "input_dataCurrent"=w2387) -> ("output_dataTrial"=w2388:u16[][], "output_dataCurrent"=w2386:u16[])  [unwired: 7 in]
            }
            frame "endTrial3" {
              w2411 = myRIO_BRig_RT__Case_Exp_stateList."endBlock" ("Enum")
              # "nRewTrials"
              # "iTrial"
              # "I_blockUntilReward"
              # "TPB"
              # "end block?"
              n838 = local read "STOP_endTrial"() -> (w2409:bool)
              n839 = local read "STOP_abort"() -> (w2408:bool)
              n840 = local read "START"() -> (w2406:bool)
              n841 = call "myRIO_BRig_RT_dataExp_IblockUntilReward.vi"() -> ("output_I_blockUntilReward"=w2418:i32)  [unwired: 11 in]
              n842 = Index Array(array=w2402, index=w2418) -> (element=w2398:u16)
              n843 = Not(x=w2406) -> (.not. x?=w2407:bool)
              n844 = Not Equal To 0?(x=w2398) -> (x != 0?=w2416:bool)
              n845 = Compound Arithmetic op=OR(w2409, w2407, w2408) -> (w2410:bool)
              n846 = call "myRIO_BRig_RT_dataCurrent_nRewTrials.vi"() -> ("output_nRewTrials"=w2414:i32)  [unwired: 11 in]
              n847 = call "myRIO_BRig_RT_dataCurrent_iTrial.vi"() -> ("output_iTrial"=w2415:i32)  [unwired: 11 in]
              n848 = Select(t=w2414, s=w2416, f=w2415) -> (s? t:f=w2413:i32)
              n849 = call "myRIO_BRig_RT_dataCurrent_TpB.vi"() -> ("output_TpB"=w2417:i32)  [unwired: 11 in]
              n850 = Index Array(array=w2403, index #1=w2417, index #2=w2413) -> (element #1=w2404:u16, element #2=w2405:u16)
              n851 = Less Or Equal?(x=w2404, y=w2405) -> (x <= y?=w2401:bool)
              n852 = Select(t=w2411, s=w2401, f=myRIO_BRig_RT__Case_Exp_stateList."initTrial" ("Enum")) -> (s? t:f=w2412:T2)
              n853 = Select(t=w2411, s=w2410, f=w2412) -> (s? t:f=w2399:T2)
            }
            frame "endBlock" {
              # "R"
              # "L"
              # "idxDataBlock"
              n854 = Equal?(x=w2442, y=enum16{"Left", "Right"}."Left") -> (x = y?=w2441:bool)
              n855 = call "myRIO_BRig_RT_dataCurrent_idxDataBlockL.vi"() -> ("output_idxDataBlock__L"=w2445:i32)  [unwired: 11 in]
              n856 = call "myRIO_BRig_RT_dataCurrent_idxDataBlockR.vi"() -> ("output_idxDataBlock__R"=w2444:i32)  [unwired: 11 in]
              n857 = Increment(x=w2436) -> (x+1=w2435:i32)
              n858 = Select(t=w2445, s=w2441, f=w2444) -> (s? t:f=w2439:i32)
              n859 = To Unsigned Word Integer(number=w2435) -> (unsigned 16bit integer=w2437:u16)
              n860 = local read "START"() -> (w2465:bool)
              n861 = local read "STOP_endBlock"() -> (w2460:bool)
              n862 = local read "STOP_endTrial"() -> (w2463:bool)
              n863 = local read "STOP_abort"() -> (w2462:bool)
              n864 = Replace Array Subset(array=w2440, new element=w2437, index=w2439) -> (w2438:u16[])
              n865 = Not(x=w2465) -> (.not. x?=w2464:bool)
              n866 = Compound Arithmetic op=OR(w2464, w2460, w2463, w2462) -> (w2461:bool)
              n867 = Select(t=myRIO_BRig_RT__Case_Exp_stateList."endExp" ("Enum"), s=w2461, f=myRIO_BRig_RT__Case_Exp_stateList."initBlock" ("Enum")) -> (s? t:f=w2469:T2)
            }
            frame "endExp" {
            }
            frame "commConnect" {
              n868 = call "myRIO_BRig_RT_comm_webdav_connect.vi"("input_password"="Host Password", "input_username"="Host UserName") -> ("output_Iconnected"=w2490:bool, "output_hSession"=w2508:T6)  [unwired: 7 in, 1 out]
              "Connected To Host?" <- w2490
              n869 = case shown="False" w2490 {
                frame False {
                  n870 = One Button Dialog(message="Connection Failed!\nData not being saved!") -> ()  [unwired: 1 in, 1 out]
                }
                frame True {
                }
              }
            }
            frame "commUpload_pre" {
              n871 = Select(t=myRIO_BRig_RT__Case_Exp_stateList."commUpload_dataBlock" ("Enum"), s=w2515, f=myRIO_BRig_RT__Case_Exp_stateList."endTrial3") -> (s? t:f=w2513:T2)
            }
            frame "commUpload_dataBlock" {
              n872 = call "myRIO_BRig_RT_comm_webdav_uploadFile__data.vi"("input_fileName_prefix"=w2536, "input_fileName"="dataBlock" ("input_filename"), "input_hSession"=w2538) -> ()  [unwired: 8 in, 1 out]
            }
            frame "commUpload_dataCurrent" {
              n873 = call "myRIO_BRig_RT_comm_webdav_uploadFile__data.vi"("input_fileName_prefix"=w2557, "input_fileName"="dataCurrent" ("input_filename"), "input_hSession"=w2559) -> ()  [unwired: 8 in, 1 out]
            }
            frame "commUpload_dataExp" {
              n874 = call "myRIO_BRig_RT_comm_webdav_uploadFile__data.vi"("input_fileName_prefix"=w2578, "input_fileName"="dataExp" ("input_filename"), "input_hSession"=w2580) -> ()  [unwired: 8 in, 1 out]
            }
            frame "commUpload_dataLC" {
              n875 = call "myRIO_BRig_RT_comm_webdav_uploadFile__data.vi"("input_fileName_prefix"=w2599, "input_fileName"="dataLC" ("input_filename"), "input_hSession"=w2601) -> ()  [unwired: 8 in, 1 out]
            }
            frame "commUpload_dataTrial" {
              n876 = call "myRIO_BRig_RT_comm_webdav_uploadFile__data.vi"("input_fileName_prefix"=w2623, "input_fileName"="dataTrial" ("input_filename"), "input_hSession"=w2625) -> ()  [unwired: 8 in, 1 out]
            }
            frame "saveData_dataBlock" {
              # "idxDataBlockR"
              # "idxDataBlockL"
              n877 = call "myRIO_BRig_RT_dataCurrent_idxDataBlockL.vi"() -> ("output_idxDataBlock__L"=w2649:i32)  [unwired: 11 in]
              n878 = call "myRIO_BRig_RT_dataCurrent_idxDataBlockR.vi"() -> ("output_idxDataBlock__R"=w2650:i32)  [unwired: 11 in]
              n879 = Index Array(array=w2651, index #1=w2649, index #2=w2650) -> (element #1=w2648:u16, element #2=w2647:u16)
              n880 = Greater?(x=w2648, y=w2647) -> (0:w2646:bool)
              n881 = Select(t=w2648, s=w2646, f=w2647) -> (s? t:f=w2644:u16)
              n882 = Increment(x=w2644) -> (x+1=w2643:u16)
              n883 = To Long Integer(number=w2643) -> (32bit integer=w2642:i32)
              n884 = Array Subset(array=w2645, length (row)=w2642) -> (w2641:u16[][])  [unwired: 3 in]
              n885 = call "myRIO_BRig_RT_comm_webdav_saveArrayToFile__2D_u16.vi"("Array"=w2641, "input_filename"="dataBlock") -> ()  [unwired: 10 in]
            }
            frame "saveData_dataCurrent" {
              n886 = call "myRIO_BRig_RT_comm_webdav_saveArrayToFile__1D_u16.vi"("Array"=w2670, "input_filename"="dataCurrent") -> ()  [unwired: 10 in]
            }
            frame "saveData_dataExp" {
              # "runTime"
              n887 = Get Date/Time In Seconds() -> (seconds since 1Jan1904=w2698:timestamp)
              n888 = To Double Precision Float(number=w2698) -> (double precision float=w2697:dbl)
              n889 = call "myRIO_BRig_RT_dataExp_runTime_seconds.vi"() -> ("output_RunTime_minutes"=w2696:i32)  [unwired: 11 in]
              n890 = Subtract(x=w2697, y=w2695) -> (x-y=w2692:dbl)
              n891 = To Unsigned Word Integer(number=w2692) -> (unsigned 16bit integer=w2691:u16)
              n892 = Replace Array Subset(array=w2690, new element=w2691, index=w2696) -> (w2693:u16[])
              n893 = call "myRIO_BRig_RT_comm_webdav_saveArrayToFile__1D_u16.vi"("Array"=w2693, "input_filename"="dataExp") -> ()  [unwired: 10 in]
            }
            frame "saveData_dataLC" {
              n894 = call "myRIO_BRig_RT_comm_webdav_saveArrayToFile__1D_u16.vi"("Array"=w2717, "input_filename"="dataLC") -> ()  [unwired: 10 in]
            }
            frame "saveData_dataTrial" {
              # "idxTrial"
              n895 = call "myRIO_BRig_RT_dataCurrent_idxDataTrial.vi"() -> ("output_idxDataTrial"=w2742:i32)  [unwired: 11 in]
              n896 = Index Array(array=w2743, index=w2742) -> (element=w2739:u16)
              n897 = Increment(x=w2739) -> (x+1=w2738:u16)
              n898 = To Long Integer(number=w2738) -> (32bit integer=w2737:i32)
              n899 = Array Subset(array=w2740, length (row)=w2737) -> (w2741:u16[][])  [unwired: 3 in]
              n900 = call "myRIO_BRig_RT_comm_webdav_saveArrayToFile__2D_u16.vi"("Array"=w2741, "input_filename"="dataTrial") -> ()  [unwired: 10 in]
            }
          }
          n901 = case shown="True" w1032 {
            tunnel: w1028 -> [w1055 w1063]
            tunnel: w1031 -> [_ w1059]
            tunnel: w1030 -> [_ w1058]
            tunnel: w1029 -> [_ w1057]
            tunnel: w998 -> [_ w1056]
            tunnel: [w1055 w1062] -> w1027
            tunnel: w1026 -> [w1054 w1061]
            tunnel: [w1054 w1060] -> w1025
            frame False {
            }
            frame True {
              n902 = call "myRIO_BRig_RT__Case_Exp__recordLick.vi"("intput_state__trialEnd"=w1056, "intput_state__trialStart"=w1057, "input_lick__R"=w1058, "input_lick__L"=w1059, "input_dataCurrent"=w1061, "input_dataLick"=w1063) -> ("output_dataCurrent"=w1060:u16[], "output_dataLick"=w1062:u16[][])  [unwired: 4 in]
            }
          }
          n903 = Or(x=w1000, y=w1001) -> (x .or. y?=w987:bool)
          n904 = Or(x=w1004, y=w984) -> (x .or. y?=w973:bool)
          n905 = Or(x=w983, y=w1005) -> (x .or. y?=w999:bool)
          n906 = Or(x=w1003, y=w1002) -> (x .or. y?=w988:bool)
          n907 = Or(x=w1033, y="STOP_abort") -> (x .or. y?=w1035:bool)
          n908 = Or(x=w961, y=w962) -> (x .or. y?=w959:bool)
          n909 = Or(x=w963, y=w962) -> (x .or. y?=w960:bool)
          n910 = xnode "Read/Write Control"("FPGA VI Reference In"=w975, "error in"=w974, "A1_SR"=w988, "A3_SL"=w987, "A6_Act"=w972, "audioTrigger_L"=w973, "audioAmp_L"=w1014, "audioFreq_L_Hz"=w982, "audioTrigger_R"=w999, "audioAmp_R"=w1015, "audioFreq_R_Hz"=w1016, "laserledMTrig"=w959, "laserMTrig"=w960) -> ("FPGA VI Reference Out"=w1024:refnum<k20>, "error out"=w1023:errorcluster)
          n911 = node-c288() -> ()  [unwired: 1 in, 1 out]
          "cState" <- w1029
        }
        n912 = node-c288(w919) -> ()  [unwired: 1 out]
        n913 = flat-sequence {
          tunnel: w915 -> [w951]
          tunnel: w914 -> [w950]
          tunnel: [w949] -> w907
          tunnel: [w948] -> w906
          tunnel: [w955] -> w908
          tunnel: [w956] -> w913
          tunnel: w907 -> [w956]
          tunnel: w906 -> [w955]
          frame #0 {
            w952 = u16 0 ("AudioLeft_phase_inc")
            w947 = FALSE
            n914 = xnode "Read/Write Control"("FPGA VI Reference In"=w951, "error in"=w950, "Counts_Reset"=TRUE, "audioTrigger_L"=w947, "audioFreq_L_Hz"=w952, "audioAmp_L"=w952, "audioTrigger_R"=w947, "audioFreq_R_Hz"=w952, "audioAmp_R"=w952, "A3_SL"=w947, "A1_SR"=w947, "A6_Act"=w947) -> ("FPGA VI Reference Out"=w949:refnum<k20>, "error out"=w948:errorcluster)
          }
          frame #1 {
            w954 = FALSE ("START")
            n915 = local write "START"(w954) -> ()
            n916 = local write "STOP_endTrial"(w954) -> ()
            n917 = local write "STOP_endBlock"(w954) -> ()
          }
        }
        n918 = stacked-sequence {
          tunnel: w891 -> [w927 _]
          tunnel: w889 -> [w928 _]
          tunnel: w888 -> [_ w933]
          tunnel: w887 -> [_ w932]
          tunnel: w886 -> [_ w931]
          tunnel: w885 -> [w921 _]
          frame #0 {
            n919 = call "myRIO_BRig_RT_dataCurrent_idxDataLick.vi"() -> ("output_idxDataLick"=w922:i32)  [unwired: 11 in]
            n920 = Index Array(array=w921, index=w922) -> (element=w924:u16)
            n921 = Increment(x=w924) -> (x+1=w925:u16)
            n922 = call "myRIO_BRig_RT_comm_webdav_saveArrayToFile__1D_u16.vi"("Array"=w928, "input_filename"="dataMTrig") -> ()  [unwired: 10 in]
            n923 = To Long Integer(number=w925) -> (32bit integer=w923:i32)
            n924 = Array Subset(array=w927, length (row)=w923) -> (w926:u16[][])  [unwired: 3 in]
            n925 = call "myRIO_BRig_RT_comm_webdav_saveArrayToFile__2D_u16.vi"("Array"=w926, "input_filename"="dataLick") -> ()  [unwired: 10 in]
          }
          frame #1 {
            n926 = case shown="True" w933 {
              tunnel: w932 -> [_ w935]
              tunnel: w931 -> [_ w934]
              frame False {
              }
              frame True {
                n927 = stacked-sequence {
                  tunnel: w935 -> [w937 w944 w946]
                  tunnel: w934 -> [w938 w943 _]
                  frame #0 {
                    n928 = call "myRIO_BRig_RT_comm_webdav_uploadFile__announce.vi"("input_addText"=TRUE, "input_fileName_prefix"=w938, "intput_fileName"="curExp_end", "intput_hSession"=w937) -> ("output_Isuccess"=w936:bool)  [unwired: 6 in, 1 out]
                    n929 = case shown="True" w936 {
                      frame False {
                        n930 = One Button Dialog(message="!!! Warning !!! Your data is located at C:\\BehaviorRig\\commTransfer") -> ()  [unwired: 1 in, 1 out]
                      }
                      frame True {
                        n931 = Wait (ms)(milliseconds to wait=u32 20) -> ()  [unwired: 1 out]
                      }
                    }
                  }
                  frame #1 {
                    n932 = call "myRIO_BRig_RT__endExp_sendData.vi"("input_fileName_prefix"=w943, "input_hSession"=w944) -> ()  [unwired: 8 in, 2 out]
                  }
                  frame #2 {
                    n933 = local write "Connected To Host?"(FALSE ("Connected To Host?")) -> ()
                    n934 = call <vilib>:"Close Session.vi"("session handle"=w946) -> ()  [unwired: 14 in, 1 out]
                  }
                }
              }
            }
          }
        }
      }
    }
    n935 = local read "STOP_abort"() -> (w30:bool)
  }
  n936 = xnode "Read/Write Control"("FPGA VI Reference In"=w8, "error in"=w7, "FPGA_Stop"=TRUE) -> ("FPGA VI Reference Out"=w13:refnum<k20>, "error out"=w14:errorcluster)
  n937 = xnode "Close FPGA VI Reference"("FPGA VI Reference In"=w13, "error in"=w14) -> ("error out"=w12:errorcluster)
  n938 = call <vilib>:"Reset myRIO.vi"("error in (no error)"=w12) -> ()  [unwired: 10 in, 1 out]
